vi "AbelFcsMain.vi"() -> ()   [LabVIEW 2011]
uses:
  <vilib>/FPGAPlugInAG/PCIe-7852R/niLvFpga_Open_PCIe-7852R.vi
  <vilib>/rvi/interface/common/dynamic/niFpgaDynamicAddResources.vi
  <vilib>/Utility/error.llb/Error Cluster From Error Code.vi
  <vilib>/FPGAPlugInAG/Dynamic/niLvFpga_Run_Dynamic.vi
  <vilib>/RVI Host/nirviSupport.llb/nirviErrorClusterFromErrorCode.vi
  <vilib>/rvi/errors/niLvFpgaAdjustHostInterfaceError.vi
  <vilib>/DAQmx/create/channels.llb/DAQmx Create Channel (CO-Pulse Generation-Frequency).vi
  <vilib>/FPGAPlugInAG/Dynamic/niLvFpga_Reset_Dynamic.vi
  <vilib>/FPGAPlugInAG/Dynamic/niLvFpga_Close_Dynamic.vi
  <vilib>/rvi/interface/nirviOpenFPGA/nirviOpenFPGA.xnode
  FPGA Bitfiles/AbelFcsProject_FPGATarget_FPGAABELKalman_643775DA.lvbitx
  ABEL-Trap/FPGA_ABEL_Kalman.vi
  <vilib>/rvi/interface/nirviMethod/nirviMethod.xnode
  <vilib>/rvi/interface/nirviCloseFPGA/nirviCloseFPGA.xnode
  <vilib>/FPGAPlugInAG/Dynamic/niLvFpga_ConfigureFifo_Dynamic.vi
  <vilib>/rvi/errors/niLvFpgaMergeErrorWithErrorCode.vi
  <vilib>/FPGAPlugInAG/Dynamic/niLvFpga_StartFifo_Dynamic.vi
  <vilib>/FPGAPlugInAG/Dynamic/niLvFpga_ReadFifo_Dynamic.vi
  <vilib>/Analysis/NI_AALBase.lvlib
  <vilib>/FPGAPlugInAG/Dynamic/niLvFpga_WriteFifo_Dynamic.vi
  <vilib>/rvi/interface/nirviMethod/StockFPGA_InlinedMethodWaitForMultipleIRQ.vi
  <vilib>/FPGAPlugInAG/Dynamic/niLvFpga_WaitOnIrq_Dynamic.vi
  <vilib>/FPGAPlugInAG/Dynamic/niLvFpga_AcknowledgeIrq_Dynamic.vi
panel:
  out "X Steps":dbl
  out "FCS Point Measurement 2":bool
  out "Abeltrapping (EodScan) 2":bool
  out "3dAbelFcs":bool=TRUE
  out "Y Steps":dbl
  out "Z Steps":dbl
  out "concatenated string":string
  out "20Mhz":bool
  out "80Mhz":bool
  in  "Main Control":enum32{"Main", "Trapping"}(tab)
  in  "Stop Program":bool
  in  "SCANNER EMERGENCY":bool
  out "Task":T1(ring)
  in  "Trap":bool
  out "Current Modulation Voltages":dbl[][](array[numeric])
  out "Current Voltages":dbl[][](array[numeric])
  out "Global Stop":bool=TRUE
  out "Stop Measurement":bool
  in  "DeviceTabs":T2(tab)
  in  "WS File Tree":string(tree)
  out "Workspace":path=path "X:/MTusers/Christoph/2011-02-01 Andi/2011-02-01.msw"
  in  "New MSW":bool
  in  "Open MSW":bool
  in  "Sample description":string
  in  "Save Files":bool=TRUE
  out "Last Image File No":i32=-1
  in  "Prefix":string
  in  "Get Position":bool
  in  "Move Stage":bool
  in  "X-Position":dbl=48.0021 caption="X" min=0.0 max=200.0 step=0.1 format="%1.3f um"
  in  "Y-Position":dbl=19.9997 caption="Y" min=0.0 max=200.0 step=0.1 format="%1.3f um"
  in  "Z-Position":dbl=69.999 caption="Z" min=0.0 max=200.0 step=0.1 format="%1.3f um"
  out "x-position":dbl format="%.3f"
  out "y-position":dbl format="%.3f"
  out "z-position":dbl format="%.3f"
  in  "Power Button":bool
  in  "Power":dbl(knob)=100.0 min=0.0 max=100.0 step=5.0 scale=0.0..100.0 scale format="%#_3g"
  out "Laser Connected":bool
  out "Laser ready":bool
  out "Time to go":i32
  in  "Laser  Profile":string="1"
  in  "CFD Settings":T3={"Sync Level"=15, "Sync ZeroX"=0, "Sync Offset"=0, "Chan Settings"=[{"CHx Level"=50, "CHx ZeroX"=10, "CHx Offset"=-22150}, {"CHx Level"=50, "CHx ZeroX"=10, "CHx Offset"=-21850}, {"CHx Level"=75, "CHx ZeroX"=10, "CHx Offset"=-6000}, {"CHx Level"=75, "CHx ZeroX"=10, "CHx Offset"=-5700}]}
  in  "Auto Exposure::Mode":u32(ring) items=["Relative"=0, "Ignored"=5]
  in  "Brightness::Mode":u32(ring) items=["Relative"=0, "Ignored"=5]
  in  "Gain::Mode":u32(ring) items=["Absolute"=1, "Auto"=3, "Relative"=0, "Ignored"=5]
  in  "Gamma::Mode":u32(ring)=2 items=["Relative"=0, "Off"=2, "Ignored"=5]
  in  "Shutter::Mode":u32(ring) items=["Auto"=3, "Relative"=0, "Ignored"=5]
  in  "Trigger::Trigger Activation":u32(ring) items=["Level Low", "Level High"]
  in  "Trigger::Trigger Mode":u32(ring)=16 items=["Mode 0"=0, "Mode 1"=1, "Mode 15"=15, "Off"=16]
  in  "Trigger Delay::Mode":u32(ring)=2 items=["Absolute"=1, "Relative"=0, "Off"=2, "Ignored"=5]
  in  "Brightness::Value":dbl=16.0 min=0.0 max=1023.0 step=1.0
  in  "Shutter::Value":dbl=436.0 min=1.0 max=4095.0 step=1.0
  in  "Auto Exposure::Value":dbl=125.0 min=50.0 max=205.0 step=1.0
  in  "Gain::Value":dbl min=0.0 max=680.0 step=1.0
  in  "Trigger::Trigger Parameter":u32 max=0
  in  "is on?":bool
  out "error out":errorcluster
  in  "PI SystemNumber":i32=1
  in  "Image Measurent Parameters":T4
  in  "Measurement Tab Control":T5(tab)
  in  "Adjustment":bool
  in  "Move into solution":bool=TRUE
  in  "Laser pulse duration":i32[](array[numeric]) min=2 max=100000 step=1 format="%d µs"
  in  "Measurement Time":i32=60 min=10 format="%.0d s"
  in  "Point Measurement":bool
  out "Counts":u32[](array[numeric])
  in  "Line Scan":bool
  in  "Grid Measurement":bool
  in  "Z-Axis Offset":dbl=2.0 min=0.1 max=10.0
  in  "Y-Axis Offset":dbl=2.0 min=0.1 max=10.0
  in  "X-Axis Offset":dbl=2.0 min=0.1 max=10.0
  in  "Z-Axis Points":u16=1 min=1 max=100
  in  "Y-Axis Points":u16=50 min=1 max=100
  in  "X-Axis Points":u16=50 min=1 max=100
  out "Grid Points":dbl[][](array[numeric])
  in  "Axis":enum32{"x-y", "x-z", "y-x", "y-z", "z-x", "z-y"}(ring)
  in  "Picture size 2":dbl=50.0 min=0.1 max=200.0 format="%1.1f um"
  in  "Picture size":dbl=50.0 min=0.1 max=200.0 format="%1.1f um"
  in  "Pixel time":dbl=1.0 min=0.1 max=10.0 step=0.1 format="%.1f ms"
  in  "Resolution":dbl=1.0 min=0.05 max=10.0 step=0.05 format="%.2f µm"
  out "Measure. time":dbl format="%7.1f s"
  in  "Aquire Image":bool
  out "y":i16=500
  out "x":i16=500
  in  "Trapping Tab Control":T6(tab)
  in  "Clear Warnings":bool
  in  "Record":bool
  in  "Estimate Trap Time":bool
  in  "Update FPGA":bool
  in  "Include Mobility Update":bool
  in  "Update Period (ms)":u32=50 min=1
  in  "Time to Show (s)":dbl=10.0 min=1.0
  in  "Threshold (Hz)":dbl=12000.0 min=0.0
  out "Number of Trapping Events":u16
  out "Average Time Trapped (ms)":dbl
  out "x Estimate":dbl
  out "y Estimate":dbl
  out "Time Recorded (s)":dbl
  in  "Time to Record (s)":dbl=-1.0
  out "Current Sub-Bin Delay":u16=112
  in  "New Sub-Bin Delay":u16=112
  out "Current Radius (um)":dbl
  in  "New Radius (um)":dbl min=0.0
  out "Current Scan Frequency (Hz)":dbl
  in  "New Scan Frequency (Hz)":dbl
  out "Current Spacing (um)":dbl
  out "Current Scan Form":enum8{"Circular", "Square", "Hexagonal"}(ring)
  in  "New Spacing (um)":dbl=0.75 min=0.0
  in  "New Number of Points per Scan":u8=27 min=3 max=32
  out "Current Number of Points per Scan":u8=1
  in  "New Scan Form":T7(ring)
  out "Current EOD Deflection Scale (um/V)":dbl
  in  "New EOD Deflection Scale (um/V)":dbl=0.21 min=0.0
  out "Current Beam Waist Estimate (um)":dbl
  in  "New Beam Waist Estimate (um)":dbl=0.36 min=0.0
  out "Current Maximum Feedback (V)":dbl
  out "Current Mobility Estimate (um/s/V)":dbl
  in  "New Mobility Estimate (um/s/V)":dbl
  out "Current Diffusion Constant Estimate (um^2/s)":dbl
  in  "New Diffusion Constant Estimate (um^2/s)":dbl min=0.0
  in  "New Maximum Feedback (V)":dbl=10.0 min=0.0 max=10.0
  out "Current Modulation Angle (degrees)":dbl
  in  "New Modulation Angle (degrees)":dbl min=0.0 max=360.0
  out "Current Number of Modulation Points":u8=1
  in  "New Number of Modulation Points":u8=1 min=1 max=16
  in  "New Modulation Radius (um)":dbl min=0.0
  out "Current Modulation Radius (um)":dbl
  in  "New Modulation Frequency (Hz)":dbl min=0.0
  out "Current Modulation Frequency (Hz)":dbl
  out "Z in":dbl
  out "Z out":dbl
  out "X in":dbl
  in  "How long?":bool
  out "Estimated Time (h)":dbl
  in  "Mesaurement Time (Sec) / Step":dbl
  in  "Start 3D FCS Abel Scan":bool
  in  "Abeltrapping (EodScan)":bool
  in  "FCS Point Measurement":bool
  in  "Z Stepsize":dbl
  in  "Y Stepsize":dbl
  in  "X Stepsize":dbl
  in  "Z End":dbl
  in  "Y End":dbl
  in  "X End":dbl
  in  "Z Start":dbl
  in  "Y Start":dbl
  in  "X Start":dbl
  out "X out":dbl
  out "Y in":dbl
  out "Y out":dbl
  out "Active pt3":path
  in  "ShowTab":T8(tab)=enum."TCSPC Histogram"
  out "acquired FPS":dbl
  out "Image Out":T9(plugin-control)
  out "Image Number":u32
  in  "Find Mols":bool
  out "Image":i32[][](graph)
  in  "Save Color Image":bool
  in  "Auto Shutter Control":bool=TRUE
  in  "Auto Meas":bool
  in  "Auto Measurement Time (ms)":i32=60 caption="Measurement Time (s)" min=10
  in  "Autopoint-Auto Z":bool
  out "Histogram":i32[][](graph)
  out "Trace":i32[][](graph)=[[2, 0, 0, 1, 1, 1, 0, 0, 0, 1, 0, 1, 0, 1, 2, 2, 0, 3, 0, 2, 2, 1, 3, 1, 0, 1, 1, 1, 0, 1, 3, 1, 0, 2, 0, 1, 0, 1, 1, 0, 1, 1, 3, 1, 0, 2, 0, 1, 1, 0, 0, 2, 0, 0, 1, 1, 1, 0, 0, 1, 0, 1, 0, 0, 0, 1, 2, 1, 1, 2, 0, 2, 4, 3, 1, 1, 0, 0, 1, 1, 2, 0, 1, 1, 0, 0, 0, 1, 1, 1, 1, 3, 0, 0, 1, 0, 0, 0, 2, 1, 1, 1, 2, 1, 0, 1, 1, 0, 0, 2, 1, 1, 0, 0, 1, 1, 1, 1, 0, 2, 2, 0, 1, 2, 1, 0, 3, 0, 2, 1, 3, 0, 1, 1, 0, 0, 3, 0, 0, 0, 0, 0, 0, 0, 0, 0, 0, 0, 0, 0, 0, 0, 0, 0, 0, 0, 0, 0, 0, 0, 0, 0, 0, 0, 0, 0, 0, 0, 0, 0, 0, 0, 0, 0, 0, 0, 0, 0, 0, 0, 0, 0, 0, 0, 0, 0, 0, 0, 0, 0, 0, 0, 0, 0, 0, 0, 0, 0, 0, 0], [1, 2, 2, 0, 0, 0, 1, 2, 1, 2, 1, 1, 1, 0, 0, 0, 3, 1, 0, 1, 0, 2, 0, 2, 1, 1, 0, 0, 1, 0, 1, 2, 1, 0, 0, 0, 0, 0, 1, 0, 1, 0, 2, 0, 1, 0, 0, 0, 0, 1, 1, 3, 0, 0, 0, 2, 0, 0, 2, 0, 1, 1, 0, 0, 2, 0, 2, 1, 0, 1, 1, 0, 1, 1, 0, 0, 0, 1, 0, 0, 1, 0, 0, 0, 0, 1, 0, 1, 1, 1, 1, 0, 0, 0, 1, 1, 1, 0, 1, 0, 0, 0, 1, 1, 1, 0, 0, 1, 1, 3, 1, 0, 0, 0, 0, 0, 0, 0, 1, 2, 1, 0, 0, 0, 2, 3, 3, 2, 0, 1, 1, 1, 0, 0, 4, 0, 1, 2, 0, 0, 0, 2, 0, 0, 0, 0, 0, 0, 0, 0, 0, 0, 0, 0, 0, 0, 0, 0, 0, 0, 0, 0, 0, 0, 0, 0, 0, 0, 0, 0, 0, 0, 0, 0, 0, 0, 0, 0, 0, 0, 0, 0, 0, 0, 0, 0, 0, 0, 0, 0, 0, 0, 0, 0, 0, 0, 0, 0, 0, 0], [2, 2, 0, 1, 2, 0, 1, 0, 2, 3, 1, 0, 1, 0, 1, 0, 0, 0, 0, 2, 1, 0, 0, 2, 2, 0, 0, 0, 3, 0, 0, 2, 2, 2, 0, 3, 0, 3, 1, 3, 1, 3, 1, 0, 3, 1, 3, 3, 1, 1, 1, 1, 2, 0, 1, 0, 1, 1, 1, 3, 0, 2, 3, 1, 1, 1, 0, 1, 0, 1, 2, 3, 1, 2, 1, 3, 0, 2, 0, 2, 0, 1, 0, 2, 2, 1, 1, 3, 1, 2, 1, 1, 1, 3, 0, 0, 0, 0, 1, 1, 1, 0, 1, 0, 2, 1, 1, 0, 1, 0, 1, 2, 2, 2, 2, 0, 1, 0, 0, 0, 1, 1, 2, 0, 0, 1, 5, 2, 2, 0, 2, 0, 2, 2, 2, 0, 1, 0, 6, 0, 0, 0, 0, 0, 0, 0, 0, 0, 0, 0, 0, 0, 0, 0, 0, 0, 0, 0, 0, 0, 0, 0, 0, 0, 0, 0, 0, 0, 0, 0, 0, 0, 0, 0, 0, 0, 0, 0, 0, 0, 0, 0, 0, 0, 0, 0, 0, 0, 0, 0, 0, 0, 0, 0, 0, 0, 0, 0, 0, 0], [0, 0, 1, 0, 1, 1, 0, 0, 0, 1, 1, 0, 1, 0, 0, 0, 0, 0, 2, 0, 0, 0, 0, 2, 0, 0, 0, 1, 1, 2, 1, 1, 1, 2, 1, 0, 0, 3, 0, 1, 1, 0, 0, 0, 0, 1, 0, 0, 2, 1, 0, 0, 1, 1, 1, 2, 2, 0, 1, 0, 0, 1, 0, 1, 1, 0, 0, 2, 1, 1, 2, 1, 1, 0, 0, 0, 0, 2, 1, 0, 0, 0, 0, 1, 0, 1, 0, 0, 0, 0, 1, 0, 0, 0, 0, 1, 0, 1, 1, 1, 0, 2, 3, 1, 1, 0, 1, 1, 1, 0, 1, 0, 0, 1, 1, 0, 2, 0, 0, 0, 0, 3, 0, 0, 0, 0, 0, 0, 0, 0, 1, 0, 2, 0, 0, 0, 1, 2, 2, 0, 1, 0, 0, 0, 0, 0, 0, 0, 0, 0, 0, 0, 0, 0, 0, 0, 0, 0, 0, 0, 0, 0, 0, 0, 0, 0, 0, 0, 0, 0, 0, 0, 0, 0, 0, 0, 0, 0, 0, 0, 0, 0, 0, 0, 0, 0, 0, 0, 0, 0, 0, 0, 0, 0, 0, 0, 0, 0, 0, 0]]
  out "Laser Temperature":dbl[](graph)
  out "Amplifier":i32[](graph)
  out "Preamplifier":i32(knob) scale=0.0..4500.0
  out "Backreflection":i32(knob) scale=0.0..500.0
  out "Power set":dbl(knob) scale=0.0..100.0 scale format="%#_3g"
  out "Photodiode":i32(knob) scale=0.0..20.0 scale format="%-3.0f"
  out "Recent Photon Count Rate":cluster{dbl[], dbl[]}(graph)
  out "Position Plot":T10(graph)
  out "On-Chip FIFO Overflow":bool
  out "Feedback DMA Overflow":bool
  out "Photon DMA Overflow":bool
  out "Unrecognized Command":bool
  out "Mistimed":bool
  out "Ready":bool
  out "Currently Trapped":bool
  out "Feedback":dbl(slide) scale=0.0..1.0
  out "Photon":dbl(slide) scale=0.0..1.0
  out "Buffer Overrun":bool
  out "Running":bool
  # "Scanner Position"
  # "Point Measurement Settings"
  # "Line Scan Settings"
  # "Starting Point"
  # "Grid Measurement Settings"
  # "Starting Point"
  # "um"
  # "um"
  # "um"
  # "Image Scan Settings"
  # "Pixel"
  # "Debug:In/out x,y,z"
  # "Auto Measurement Settings"
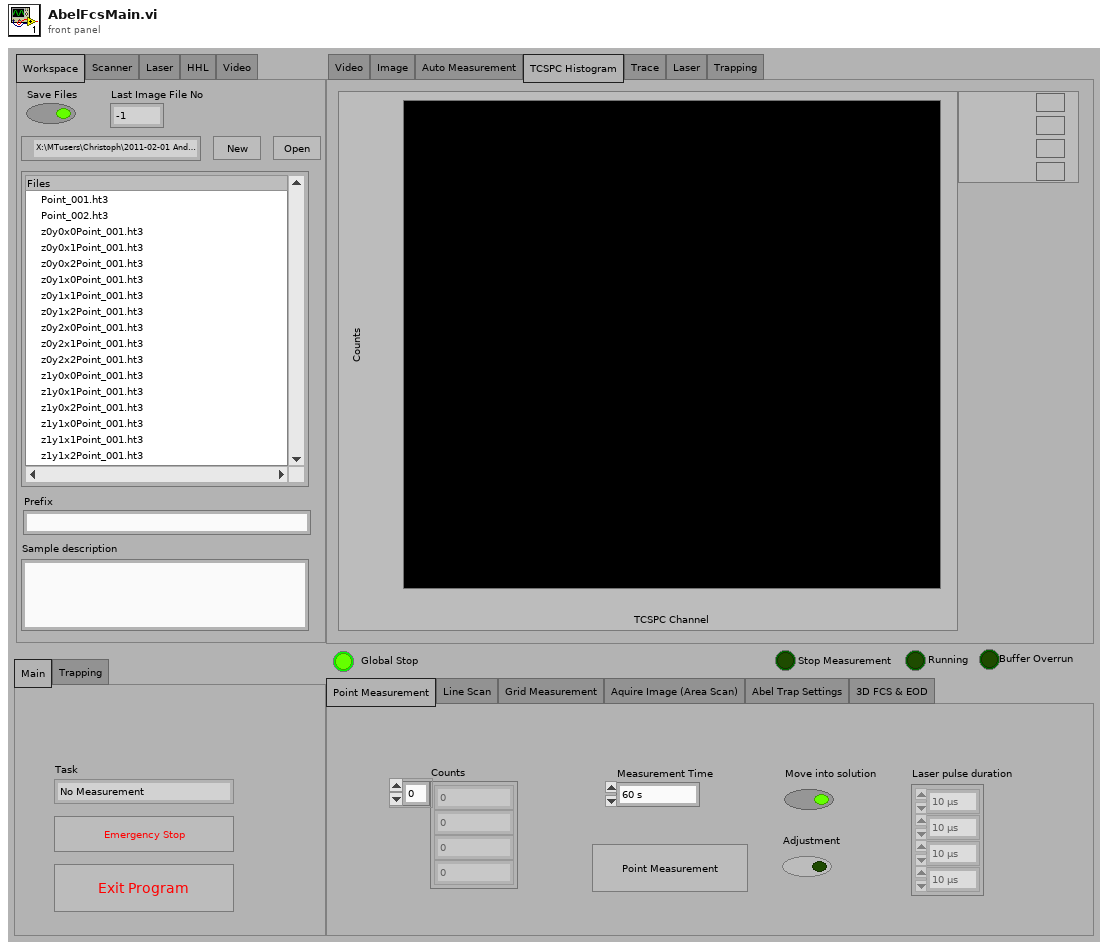
[diagram p1: front panel]
types:
  T1 = enum16{"No Measurement", "Aquire Image", "Point Measurement", "Multi Measurement", "Save Color Image", "Find Single Mol.", "Auto Measurement Control", "Auto Point", "Aquire Line Scan", "Grid Measurement", "Trapping", "Move Scanner"}
  T2 = enum32{"Workspace", "Scanner", "Laser", "HHL", "Video"}
  T3 = cluster{"Sync Level":i32, "Sync ZeroX":i32, "Sync Offset":i32, "Chan Settings":cluster{"CHx Level":i32, "CHx ZeroX":i32, "CHx Offset":i32}[]}
  T4 = cluster{"Position":cluster{"X-Position":dbl, "Y-Position":dbl, "Z-Position":dbl}, "Axis 1 Pixels":dbl, "Axis 2 Pixels":dbl, "Axis":i32, "Resolution":dbl, "PixelTime":dbl, "Laser pulses":i32}
  T5 = enum32{"Point Measurement", "Line Scan", "Grid Measurement", "Aquire Image (Area Scan)", "Abel Trap Settings", "3D FCS & EOD"}
  T6 = enum32{"Main", "Scan Parameters", "Beam Parameters", "Trap Parameters", "modulation Parameters"}
  T7 = enum8{"Circular", "Square", "Hexagonal", "FilledSquare"}
  T8 = enum32{"Video", "Image", "Auto Measurement", "TCSPC Histogram", "Trace", "Laser", "Trapping"}
  T9 = typedef "IMAQ Image.ctl" = refnum<image>
  T10 = cluster{"X coordinates":dbl[], "Y coordinates":dbl[]}[]
  T11 = cluster{"Dev":i32, "SerNo":string, "HW_Model":string, "HW_Partno":string}[]
  T12 = enum16{"No Measurement", "Aquire Image", "Point Measurement", "Multi Measurement", "Save Color Image"}
  T13 = enum16{"No Measurement", "Aquire Image", "Point Measurement", "Multi Measurement", "Save Color Image", "Find Single Mol.", "Auto Measurement Control", "Auto Point", "Aquire Line Scan"}
  T14 = enum16{"No Measurement", "Aquire Image", "Point Measurement", "Multi Measurement", "Save Color Image", "Find Single Mol.", "Auto Measurement Control", "Auto Point", "Aquire Line Scan", "Grid Measurement"}
  T15 = enum16{"No Measurement", "Aquire Image", "Point Measurement", "Multi Measurement", "Save Color Image", "Find Single Mol.", "Auto Measurement Control", "Auto Point"}
  T16 = enum16{"No Measurement", "Aquire Image", "Point Measurement", "Multi Measurement", "Save Color Image", "Find Single Mol."}
  T17 = enum16{"Get (Default)", "Set Workspace", "Append File", "Change Comment"}
  T18 = enum16{"unknown", "pt3 File", "png Image", "bmp Image"}
  T19 = cluster{"File No":i32, "File Path":path, "Parent File":i32, "File Type":enum16{"unknown", "pt3 File", "png Image", "bmp Image"}, "Measurement Type":enum16{"not a pt3 File", "Image File", "Point Measurement", "Auto Point", "Line Scan", "Grid Scan"}, "Upper Left":cluster{"x-Position":dbl, "y-Position":dbl, "z-Position":dbl}, "Pixels":dbl[], "Resolution":dbl, "Scan Axis":enum32{"x-y", "x-z", "y-x", "y-z", "z-x", "z-y"}, "PixelTime":dbl}[]
  T20 = cluster{"File No":i32, "File Path":path, "Parent File":i32, "File Type":enum16{"unknown", "pt3 File", "png Image", "bmp Image"}, "Measurement Type":enum16{"not a pt3 File", "Image File", "Point Measurement", "Auto Point", "Line Scan", "Grid Scan"}, "Upper Left":cluster{"x-Position":dbl, "y-Position":dbl, "z-Position":dbl}, "Pixels":i32[], "Scan Axis":enum32{"x-y", "x-z", "y-x", "y-z", "z-x", "z-y"}, "Resolution":dbl, "PixelTime":dbl}[]
  T21 = cluster{"File No":i32, "File Path":path, "Parent File":i32, "File Type":enum16{"unknown", "pt3 File", "png Image", "bmp Image"}, "Measurement Type":enum16{"not a pt3 File", "Image File", "Point Measurement", "Auto Point", "Line Scan", "Grid Scan"}, "Upper Left":cluster{"x-Position":dbl, "y-Position":dbl, "z-Position":dbl}, "Pixels":i32[], "Resolution":dbl, "Scan Axis":enum32{"x-y", "x-z", "y-z"}, "PixelTime":dbl}[]
  T22 = typedef "LVPoint32TypeDef.ctl" = cluster{"Horizontal":i32, "Vertical":i32}
  T23 = cluster{"Shift":bool, "Ctrl":bool, "Alt":bool, "Cmd":bool, "Opt":bool}
  T24 = cluster{"File No":i32, "File Path":path, "Parent File":i32, "File Type":enum16{"unknown", "pt3 File", "png Image", "bmp Image"}, "Measurement Type":enum16{"not a pt3 File", "Image File", "Point Measurement", "Auto Point", "Line Scan", "Grid Scan"}, "Upper Left":cluster{"x-Position":dbl, "y-Position":dbl, "z-Position":dbl}, "Pixels":i32[], "Scan Axis":enum32{"x-y", "x-z", "y-z"}, "Resolution":dbl, "PixelTime":dbl}
  T25 = enum16{"not a pt3 File", "Image File", "Point Measurement", "Auto Point", "Line Scan", "Grid Scan"}
  T26 = cluster{"Ident":string, "Format Version":string, "Creator Name":string, "Creator Version":string, "File Time":string, "Comment":string, "Laser":i32, "Binning":i32, "Offset":i32, "AcquisitionTime (ms)":i32, "HardwareSerial":i32, "SyncDivider":i32, "Resolution (ps)":dbl, "Rates":dbl[], "SyncRate":dbl, "CFD Settings":cluster{"Sync Level":i32, "Sync ZeroX":i32, "Sync Offset":i32, "Chan Settings":cluster{"CHx Level":i32, "CHx ZeroX":i32, "CHx Offset":i32}[]}}
  T27 = cluster{"Dimensions":i32, "Time Per Pixel [ms]":dbl, "Acceleration":i32, "Pattern":i32, "X0":sgl, "Y0":sgl, "Z0":dbl, "PixX":i32, "PixY":i32, "PixResol":sgl, "TStartTo":sgl, "TStoptTo":sgl, "TStartFro":sgl, "TStopFro":sgl}
  T28 = cluster{cluster{"X0":sgl, "Y0":sgl, "Z0":dbl}, "PixX":i32, "PixY":i32, "Pattern":i32, "PixResol":sgl, "Time Per Pixel [ms]":dbl, "Laser":i32}
  T29 = enum8{"Enabled", "Disabled", "Disabled and Grayed Out"}
  T30 = cluster{"Photon File":refnum<file>, "Feedback File":refnum<file>}
  T31 = enum16{"big-endian, network order", "native, host order", "little-endian"}
  T32 = enum16{"open", "replace", "create", "open or create", "replace or create", "replace or create with confirmation"}
  T33 = cluster{"X coordinates":dbl[], "Y coordinates":dbl[]}
  T34 = cluster{"refnum out":refnum<file>, "refnum out":refnum<file>}
  T35 = enum16{"none", "fast axis", "slow axis", "both axis", ""}
  T36 = enum16{"none", "fast axis", "slow axis", "both", ""}
  T37 = enum16{"target position", "relative position", "actual position", "position error"}
  T38 = enum16{"not a pt3 File", "Image File", "Point Measurement", "Auto Point"}
  T39 = enum16{"not a pt3 File", "Image File", "Point Measurement", "Auto Point", "Line Scan"}
  T40 = cluster{"Dev":i32, "SerNo":string, "HW_Model":string, "HW_Partno":string}
  T41 = cluster{"Comment":string, "Binning":i32, "Offset":i32, "AcquisitionTime (ms)":i32, "HardwareSerial":i32, "SyncDivider":i32, "Resolution (ps)":dbl, "CFD Settings":cluster{"Sync Level":i32, "Sync ZeroX":i32, "Sync Offset":i32, "Chan Settings":cluster{"CHx Level":i32, "CHx ZeroX":i32, "CHx Offset":i32}[]}, "ModuleInfo":cluster{"modelcode":i32, "versioncode":i32}[], "BaseResolution (ps)":dbl, "RefClockSource":i32, "ChanInfo":cluster{"CHx Level":i32, "CHx ZeroX":i32, "CHx Offset":i32, "CHx modidx":i32}[], "SyncRate":i32, "InputsEnabled":i64}
  T42 = cluster{"InpRateFilePos":i64, "StopAfterFilePos":i64}
  T43 = cluster{"X-Position":dbl, "Y-Position":dbl, "Z-Position":dbl}
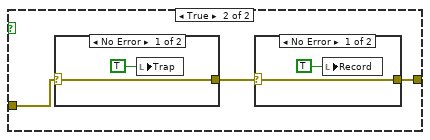
[diagram p3: hidden frame]
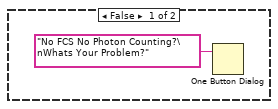
[diagram p7: hidden frame]
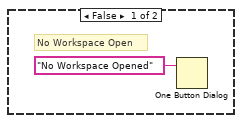
[diagram p8: hidden frame]
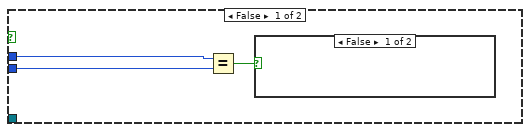
[diagram p9: hidden frame]
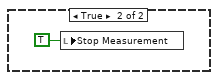
[diagram p10: hidden frame]
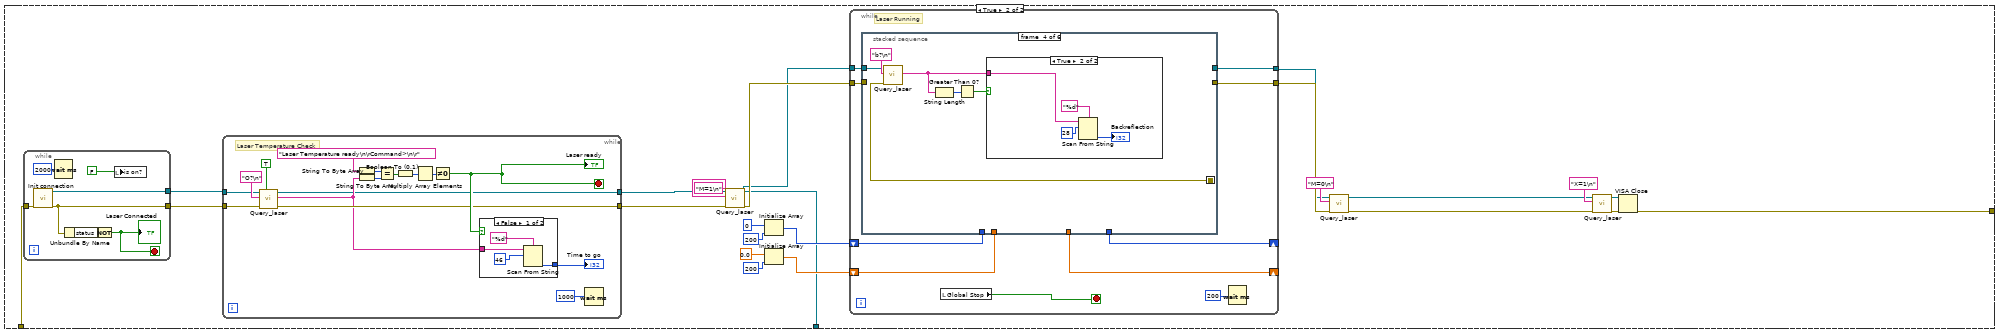
[diagram p11: hidden frame]
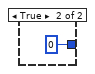
[diagram p12: hidden frame]
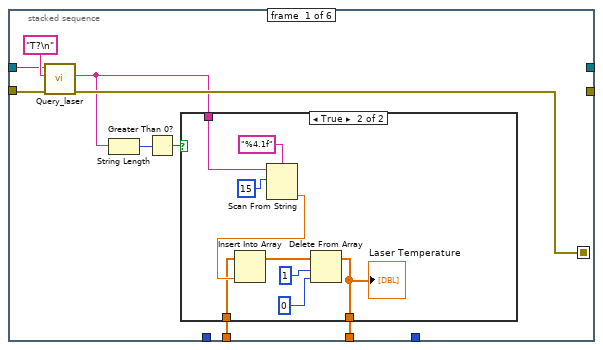
[diagram p13: hidden frame]
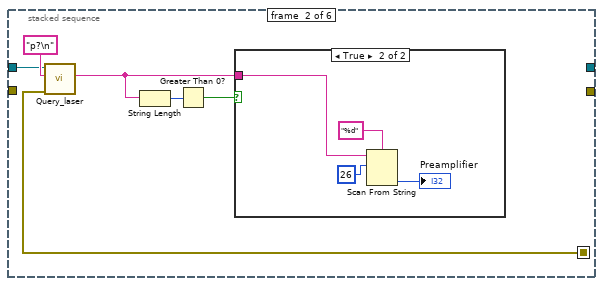
[diagram p15: hidden frame]
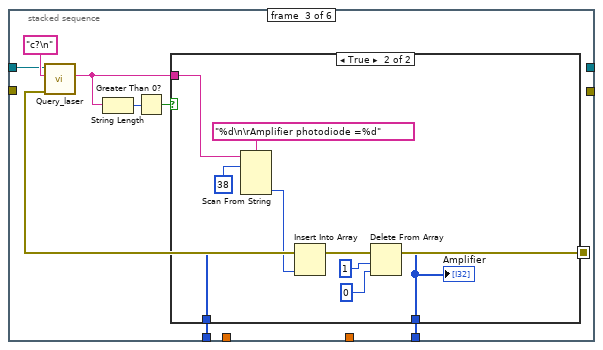
[diagram p17: hidden frame]
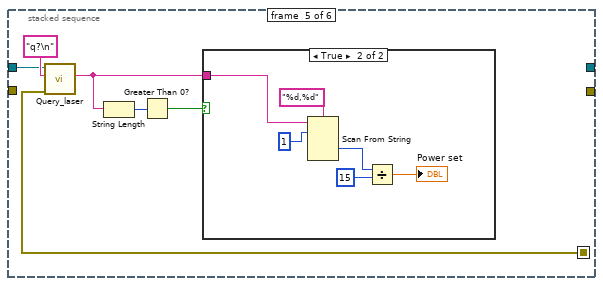
[diagram p20: hidden frame]
diagram:
  w11 = i8 4  # Variance Scale
  w18 = 41.0  # Shortest Bin Length (ticks)
  w20 = 40000000.0  # Clock Speed
  w21 = u8 32  # Maximum Allowed Points
  # "Command Interpreter\nValue in 8 MSBs sets the command\n[Bracketed commands are deprecated]\n0, dflt - unrecognized\n1 - Go/Stop (T/F) (value in 16 LSBs)\n[2 - Acquire/stop acquiring (T/F) (value in 16 LSBs)]\n4 - Mobility Update? (value in 16 LSBs)\n5 - Inverse Diffusion Constant (value in 24 LSBs)\n6 - Inverse Mobility (value in 24 LSBs)\n7 - Saturated Position Step (value in 24 LSBs)\n8 - Bin Length in ticks (value in 24 LSBs)\n9 - Bins per Cycle (value in 8 LSBs)\n[10 - Bin Delay (T/F) (value in 16 LSBs)]\n11 - Sub-Bin Delay in ticks (value in 16 LSBs)\n12 - Cycles per Modulation (value in 24 LSBs)\n13 - Number of Modulation Points (value in 8 LSBs)\n16 - EOD Voltage (x) (value in 16 LSBs, address in bits 16-23)\n17 - EOD Voltage (y) (value in 16 LSBs, address in bits 16-23)\n[18 - Feedback Voltage (x) (value in 16 LSBs, address in bits 16-23)]\n[19 - Feedback Voltage (y) (value in 16 LSBs, address in bits 16-23)]\n20 - Modulation (x) (value in 16 LSBs, address in bits 16-23)\n21 - Modulation (y) (value in 16 LSBs, address in bits 16-23)"
  # "Maximum Voltage"
  # "Global Constants"
  n1 = control-ref of="ShowTab"() -> (w1:refnum<vi>)
  n2 = local read "20Mhz"() -> (w6:bool)
  n3 = flat-sequence {
    tunnel: [w63] -> w35
    tunnel: errorcluster {"status"=FALSE, "code"=0, "source"=""} ("error in") -> [w51]
    frame #0 {
      w56 = path ""
      w66 = FALSE ("Global Stop")
      n4 = local write "Last Image File No"(-1 ("Last Image File No")) -> ()
      n5 = property on="Aquire Image" class="Bool"("BoolText.Text"="Aquire Image" ("Caption.Text"), "BoolText.TextColor"=u32 0 ("Boolean Text.Colors:FG Color")) -> ()  [unwired: 2 in, 2 out]
      n6 = property on="Line Scan" class="Bool"("BoolText.Text"="Start Line Scan" ("Caption.Text"), "BoolText.TextColor"=u32 0 ("Boolean Text.Colors:FG Color")) -> ()  [unwired: 2 in, 2 out]
      n7 = control-ref of="WS File Tree"() -> (w65:refnum<vi>)
      n8 = control-ref of="ShowTab"() -> (w48:refnum<vi>)
      n9 = property on="Point Measurement" class="Bool"("BoolText.Text"="Point Measurement" ("Caption.Text"), "BoolText.TextColor"=u32 0 ("Boolean Text.Colors:FG Color")) -> ()  [unwired: 2 in, 2 out]
      n10 = property on="Grid Measurement" class="Bool"("BoolText.Text"="Grid Measurement" ("Caption.Text"), "BoolText.TextColor"=u32 0 ("Boolean Text.Colors:FG Color")) -> ()  [unwired: 2 in, 2 out]
      n11 = local write "PI SystemNumber"("PI SystemNumber") -> ()
      n12 = call "MTS_ClearWSTree2.vi"("error in"=w51, "Tree Refnum"=w65) -> ("error out"=w64:errorcluster)  [unwired: 8 in, 1 out]
      n13 = call "MTS_ShowHideTabs.vi"("Action"=enum16{"Show All", "Hide Tab", "Show Tab"}."Show All", "error in (no error)"=w64, "ShowTab"=w48) -> ("error out"=w63:errorcluster)  [unwired: 7 in, 1 out]
      "Global Stop" <- w66
      "Running" <- w66
      "Buffer Overrun" <- w66
      "Stop Measurement" <- w66
      "Workspace" <- w56
      "Active pt3" <- w56
      "Task" <- T1."No Measurement" ("Do Measurement")
    }
  }
  n14 = flat-sequence {
    tunnel: [w74] -> w45
    tunnel: w35 -> [w69]
    tunnel: [w67] -> w5
    frame #0 {
      n15 = local read "PI SystemNumber"() -> (w68:i32)
      n16 = call "InitScanner.vi"("error in (no error)"=w69, "PI SystemNumber"=w68) -> ("error out"=w73:errorcluster, "z-position"=w71:dbl, "y-position"=w70:dbl, "x-position"=w72:dbl)  [unwired: 6 in]
      n17 = local write "X-Position"(w72) -> ()
      n18 = local write "Y-Position"(w70) -> ()
      n19 = local write "Z-Position"(w71) -> ()
      n20 = call "HH_Init.vi"("error in (no error)"=w73) -> ("Device List"=w74:T11, "error out"=w67:errorcluster)  [unwired: 12 in, 1 out]
    }
  }
  n21 = call "Prompt User for Input"("error in (no error)"=w5) -> ("20Mhz"=→"20Mhz":bool, "80Mhz"=→"80Mhz":bool, "error out"=w2:errorcluster)  [unwired: 15 in, 1 out]
  n22 = while {
    tunnel: w2 -> [w78]
    tunnel: [w76] -> _
    tunnel: w1 -> [w75]
    stop <- w80 stop-if-true
    n23 = property on="3dAbelFcs" class="Bool (strict)"(error in=w78) -> (error out=w77:errorcluster, "Value"=w79:bool)  [unwired: 1 in, 1 out]
    n24 = case shown="True" w79 {
      tunnel: w77 -> [_ w89]
      tunnel: [_ w86] -> w76
      tunnel: w75 -> [_ w82]
      frame False {
      }
      frame True {
        n25 = local read "X Stepsize"() -> (w85:dbl)
        n26 = local read "Y Stepsize"() -> (w84:dbl)
        n27 = local read "Z Stepsize"() -> (w83:dbl)
        n28 = local read "Z Steps"() -> (w81:dbl)
        n29 = for {
          N: w81 -> [_]
          tunnel: w82 -> [w101]
          tunnel: w89 -> [w94]
          tunnel: w83 -> [w100]
          tunnel: w84 -> [w99]
          tunnel: w85 -> [w98]
          tunnel: [w97] -> w88
          i -> [w96]
          n30 = local read "Z Start"() -> (w91:dbl)
          n31 = local read "Y Steps"() -> (w93:dbl)
          n32 = Multiply(x=w100, y=w96) -> (x*y=w92:dbl)
          n33 = Number To Decimal String(number=w96) -> (decimal integer string=w95:string)  [unwired: 1 in]
          n34 = Add(x=w91, y=w92) -> (x+y=w90:dbl)
          "Z in" <- w90
          n35 = for {
            N: w93 -> [_]
            tunnel: w101 -> [w113]
            tunnel: w99 -> [w112]
            tunnel: w98 -> [w111]
            tunnel: w94 -> [w106]
            tunnel: [w110] -> w97
            tunnel: w95 -> [w108]
            i -> [w109]
            n36 = local read "Y Start"() -> (w103:dbl)
            n37 = local read "X Steps"() -> (w105:dbl)
            n38 = Multiply(x=w112, y=w109) -> (x*y=w104:dbl)
            n39 = Add(x=w103, y=w104) -> (x+y=w102:dbl)
            "Y in" <- w102
            n40 = Number To Decimal String(number=w109) -> (decimal integer string=w107:string)  [unwired: 1 in]
            n41 = for {
              N: w105 -> [_]
              tunnel: w113 -> [w133]
              tunnel: w106 -> [w115]
              tunnel: w111 -> [w131]
              tunnel: [w123] -> w110
              tunnel: w108 -> [w128]
              tunnel: w107 -> [w126]
              i -> [w130]
              n42 = local read "FCS Point Measurement"() -> (w120:bool)
              n43 = Multiply(x=w131, y=w130) -> (x*y=w118:dbl)
              n44 = case shown="True" w120 {
                tunnel: w133 -> [_ w155]
                tunnel: [_ w154] -> w132
                tunnel: w115 -> [_ w152]
                frame False {
                  n45 = One Button Dialog(message="No FCS No Photon Counting?\nWhats Your Problem?") -> ()  [unwired: 1 in, 1 out]
                }
                frame True {
                  n46 = local read "Workspace"() -> (w153:path)
                  n47 = local read "Running"() -> (w161:bool)
                  n48 = Not(x=w161) -> (.not. x?=w156:bool)
                  n49 = Not Equal?(x=w153, y=path "") -> (x != y?=w157:bool)
                  n50 = local read "Task"() -> (w160:T1)
                  n51 = case shown="True" w157 {
                    tunnel: w156 -> [_ w168]
                    tunnel: T12."Point Measurement" ("Do Measurement") -> [_ w167]
                    tunnel: w160 -> [_ w166]
                    tunnel: w155 -> [_ w165]
                    tunnel: [_ w164] -> w154
                    tunnel: w152 -> [_ w163]
                    frame False {
                      # "No Workspace Open"
                      n52 = One Button Dialog(message="No Workspace Opened") -> ()  [unwired: 1 in, 1 out]
                    }
                    frame True {
                      # "Aquire Image if not Running"
                      n53 = case shown="True" w168 {
                        tunnel: w167 -> [w170 w183]
                        tunnel: w166 -> [w171 _]
                        tunnel: w165 -> [_ w175]
                        tunnel: [_ w173] -> w164
                        tunnel: w163 -> [_ w173]
                        frame False {
                          n54 = Equal?(x=w171, y=w170) -> (x = y?=w169:bool)
                          n55 = case shown="False" w169 {
                            frame False {
                            }
                            frame True {
                              n56 = local write "Stop Measurement"(TRUE ("Stop Measurement")) -> ()
                            }
                          }
                        }
                        frame True {
                          w176 = enum16{"Show All", "Hide Tab", "Show Tab"}."Hide Tab" ("Action")
                          n57 = local write "Task"(w183) -> ()
                          n58 = local write "Running"(TRUE ("Measurement Running")) -> ()
                          n59 = control-ref of="Point Measurement"() -> (w174:refnum<vi>)
                          n60 = call "MTS_ShowHideTabs.vi"("Action"=w176, "Tab Caption"="Video", "ShowTab"=w175) -> ("ShowTab out"=w179:refnum<vi>)  [unwired: 7 in, 1 out]
                          n61 = property on="Property Node" class="Bool"(reference=w174, "BoolText.Text"="Stop Aquire" ("Caption.Text"), "BoolText.TextColor"=u32 16711680 ("Boolean Text.Colors:FG Color")) -> ()  [unwired: 1 in, 2 out]
                          n62 = call "MTS_ShowHideTabs.vi"("Action"=w176, "Tab Caption"="Image", "ShowTab"=w179) -> ("ShowTab out"=w177:refnum<vi>)  [unwired: 7 in, 1 out]
                          n63 = call "MTS_ShowHideTabs.vi"("Action"=w176, "Tab Caption"="Auto Measurement", "ShowTab"=w177) -> ()  [unwired: 7 in, 2 out]
                        }
                      }
                    }
                  }
                }
              }
              n64 = Number To Decimal String(number=w130) -> (decimal integer string=w124:string)  [unwired: 1 in]
              n65 = local read "X Start"() -> (w117:dbl)
              n66 = Add(x=w117, y=w118) -> (x+y=w116:dbl)
              "X in" <- w116
              n67 = Concatenate Strings("z" ("string"), w128, "y" ("string"), w126, "x" ("string"), w124) -> (→"concatenated string":string)
              n68 = local write "X-Position"(w116) -> ()
              n69 = local read "Abeltrapping (EodScan)"() -> (w119:bool)
              n70 = case shown="False" w119 {
                tunnel: [w134 w136] -> w122
                tunnel: w115 -> [w134 w135]
                frame False {
                }
                frame True {
                  n71 = case shown="No Error" w135 {
                    selector: w135 -> [w141 _]
                    tunnel: [w141 _] -> w137
                    frame No Error {
                      n72 = local write "Trap"(TRUE ("Trap")) -> ()
                    }
                    frame Error {
                    }
                  }
                  n73 = case shown="No Error" w137 {
                    selector: w137 -> [w139 _]
                    tunnel: [w139 _] -> w136
                    frame No Error {
                      n74 = local write "Record"(TRUE ("Record")) -> ()
                    }
                    frame Error {
                    }
                  }
                }
              }
              n75 = while {
                tunnel: w132 -> [w148]
                tunnel: w122 -> [w147]
                tunnel: [w146] -> w114
                stop <- w150 continue-if-true
                n76 = Merge Errors(w148, w147) -> (w146:errorcluster)
                n77 = local read "Running"() -> (w150:bool)
                n78 = Wait (ms)(milliseconds to wait=u32 100) -> ()  [unwired: 1 out]
              }
              n79 = case shown="No Error" w114 {
                selector: w114 -> [w143 w145]
                tunnel: [w144 w145] -> w123
                frame No Error {
                  w142 = FALSE ("Value (Signaling)")
                  n80 = local write "Trap"(w142) -> ()
                  n81 = local write "Record"(w142) -> ()
                  n82 = property on="Trap" class="Bool (strict)"(error in=w143, "Val(Sgnl)"=w142) -> (error out=w144:errorcluster)  [unwired: 1 in, 1 out]
                }
                frame Error {
                }
              }
            }
            n83 = local write "Y-Position"(w102) -> ()
          }
          n84 = local write "Z-Position"(w90) -> ()
        }
        n85 = property on="3dAbelFcs" class="Bool (strict)"(error in=w88, "Value"=FALSE ("3dAbelFcs")) -> (error out=w86:errorcluster)  [unwired: 1 in, 1 out]
      }
    }
    n86 = local read "Global Stop"() -> (w80:bool)
  }
  n87 = case shown="False" w6 {
    tunnel: [_ w189] -> w34
    tunnel: [w186 w188] -> w33
    tunnel: w2 -> [w186 w187]
    frame False {
    }
    frame True {
      n88 = while {
        tunnel: [w235] -> w206
        tunnel: [w234] -> w207
        tunnel: w187 -> [w231]
        stop <- w233 stop-if-true
        n89 = call "Init connection.vi"("error in"=w231) -> ("error constant"=w235:errorcluster, "VISA resource name 2"=w234:refnum<visa-resource-name>)  [unwired: 9 in]
        n90 = Wait (ms)(milliseconds to wait=2000) -> ()  [unwired: 1 out]
        n91 = Unbundle By Name(w235) -> ("status"=w236:bool)
        n92 = Not(x=w236) -> (.not. x?=w233:bool)
        "Laser Connected" <- w233
        n93 = local write "is on?"(FALSE) -> ()
      }
      n94 = while {
        tunnel: w207 -> [w223]
        tunnel: w206 -> [w222]
        tunnel: [w211] -> w189
        tunnel: [w213] -> w209
        stop <- w215 stop-if-true
        # "Laser Temperature Check"
        n95 = call "Query_laser.vi"("Reset?"=TRUE, "error in (no error)"=w222, "String in"="O?\n", "VISA resource name"=w223) -> ("error out"=w213:errorcluster, "String out"=w212:string, "VISA resource name 2"=w211:refnum<visa-resource-name>)  [unwired: 3 in, 1 out]
        n96 = String To Byte Array(string="Laser Temperature ready\n\rCommand>\n\r") -> (unsigned byte array=w220:u8[])
        n97 = String To Byte Array(string=w212) -> (unsigned byte array=w219:u8[])
        n98 = Equal?(x=w220, y=w219) -> (x = y?=w218:bool[])
        n99 = Boolean To (0,1)(Boolean=w218) -> (0, 1=w217:i16[])
        n100 = Multiply Array Elements(1:w217) -> (0:w216:i16)
        n101 = Not Equal To 0?(x=w216) -> (x != 0?=w215:bool)
        "Laser ready" <- w215
        n102 = case shown="False" w215 {
          tunnel: w212 -> [w229 _]
          tunnel: [w227 0] -> w214
          frame False {
            n103 = Scan From String(format string="%d", input string=w229, initial scan location=46) -> (output 1=w227:i32)  [unwired: 2 in, 3 out]
          }
          frame True {
          }
        }
        "Time to go" <- w214
        n104 = Wait (ms)(milliseconds to wait=1000) -> ()  [unwired: 1 out]
      }
      n105 = call "Query_laser.vi"("error in (no error)"=w209, "String in"="M=1\n", "VISA resource name"=w189) -> ("error out"=w191:errorcluster, "VISA resource name 2"=w190:refnum<visa-resource-name>)  [unwired: 4 in, 2 out]
      n106 = Initialize Array(0, 200) -> (w192:i32[])
      n107 = Initialize Array(0.0, 200) -> (w195:dbl[])
      n108 = while {
        tunnel: w190 -> [w246]
        tunnel: w191 -> [w247]
        tunnel: [w244] -> w199
        tunnel: [w245] -> w198
        shift-right: [w240] -> _
        shift-left: w195 -> [w242]
        shift-right: [w239] -> _
        shift-left: w192 -> [w241]
        stop <- w238 stop-if-true
        # "Laser Running"
        n109 = stacked-sequence {
          seq-local: [w251 _ _ _ _ _] -> [_ w267 w283 w299 w309 w323]
          tunnel: w246 -> [w254 w271 w280 w298 w308 w320]
          tunnel: w247 -> [w255 _ _ _ _ _]
          tunnel: [_ _ _ _ _ w322] -> w245
          tunnel: [_ _ _ _ _ w321] -> w244
          tunnel: w242 -> [w253 _ _ _ _ _]
          tunnel: w241 -> [_ _ w282 _ _ _]
          tunnel: [w252 _ _ _ _ _] -> w240
          tunnel: [_ _ w281 _ _ _] -> w239
          frame #0 {
            n110 = call "Query_laser.vi"("error in (no error)"=w255, "String in"="T?\n", "VISA resource name"=w254) -> ("error out"=w251:errorcluster, "String out"=w249:string)  [unwired: 4 in, 2 out]
            n111 = String Length(string=w249) -> (length=w250:i32)
            n112 = Greater Than 0?(x=w250) -> (x > 0?=w248:bool)
            n113 = case shown="True" w248 {
              tunnel: w253 -> [w257 w263]
              tunnel: [w257 w259] -> w252
              tunnel: w249 -> [_ w258]
              frame False {
              }
              frame True {
                n114 = Scan From String(format string="%4.1f", input string=w258, initial scan location=15) -> (output 1=w264:dbl)  [unwired: 2 in, 3 out]
                n115 = Insert Into Array(array=w263, new element=w264) -> (w262:dbl[])  [unwired: 1 in]
                n116 = Delete From Array(array=w262, length=1, index=0) -> (array with subset deleted=w259:dbl[])  [unwired: 1 out]
                "Laser Temperature" <- w259
              }
            }
          }
          frame #1 {
            n117 = call "Query_laser.vi"("error in (no error)"=w267, "String in"="p?\n", "VISA resource name"=w271) -> ("String out"=w270:string)  [unwired: 4 in, 3 out]
            n118 = String Length(string=w270) -> (length=w269:i32)
            n119 = Greater Than 0?(x=w269) -> (x > 0?=w268:bool)
            n120 = case shown="True" w268 {
              tunnel: w270 -> [_ w273]
              frame False {
              }
              frame True {
                n121 = Scan From String(format string="%d", input string=w273, initial scan location=26) -> (output 1=→"Preamplifier":i32)  [unwired: 2 in, 3 out]
              }
            }
          }
          frame #2 {
            n122 = call "Query_laser.vi"("error in (no error)"=w283, "String in"="c?\n", "VISA resource name"=w280) -> ("String out"=w277:string)  [unwired: 4 in, 3 out]
            n123 = String Length(string=w277) -> (length=w279:i32)
            n124 = Greater Than 0?(x=w279) -> (x > 0?=w278:bool)
            n125 = case shown="True" w278 {
              tunnel: w282 -> [w285 w288]
              tunnel: [w285 w287] -> w281
              tunnel: w277 -> [_ w286]
              frame False {
              }
              frame True {
                n126 = Scan From String(format string="%d\n\rAmplifier photodiode =%d", input string=w286, initial scan location=38) -> (output 2=w289:i32)  [unwired: 4 in, 3 out]
                n127 = Insert Into Array(array=w288, new element=w289) -> (w292:i32[])  [unwired: 1 in]
                n128 = Delete From Array(array=w292, length=1, index=0) -> (array with subset deleted=w287:i32[])  [unwired: 1 out]
                "Amplifier" <- w287
              }
            }
          }
          frame #3 {
            n129 = call "Query_laser.vi"("error in (no error)"=w299, "String in"="b?\n", "VISA resource name"=w298) -> ("String out"=w296:string)  [unwired: 4 in, 3 out]
            n130 = String Length(string=w296) -> (length=w297:i32)
            n131 = Greater Than 0?(x=w297) -> (x > 0?=w295:bool)
            n132 = case shown="True" w295 {
              tunnel: w296 -> [_ w301]
              frame False {
              }
              frame True {
                n133 = Scan From String(format string="%d", input string=w301, initial scan location=28) -> (output 1=→"Backreflection":i32)  [unwired: 2 in, 3 out]
              }
            }
          }
          frame #4 {
            n134 = call "Query_laser.vi"("error in (no error)"=w309, "String in"="q?\n", "VISA resource name"=w308) -> ("String out"=w306:string)  [unwired: 4 in, 3 out]
            n135 = String Length(string=w306) -> (length=w307:i32)
            n136 = Greater Than 0?(x=w307) -> (x > 0?=w305:bool)
            n137 = case shown="True" w305 {
              tunnel: w306 -> [_ w311]
              frame False {
              }
              frame True {
                n138 = Scan From String(format string="%d,%d", input string=w311, initial scan location=1) -> (output 1=w312:i32)  [unwired: 4 in, 3 out]
                n139 = Divide(x=w312, y=15) -> (x/y=→"Power set":dbl)
              }
            }
          }
          frame #5 {
            n140 = call "Query_laser.vi"("error in (no error)"=w323, "String in"="g?\n", "VISA resource name"=w320) -> ("error out"=w321:errorcluster, "String out"=w318:string, "VISA resource name 2"=w322:refnum<visa-resource-name>)  [unwired: 4 in, 1 out]
            n141 = String Length(string=w318) -> (length=w319:i32)
            n142 = Greater Than 0?(x=w319) -> (x > 0?=w317:bool)
            n143 = case shown="True" w317 {
              tunnel: w318 -> [_ w325]
              frame False {
              }
              frame True {
                n144 = Scan From String(format string="%d", input string=w325, initial scan location=12) -> (output 1=→"Photodiode":i32)  [unwired: 2 in, 3 out]
              }
            }
          }
        }
        n145 = local read "Global Stop"() -> (w238:bool)
        n146 = Wait (ms)(milliseconds to wait=u32 200) -> ()  [unwired: 1 out]
      }
      n147 = call "Query_laser.vi"("error in (no error)"=w199, "String in"="M=0\n", "VISA resource name"=w198) -> ("error out"=w200:errorcluster, "VISA resource name 2"=w201:refnum<visa-resource-name>)  [unwired: 4 in, 2 out]
      n148 = call "Query_laser.vi"("error in (no error)"=w200, "String in"="X=1\n", "VISA resource name"=w201) -> ("error out"=w204:errorcluster, "VISA resource name 2"=w203:refnum<visa-resource-name>)  [unwired: 4 in, 2 out]
      n149 = VISA Close(VISA resource name=w203, error in (no error)=w204) -> (error out=w188:errorcluster)
    }
  }
  n150 = local read "PI SystemNumber"() -> (w37:i32)
  n151 = local read "PI SystemNumber"() -> (w38:i32)
  n152 = while {
    shift-right: [w360] -> w32
    shift-left: w2 -> [w363]
    tunnel: w34 -> [w348]
    stop <- w362 stop-if-true
    n153 = control-ref of="ShowTab"() -> (w361:refnum<vi>)
    n154 = control-ref of="WS File Tree"() -> (w330:refnum<vi>)
    n155 = event shown="[19] \"Power Button\": Value Change" {
      selector: _ -> [_ _ _ _ _ _ _ _ _ _ _ _ _ _ _ _ _ _ _ _ _]
      dyn-events: _ -> [_ _ _ _ _ _ _ _ _ _ _ _ _ _ _ _ _ _ _ _ _]
      timeout: 100 -> [_ _ _ _ _ _ _ _ _ _ _ _ _ _ _ _ _ _ _ _ _]
      tunnel: w363 -> [w365 w367 _ _ _ _ w517 w533 _ _ _ _ w607 w636 w639 w675 _ w729 _ w901 w952]
      tunnel: [w365 w367 _ _ _ _ w508 w533 _ _ _ _ w606 w635 w637 w672 _ w728 _ w892 w950] -> w360
      tunnel: w330 -> [_ _ _ _ _ _ _ _ _ _ _ _ _ _ w641 w676 _ _ _ _ _]
      tunnel: w361 -> [_ _ w369 w395 w427 _ _ _ w540 w558 w566 w574 _ _ _ _ _ _ _ _ _]
      tunnel: "Aquire Image" -> [_ _ _ _ _ _ _ _ _ _ _ _ _ _ _ _ _ _ _ _ _]
      tunnel: "Save Color Image" -> [_ _ _ _ _ _ _ _ _ _ _ _ _ _ _ _ _ _ _ _ _]
      tunnel: "Open MSW" -> [_ _ _ _ _ _ _ _ _ _ _ _ _ _ _ _ _ _ _ _ _]
      tunnel: "Find Mols" -> [_ _ _ _ _ _ _ _ _ _ _ _ _ _ _ _ _ _ _ _ _]
      tunnel: "Auto Meas" -> [_ _ _ _ _ _ _ _ _ _ _ _ _ _ _ _ _ _ _ _ _]
      tunnel: "Line Scan" -> [_ _ _ _ _ _ _ _ _ _ _ _ _ _ _ _ _ _ _ _ _]
      tunnel: "Grid Measurement" -> [_ _ _ _ _ _ _ _ _ _ _ _ _ _ _ _ _ _ _ _ _]
      tunnel: "New MSW" -> [_ _ _ _ _ _ _ _ _ _ _ _ _ _ _ _ _ _ _ _ _]
      tunnel: "Stop Program" -> [_ _ _ _ _ _ _ _ _ _ _ _ _ _ _ _ _ _ _ _ _]
      tunnel: "Point Measurement" -> [_ _ _ _ _ _ _ _ _ _ _ _ _ _ _ _ _ _ _ _ _]
      tunnel: "Move Stage" -> [_ _ _ _ _ _ _ _ _ _ _ _ _ _ _ _ _ _ _ _ _]
      tunnel: w348 -> [_ _ _ _ _ _ _ _ _ _ _ _ _ _ _ _ _ _ _ w893 w951]
      tunnel: "Get Position" -> [_ _ _ _ _ _ _ _ _ _ _ _ _ _ _ _ _ _ _ _ _]
      tunnel: [_ _ _ _ _ _ _ _ _ _ _ _ w602 w633 _ _ _ _ _ _ _] -> w346
      tunnel: [_ _ _ _ _ _ _ _ _ _ _ _ w603 w632 _ _ _ _ _ _ _] -> w329
      tunnel: [_ _ _ _ _ _ _ _ _ _ _ _ w604 w631 _ _ _ _ _ _ _] -> w345
      tunnel: "How long?" -> [_ _ _ _ _ _ _ _ _ _ _ _ _ _ _ _ _ _ _ _ _]
      tunnel: "Start 3D FCS Abel Scan" -> [_ _ _ _ _ _ _ _ _ _ _ _ _ _ _ _ _ _ _ _ _]
      tunnel: "Mesaurement Time (Sec) / Step" -> [_ _ _ _ _ w479 w516 _ _ _ _ _ _ _ _ _ _ _ _ _ _]
      tunnel: "Y Stepsize" -> [_ _ _ _ _ w478 w512 _ _ _ _ _ _ _ _ _ _ _ _ _ _]
      tunnel: "X Stepsize" -> [_ _ _ _ _ w477 w511 _ _ _ _ _ _ _ _ _ _ _ _ _ _]
      tunnel: "Z Stepsize" -> [_ _ _ _ _ w476 w510 _ _ _ _ _ _ _ _ _ _ _ _ _ _]
      tunnel: "FCS Point Measurement" -> [_ _ _ _ _ _ w529 _ _ _ _ _ _ _ _ _ _ _ _ _ _]
      tunnel: "Abeltrapping (EodScan)" -> [_ _ _ _ _ _ w528 _ _ _ _ _ _ _ _ _ _ _ _ _ _]
      tunnel: "Z End" -> [_ _ _ _ _ w475 w527 _ _ _ _ _ _ _ _ _ _ _ _ _ _]
      tunnel: "X End" -> [_ _ _ _ _ w474 w521 _ _ _ _ _ _ _ _ _ _ _ _ _ _]
      tunnel: "Y End" -> [_ _ _ _ _ w473 w524 _ _ _ _ _ _ _ _ _ _ _ _ _ _]
      tunnel: "Z Start" -> [_ _ _ _ _ w472 w513 _ _ _ _ _ _ _ _ _ _ _ _ _ _]
      tunnel: "X Start" -> [_ _ _ _ _ w471 w515 _ _ _ _ _ _ _ _ _ _ _ _ _ _]
      tunnel: "Y Start" -> [_ _ _ _ _ w470 w514 _ _ _ _ _ _ _ _ _ _ _ _ _ _]
      tunnel: w330 -> [_ _ _ _ _ _ _ _ _ _ _ _ _ _ _ _ _ _ _ _ _]
      event Timeout {
        n156 = event-data() -> ()  [unwired: 1 in, 2 out]
      }
      event "Stop Program": Mouse Up {
        n157 = event-data() -> ()  [unwired: 1 in, 7 out]
        n158 = local write "Global Stop"(TRUE ("Global Stop")) -> ()
      }
      event "Aquire Image": Mouse Up {
        n159 = event-data() -> ()  [unwired: 1 in, 7 out]
        n160 = local read "Workspace"() -> (w372:path)
        n161 = local read "Running"() -> (w375:bool)
        n162 = local read "Task"() -> (w368:T1)
        n163 = Not Equal?(x=w372, y=path "") -> (x != y?=w370:bool)
        n164 = Not(x=w375) -> (.not. x?=w374:bool)
        n165 = case shown="True" w370 {
          tunnel: w374 -> [_ w380]
          tunnel: T12."Aquire Image" ("Do Measurement") -> [_ w379]
          tunnel: w369 -> [_ w378]
          tunnel: w368 -> [_ w377]
          frame False {
            # "No Workspace Open"
            n166 = One Button Dialog(message="No Workspace Opened") -> ()  [unwired: 1 in, 1 out]
          }
          frame True {
            # "Aquire Image if not Running"
            n167 = case shown="True" w380 {
              tunnel: w379 -> [w383 w391]
              tunnel: w378 -> [_ w388]
              tunnel: w377 -> [w381 _]
              frame False {
                n168 = Equal?(x=w381, y=w383) -> (x = y?=w382:bool)
                n169 = case shown="False" w382 {
                  frame False {
                  }
                  frame True {
                    n170 = local write "Stop Measurement"(TRUE ("Stop Measurement")) -> ()
                  }
                }
              }
              frame True {
                w386 = enum16{"Show All", "Hide Tab", "Show Tab"}."Hide Tab" ("Action")
                n171 = local write "Task"(w391) -> ()
                n172 = property on="Aquire Image" class="Bool"("BoolText.Text"="Stop Aquire" ("Caption.Text"), "BoolText.TextColor"=u32 16711680 ("Boolean Text.Colors:FG Color")) -> ()  [unwired: 2 in, 2 out]
                n173 = local write "Running"(TRUE ("Measurement Running")) -> ()
                n174 = call "MTS_ShowHideTabs.vi"("Action"=w386, "Tab Caption"="Video", "ShowTab"=w388) -> ("ShowTab out"=w387:refnum<vi>)  [unwired: 7 in, 1 out]
                n175 = call "MTS_ShowHideTabs.vi"("Action"=w386, "Tab Caption"="Auto Measurement", "ShowTab"=w387) -> ()  [unwired: 7 in, 2 out]
              }
            }
          }
        }
      }
      event "Line Scan": Mouse Up {
        n176 = event-data() -> ()  [unwired: 1 in, 7 out]
        n177 = local read "Workspace"() -> (w398:path)
        n178 = local read "Task"() -> (w399:T1)
        n179 = local read "Running"() -> (w401:bool)
        n180 = Not Equal?(x=w398, y=path "") -> (x != y?=w396:bool)
        n181 = Not(x=w401) -> (.not. x?=w400:bool)
        n182 = case shown="True" w396 {
          tunnel: w400 -> [_ w406]
          tunnel: T13."Aquire Line Scan" ("Do Measurement") -> [_ w405]
          tunnel: w399 -> [_ w404]
          tunnel: w395 -> [_ w403]
          frame False {
            # "No Workspace Open"
            n183 = One Button Dialog(message="No Workspace Opened") -> ()  [unwired: 1 in, 1 out]
          }
          frame True {
            # "Aquire Image if not Running"
            n184 = case shown="False" w406 {
              tunnel: w405 -> [w408 w419]
              tunnel: w404 -> [w409 _]
              tunnel: w403 -> [_ w416]
              frame False {
                n185 = Equal?(x=w409, y=w408) -> (x = y?=w407:bool)
                n186 = case shown="True" w407 {
                  frame False {
                  }
                  frame True {
                    n187 = local write "Stop Measurement"(TRUE ("Stop Measurement")) -> ()
                  }
                }
              }
              frame True {
                w411 = enum16{"Show All", "Hide Tab", "Show Tab"}."Hide Tab" ("Action")
                n188 = local write "Running"(TRUE ("Measurement Running")) -> ()
                n189 = call "MTS_ShowHideTabs.vi"("Action"=w411, "Tab Caption"="Video", "ShowTab"=w416) -> ("ShowTab out"=w414:refnum<vi>)  [unwired: 7 in, 1 out]
                n190 = property on="Line Scan" class="Bool"("BoolText.Text"="Stop Scan" ("Caption.Text"), "BoolText.TextColor"=u32 16711680 ("Boolean Text.Colors:FG Color")) -> ()  [unwired: 2 in, 2 out]
                n191 = local write "Task"(w419) -> ()
                n192 = call "MTS_ShowHideTabs.vi"("Action"=w411, "Tab Caption"="Image", "ShowTab"=w414) -> ("ShowTab out"=w412:refnum<vi>)  [unwired: 7 in, 1 out]
                n193 = call "MTS_ShowHideTabs.vi"("Action"=w411, "Tab Caption"="Auto Measurement", "ShowTab"=w412) -> ()  [unwired: 7 in, 2 out]
              }
            }
          }
        }
      }
      event "Grid Measurement": Mouse Up {
        n194 = event-data() -> ()  [unwired: 1 in, 7 out]
        n195 = local read "Workspace"() -> (w430:path)
        n196 = local read "Task"() -> (w431:T1)
        n197 = local read "Running"() -> (w433:bool)
        n198 = local read "X-Position"() -> (w423:dbl)
        n199 = local read "Y-Position"() -> (w424:dbl)
        n200 = local read "Z-Position"() -> (w425:dbl)
        n201 = Not Equal?(x=w430, y=path "") -> (x != y?=w428:bool)
        n202 = Not(x=w433) -> (.not. x?=w432:bool)
        n203 = Build Array(w423, w424, w425) -> (w422:dbl[])
        n204 = case shown="True" w428 {
          tunnel: w432 -> [_ w439]
          tunnel: T14."Grid Measurement" ("Do Measurement") -> [_ w438]
          tunnel: w431 -> [_ w437]
          tunnel: w427 -> [_ w436]
          tunnel: w422 -> [_ w435]
          frame False {
            # "No Workspace Open"
            n205 = One Button Dialog(message="No Workspace Opened") -> ()  [unwired: 1 in, 1 out]
          }
          frame True {
            # "Aquire Grid if not Running"
            n206 = case shown="True" w439 {
              tunnel: w438 -> [w441 w462]
              tunnel: w437 -> [w442 _]
              tunnel: w436 -> [_ w459]
              tunnel: w435 -> [_ w445]
              frame False {
                n207 = Equal?(x=w442, y=w441) -> (x = y?=w440:bool)
                n208 = case shown="True" w440 {
                  frame False {
                  }
                  frame True {
                    n209 = local write "Stop Measurement"(TRUE ("Stop Measurement")) -> ()
                  }
                }
              }
              frame True {
                w454 = enum16{"Show All", "Hide Tab", "Show Tab"}."Hide Tab" ("Action")
                n210 = local write "Running"(TRUE ("Measurement Running")) -> ()
                n211 = call "MTS_ShowHideTabs.vi"("Action"=w454, "Tab Caption"="Video", "ShowTab"=w459) -> ("ShowTab out"=w457:refnum<vi>)  [unwired: 7 in, 1 out]
                n212 = property on="Grid Measurement" class="Bool"("BoolText.Text"="Stop Scan" ("Caption.Text"), "BoolText.TextColor"=u32 16711680 ("Boolean Text.Colors:FG Color")) -> ()  [unwired: 2 in, 2 out]
                n213 = local read "X-Axis Offset"() -> (w453:dbl)
                n214 = local read "Y-Axis Offset"() -> (w452:dbl)
                n215 = local read "Z-Axis Offset"() -> (w451:dbl)
                n216 = local write "Task"(w462) -> ()
                n217 = call "MTS_ShowHideTabs.vi"("Action"=w454, "Tab Caption"="Image", "ShowTab"=w457) -> ("ShowTab out"=w455:refnum<vi>)  [unwired: 7 in, 1 out]
                n218 = Build Array(w453, w452, w451) -> (w444:dbl[])
                n219 = call "MTS_ShowHideTabs.vi"("Action"=w454, "Tab Caption"="Auto Measurement", "ShowTab"=w455) -> ()  [unwired: 7 in, 2 out]
                n220 = local read "X-Axis Points"() -> (w450:u16)
                n221 = local read "Y-Axis Points"() -> (w449:u16)
                n222 = local read "Z-Axis Points"() -> (w448:u16)
                n223 = Build Array(w450, w449, w448) -> (w446:u16[])
                n224 = call "MTS_GenGridScanList.vi"("Offsets"=w444, "Points"=w446, "Starting"=w445) -> ("Grid Points"=→"Grid Points":dbl[][])  [unwired: 8 in]
              }
            }
          }
        }
      }
      event "How long?": Value Change {
        n225 = event-data() -> ()  [unwired: 1 in, 5 out]
        n226 = Build Array(w479, w478, w477, w476, w475, w474, w473, w472, w471, w470) -> (w469:dbl[])
        n227 = for {
          tunnel: w469 -> [w507] mode=indexing
          tunnel: [w506] -> w468 mode=indexing
          n228 = Not Equal To 0?(x=w507) -> (x != 0?=w506:bool)
        }
        n229 = Boolean Array To Number(Boolean array=w468) -> (number=w467:u32)
        n230 = Not Equal To 0?(x=w467) -> (x != 0?=w466:bool)
        n231 = case shown="True" w466 {
          tunnel: [0.0 w492] -> w465
          tunnel: w479 -> [_ w491]
          tunnel: w478 -> [_ w490]
          tunnel: w477 -> [_ w489]
          tunnel: w476 -> [_ w488]
          tunnel: w475 -> [_ w487]
          tunnel: w474 -> [_ w486]
          tunnel: w473 -> [_ w485]
          tunnel: w472 -> [_ w484]
          tunnel: w471 -> [_ w483]
          tunnel: w470 -> [_ w482]
          frame False {
            n232 = One Button Dialog(message="Supply valid information for the scanner x-z and stepsize and apply a measurement time ") -> ()  [unwired: 1 in, 1 out]
          }
          frame True {
            w493 = 60.0 ("y")
            # "to hours"
            # "to minutes"
            n233 = Subtract(x=w486, y=w483) -> (x-y=w505:dbl)
            n234 = Subtract(x=w485, y=w482) -> (x-y=w502:dbl)
            n235 = Subtract(x=w487, y=w484) -> (x-y=w500:dbl)
            n236 = Divide(x=w505, y=w489) -> (x/y=w504:dbl)
            n237 = Divide(x=w502, y=w490) -> (x/y=w503:dbl)
            n238 = Divide(x=w500, y=w488) -> (x/y=w501:dbl)
            n239 = Multiply(x=w491, y=w504) -> (x*y=w499:dbl)
            n240 = Multiply(x=w491, y=w503) -> (x*y=w498:dbl)
            n241 = Multiply(x=w491, y=w501) -> (x*y=w497:dbl)
            n242 = Add(x=w499, y=w498) -> (x+y=w496:dbl)
            n243 = Add(x=w497, y=w496) -> (x+y=w495:dbl)
            n244 = Divide(x=w495, y=w493) -> (x/y=w494:dbl)
            n245 = Divide(x=w494, y=w493) -> (x/y=w492:dbl)
          }
        }
        "Estimated Time (h)" <- w465
      }
      event "Start 3D FCS Abel Scan": Value Change {
        n246 = event-data() -> ()  [unwired: 1 in, 5 out]
        n247 = local write "X-Position"(w515) -> ()
        n248 = local write "Z-Position"(w513) -> ()
        n249 = local write "Y-Position"(w514) -> ()
        n250 = local read "PI SystemNumber"() -> (w518:i32)
        n251 = Subtract(x=w527, y=w513) -> (x-y=w525:dbl)
        n252 = Subtract(x=w524, y=w514) -> (x-y=w523:dbl)
        n253 = Subtract(x=w521, y=w515) -> (x-y=w520:dbl)
        n254 = Divide(x=w525, y=w510) -> (x/y=→"Z Steps":dbl)
        n255 = Divide(x=w523, y=w512) -> (x/y=→"Y Steps":dbl)
        n256 = Divide(x=w520, y=w511) -> (x/y=→"X Steps":dbl)
        n257 = call "PI Goto GPIB.vi"("System no."=w518, "x-position"=w515, "y-position"=w514, "z-position"=w513, "error in"=w517) -> ("error out"=w509:errorcluster)  [unwired: 14 in]
        n258 = property on="Measurement Time" class="DigNum (strict)"("Value"=w516) -> ()  [unwired: 2 in, 2 out]
        n259 = local write "Y Stepsize"(w512) -> ()
        n260 = local write "X Stepsize"(w511) -> ()
        n261 = local write "Z Stepsize"(w510) -> ()
        n262 = case shown="No Error" w509 {
          selector: w509 -> [w530 w532]
          tunnel: [w530 w532] -> w508
          frame No Error {
            "3dAbelFcs" <- TRUE
          }
          frame Error {
          }
        }
        "Abeltrapping (EodScan) 2" <- w528
        "FCS Point Measurement 2" <- w529
      }
      event "X-Axis Points", "Z-Axis Points", "Y-Axis Points": Value Change {
        n263 = event-data() -> ()  [unwired: 1 in, 5 out]
      }
      event "Auto Meas": Mouse Up {
        n264 = event-data() -> ()  [unwired: 1 in, 7 out]
        n265 = local read "Workspace"() -> (w542:path)
        n266 = local read "Task"() -> (w543:T1)
        n267 = local read "Last Image File No"() -> (w538:i32)
        n268 = local read "Running"() -> (w545:bool)
        n269 = Not Equal?(x=w542, y=path "") -> (x != y?=w536:bool)
        n270 = Not(x=w545) -> (.not. x?=w544:bool)
        n271 = Not Equal?(x=w538, y=-1) -> (x != y?=w535:bool)
        n272 = And(x=w536, y=w535) -> (x .and. y?=w534:bool)
        n273 = case shown="True" w534 {
          tunnel: w544 -> [_ w550]
          tunnel: T15."Auto Measurement Control" ("Do Measurement") -> [_ w549]
          tunnel: w543 -> [_ w548]
          tunnel: w540 -> [_ w547]
          frame False {
            # "No Workspace Open"
            n274 = One Button Dialog(message="No Workspace Opened or No Image Acquired") -> ()  [unwired: 1 in, 1 out]
          }
          frame True {
            # "Start Auto Measurement"
            n275 = case shown="True" w550 {
              tunnel: w549 -> [_ w556]
              tunnel: w548 -> [_ _]
              tunnel: w547 -> [_ w553]
              frame False {
                n276 = case shown="True" FALSE {
                  frame False {
                  }
                  frame True {
                    n277 = local write "Stop Measurement"(TRUE ("Stop Measurement")) -> ()
                  }
                }
              }
              frame True {
                n278 = local write "Running"(TRUE ("Measurement Running")) -> ()
                n279 = local write "Task"(w556) -> ()
                n280 = call "MTS_ShowHideTabs.vi"("Action"=enum16{"Show All", "Hide Tab", "Show Tab"}."Hide Tab", "Tab Caption"="Video", "ShowTab"=w553) -> ()  [unwired: 7 in, 2 out]
              }
            }
          }
        }
      }
      event "Save Color Image": Mouse Up {
        n281 = event-data() -> ()  [unwired: 1 in, 7 out]
        n282 = local read "Active pt3"() -> (w561:path)
        n283 = Not Equal?(x=w561, y=path "") -> (x != y?=w559:bool)
        n284 = case shown="True" w559 {
          tunnel: T16."Save Color Image" ("Do Measurement") -> [_ w565]
          tunnel: w558 -> [_ _]
          frame False {
            # "No Workspace Open"
            n285 = One Button Dialog(message="No pt3 File opened") -> ()  [unwired: 1 in, 1 out]
          }
          frame True {
            # "Aquire Image if not Running"
            n286 = local write "Running"(TRUE ("Measurement Running")) -> ()
            n287 = local write "Task"(w565) -> ()
          }
        }
      }
      event "Find Mols": Mouse Up {
        n288 = event-data() -> ()  [unwired: 1 in, 7 out]
        n289 = local read "Active pt3"() -> (w569:path)
        n290 = Not Equal?(x=w569, y=path "") -> (x != y?=w567:bool)
        n291 = case shown="True" w567 {
          tunnel: T16."Find Single Mol." ("Do Measurement") -> [_ w573]
          tunnel: w566 -> [_ _]
          frame False {
            # "No Workspace Open"
            n292 = One Button Dialog(message="No pt3 File opened") -> ()  [unwired: 1 in, 1 out]
          }
          frame True {
            # "Aquire Image if not Running"
            n293 = local write "Running"(TRUE ("Measurement Running")) -> ()
            n294 = local write "Task"(w573) -> ()
          }
        }
      }
      event "Point Measurement": Mouse Up {
        n295 = event-data() -> ()  [unwired: 1 in, 7 out]
        n296 = local read "Workspace"() -> (w577:path)
        n297 = local read "Running"() -> (w581:bool)
        n298 = local read "Task"() -> (w578:T1)
        n299 = Not Equal?(x=w577, y=path "") -> (x != y?=w575:bool)
        n300 = Not(x=w581) -> (.not. x?=w580:bool)
        n301 = case shown="True" w575 {
          tunnel: w580 -> [_ w586]
          tunnel: T12."Point Measurement" ("Do Measurement") -> [_ w585]
          tunnel: w578 -> [_ w584]
          tunnel: w574 -> [_ w583]
          frame False {
            # "No Workspace Open"
            n302 = One Button Dialog(message="No Workspace Opened") -> ()  [unwired: 1 in, 1 out]
          }
          frame True {
            # "Aquire Image if not Running"
            n303 = case shown="True" w586 {
              tunnel: w585 -> [w588 w599]
              tunnel: w584 -> [w589 _]
              tunnel: w583 -> [_ w591]
              frame False {
                n304 = Equal?(x=w589, y=w588) -> (x = y?=w587:bool)
                n305 = case shown="False" w587 {
                  frame False {
                  }
                  frame True {
                    n306 = local write "Stop Measurement"(TRUE ("Stop Measurement")) -> ()
                  }
                }
              }
              frame True {
                w592 = enum16{"Show All", "Hide Tab", "Show Tab"}."Hide Tab" ("Action")
                n307 = local write "Running"(TRUE ("Measurement Running")) -> ()
                n308 = call "MTS_ShowHideTabs.vi"("Action"=w592, "Tab Caption"="Video", "ShowTab"=w591) -> ("ShowTab out"=w595:refnum<vi>)  [unwired: 7 in, 1 out]
                n309 = property on="Point Measurement" class="Bool"("BoolText.Text"="Stop Aquire" ("Caption.Text"), "BoolText.TextColor"=u32 16711680 ("Boolean Text.Colors:FG Color")) -> ()  [unwired: 2 in, 2 out]
                n310 = local write "Task"(w599) -> ()
                n311 = call "MTS_ShowHideTabs.vi"("Action"=w592, "Tab Caption"="Image", "ShowTab"=w595) -> ("ShowTab out"=w593:refnum<vi>)  [unwired: 7 in, 1 out]
                n312 = call "MTS_ShowHideTabs.vi"("Action"=w592, "Tab Caption"="Auto Measurement", "ShowTab"=w593) -> ()  [unwired: 7 in, 2 out]
              }
            }
          }
        }
      }
      event "X-Position", "Y-Position", "Z-Position": Value Change; "Move Stage": Mouse Up {
        n313 = event-data() -> ()  [unwired: 1 in, 3 out]
        n314 = local read "PI SystemNumber"() -> (w605:i32)
        n315 = local read "Workspace"() -> (w610:path)
        n316 = local read "Running"() -> (w612:bool)
        n317 = Not Equal?(x=w610, y=path "") -> (x != y?=w608:bool)
        n318 = Not(x=w612) -> (.not. x?=w611:bool)
        n319 = case shown="True" w608 {
          tunnel: w611 -> [_ w620]
          tunnel: w607 -> [_ w619]
          tunnel: [_ w618] -> w606
          tunnel: w605 -> [_ w617]
          tunnel: [_ w616] -> w602
          tunnel: [_ w615] -> w603
          tunnel: [_ w614] -> w604
          frame False {
            # "No Workspace Open"
            n320 = One Button Dialog(message="No Workspace Opened") -> ()  [unwired: 1 in, 1 out]
          }
          frame True {
            # "Move Stage if not Running"
            n321 = case shown="True" w620 {
              tunnel: w619 -> [_ w627]
              tunnel: [_ w625] -> w618
              tunnel: w617 -> [_ w624]
              tunnel: [_ w623] -> w616
              tunnel: [_ w622] -> w615
              tunnel: [_ w621] -> w614
              frame False {
              }
              frame True {
                n322 = local read "X-Position"() -> (w630:dbl)
                n323 = local read "Y-Position"() -> (w629:dbl)
                n324 = local read "Z-Position"() -> (w628:dbl)
                n325 = call "PI Goto GPIB.vi"("System no."=w624, "x-position"=w630, "y-position"=w629, "z-position"=w628, "error in"=w627) -> ("error out"=w626:errorcluster)  [unwired: 14 in]
                n326 = call "PI Pos GPIB.vi"("System no."=w624, "error in"=w626) -> ("x-position"=w621:dbl, "y-position"=w622:dbl, "z-position"=w623:dbl, "error out"=w625:errorcluster)  [unwired: 14 in]
              }
            }
          }
        }
        n327 = property on="x-position" class="DigNum (strict)"("Value"=w604) -> ()  [unwired: 2 in, 2 out]
        n328 = property on="y-position" class="DigNum (strict)"("Value"=w603) -> ()  [unwired: 2 in, 2 out]
        n329 = property on="z-position" class="DigNum (strict)"("Value"=w602) -> ()  [unwired: 2 in, 2 out]
      }
      event "Get Position": Value Change {
        n330 = event-data() -> ()  [unwired: 1 in, 5 out]
        n331 = local read "PI SystemNumber"() -> (w634:i32)
        n332 = call "PI Pos GPIB.vi"("System no."=w634, "error in"=w636) -> ("x-position"=w631:dbl, "y-position"=w632:dbl, "z-position"=w633:dbl, "error out"=w635:errorcluster)  [unwired: 14 in]
        n333 = property on="z-position" class="DigNum (strict)"("Value"=w633) -> ()  [unwired: 2 in, 2 out]
        n334 = property on="x-position" class="DigNum (strict)"("Value"=w631) -> ()  [unwired: 2 in, 2 out]
        n335 = property on="y-position" class="DigNum (strict)"("Value"=w632) -> ()  [unwired: 2 in, 2 out]
      }
      event "New MSW": Mouse Up {
        # "Default Name"
        n336 = event-data() -> ()  [unwired: 1 in, 7 out]
        n337 = flat-sequence {
          tunnel: [w657] -> w640
          tunnel: w639 -> [w657]
          frame #0 {
            n338 = local write "Running"(TRUE ("MeasRunig")) -> ()
          }
        }
        n339 = Get Date/Time In Seconds() -> (seconds since 1Jan1904=w654:timestamp)
        n340 = Format Date/Time String(time format string (%c)="%Y-%m-%d", seconds (now)=w654) -> (date/time string=w652:string)  [unwired: 1 out]
        n341 = Concatenate Strings(w652, ".msw" ("string")) -> (w650:string)
        n342 = call "File Dialog"("start path"=path "D:/", "prompt"="Create New Workspace", "button label"="Create", "default name"=w650, "error in"=w640, "pattern (all files)"="*.msw", "pattern label"="MT Scan Workspace") -> ("selected path"=w644:path, "cancelled"=w645:bool, "error out"=w643:errorcluster)  [unwired: 5 in, 1 out]
        n343 = case shown="False" w645 {
          tunnel: w644 -> [w663 _]
          tunnel: w643 -> [w669 w671]
          tunnel: [w661 w670] -> w638
          tunnel: w641 -> [w659 _]
          frame False {
            # "Create Empty Workspace"
            n344 = local write "Workspace"(w663) -> ()
            n345 = call "MTS_CreateWriteMSW.vi"("Rewrite"=TRUE, "error in (no error)"=w669, "Workspace Path"=w663) -> ("error out"=w662:errorcluster, "Created"=w666:string, "Comment (dup)"=w665:string, "Files in Workspace (dup)"=w664:T19)  [unwired: 5 in]
            n346 = call "MTS_Workspace.vi"("Workspace"=w663, "Operation"=T17."Set Workspace", "Created in"=w666, "New Comment"=w665, "Files in Workspace in"=w664) -> ("Files in Workspace"=w660:T20)  [unwired: 3 in, 3 out]
            n347 = call "MTS_BuildWSTree.vi"("error in"=w662, "Files in Workspace"=w660, "Tree Refnum"=w659) -> ("error out"=w661:errorcluster)  [unwired: 7 in, 1 out]
          }
          frame True {
            n348 = call <vilib>:"Clear Errors.vi"("error in (no error)"=w671) -> ("error out"=w670:errorcluster)  [unwired: 6 in]
          }
        }
        n349 = flat-sequence {
          tunnel: w638 -> [w655]
          tunnel: [w655] -> w637
          frame #0 {
            n350 = local write "Running"(FALSE ("MeasRunig")) -> ()
          }
        }
      }
      event "Open MSW": Mouse Up {
        n351 = event-data() -> ()  [unwired: 1 in, 7 out]
        n352 = flat-sequence {
          tunnel: w675 -> [w687]
          tunnel: [w687] -> w674
          frame #0 {
            n353 = local write "Running"(TRUE ("MeasRunig")) -> ()
          }
        }
        n354 = call "File Dialog2"("start path"=path "D:/", "prompt"="Create New Workspace", "button label"="Open", "error in"=w674, "pattern (all files)"="*.msw", "pattern label"="MT Scan Workspace") -> ("selected path"=w679:path, "cancelled"=w680:bool, "error out"=w678:errorcluster)  [unwired: 6 in, 1 out]
        n355 = case shown="False" w680 {
          tunnel: w679 -> [w693 _]
          tunnel: w678 -> [w698 w700]
          tunnel: [w691 w699] -> w673
          tunnel: w676 -> [w689 _]
          frame False {
            # "Open Workspace"
            n356 = local write "Workspace"(w693) -> ()
            n357 = call "MTS_ReadMSW.vi"("error in (no error)"=w698, "Workspace Path"=w693) -> ("error out"=w692:errorcluster, "Created"=w696:string, "Comment"=w695:string, "Files in Workspace"=w694:T21)  [unwired: 6 in]
            n358 = call "MTS_Workspace.vi"("Workspace"=w693, "Operation"=T17."Set Workspace", "Created in"=w696, "New Comment"=w695, "Files in Workspace in"=w694) -> ("Files in Workspace"=w690:T20)  [unwired: 3 in, 3 out]
            n359 = call "MTS_BuildWSTree.vi"("error in"=w692, "Files in Workspace"=w690, "Tree Refnum"=w689) -> ("error out"=w691:errorcluster)  [unwired: 7 in, 1 out]
          }
          frame True {
            n360 = call <vilib>:"Clear Errors.vi"("error in (no error)"=w700) -> ("error out"=w699:errorcluster)  [unwired: 6 in]
          }
        }
        n361 = flat-sequence {
          tunnel: w673 -> [w685]
          tunnel: [w685] -> w672
          frame #0 {
            n362 = local write "Running"(FALSE ("MeasRunig")) -> ()
          }
        }
      }
      event "Image": Mouse Up {
        w703 = 100.0 ("y")
        n363 = event-data() -> ("Coords"=w715:T22, "PlatMods"=w716:T23)  [unwired: 1 in, 5 out]
        n364 = local read "Axis"() -> (w711:enum32{"x-y", "x-z", "y-x", "y-z", "z-x", "z-y"})
        n365 = invoke on="Image" class="IntGraph (strict)" method="Map Coords To XY"("Coords"=w715) -> ("Map Coords To XY"=w712:bool, "XY"=w710:cluster{"X":dbl, "Y":dbl})  [unwired: 6 in, 5 out]
        n366 = Unbundle By Name(w716) -> ("Ctrl"=w713:bool)
        n367 = And(x=w712, y=w713) -> (x .and. y?=w714:bool)
        n368 = Unbundle(w710) -> ("X"=w709:dbl, "Y"=w706:dbl)
        n369 = Multiply(x=w709, y=w703) -> (x*y=w708:dbl)
        n370 = Multiply(x=w706, y=w703) -> (x*y=w705:dbl)
        n371 = Round To Nearest(number=w708) -> (nearest integer value=w707:dbl)
        n372 = Round To Nearest(number=w705) -> (nearest integer value=w704:dbl)
        n373 = Divide(x=w707, y=w703) -> (x/y=w702:dbl)
        n374 = Divide(x=w704, y=w703) -> (x/y=w701:dbl)
        n375 = case shown="True" w714 {
          tunnel: w711 -> [_ w719]
          tunnel: w702 -> [_ w718]
          tunnel: w701 -> [_ w717]
          frame False {
          }
          frame True {
            n376 = case shown="\"x-y\", Default" w719 {
              tunnel: w718 -> [w721 w723 w725]
              tunnel: w717 -> [w720 w722 w724]
              frame "x-y", Default {
                n377 = local write "X-Position"(w721) -> ()
                n378 = local write "Y-Position"(w720) -> ()
              }
              frame "x-z" {
                n379 = local write "X-Position"(w723) -> ()
                n380 = local write "Z-Position"(w722) -> ()
              }
              frame "y-z" {
                n381 = local write "Y-Position"(w725) -> ()
                n382 = local write "Z-Position"(w724) -> ()
              }
            }
          }
        }
      }
      event "WS File Tree": Value Change {
        n383 = event-data() -> ("NewVal"=w731:string)  [unwired: 1 in, 4 out]
        n384 = local read "Workspace"() -> (w727:path)
        n385 = Not Equal?(x=path "", y=w727) -> (x != y?=w730:bool)
        n386 = case shown="True" w730 {
          tunnel: w731 -> [_ w742]
          tunnel: w727 -> [_ w741]
          tunnel: w729 -> [w732 w740]
          tunnel: [w732 w739] -> w728
          frame False {
          }
          frame True {
            n387 = call "MTS_GetFileFromWS.vi"("Tree Label"=w742) -> ("File Header"=w738:T24, "File Found"=w737:bool)  [unwired: 9 in]
            n388 = Unbundle By Name(w738) -> ("File Type"=w736:T18)
            n389 = Equal?(x=w736, y=T18."pt3 File" ("File Type")) -> (x = y?=w734:bool)
            n390 = And(x=w737, y=w734) -> (x .and. y?=w733:bool)
            n391 = case shown="True" w733 {
              tunnel: w738 -> [_ w772]
              tunnel: w741 -> [_ w786]
              tunnel: w740 -> [w743 w783]
              tunnel: [w743 w776] -> w739
              frame False {
              }
              frame True {
                # "Image Intensity Array"
                n392 = control-ref of="Image"() -> (w754:refnum<vi>)
                n393 = Unbundle By Name(w772) -> ("File Path"=w785:path)
                n394 = Unbundle By Name(w772) -> ("Measurement Type"=w771:T25)
                n395 = Strip Path(path=w786) -> (stripped path=w784:path)  [unwired: 1 out]
                n396 = Strip Path(path=w785) -> (name=w773:string)  [unwired: 1 out]
                n397 = Build Path(base path=w784, name or relative path=w773) -> (appended path=w766:path)
                n398 = local write "Active pt3"(w766) -> ()
                n399 = call "HT3_Open.vi"("error in"=w783, "File Path"=w766) -> ("error out"=w782:errorcluster, "Header"=w751:T26, "refnum out"=w781:refnum<file>, "Image Header"=w774:T27)  [unwired: 3 in, 3 out]
                n400 = Unbundle By Name(w751) -> ("SyncRate"=w764:dbl)
                n401 = Divide(x=w764, y=10) -> (x/y=w757:dbl)
                n402 = Unbundle By Name(w774) -> ("PixX"=w749:i32, "PixY"=w748:i32, "PixResol"=w755:sgl, "X0"=w768:sgl, "Y0"=w756:sgl, "Z0"=w753:dbl, "Time Per Pixel [ms]"=w765:dbl, "TStartTo"=w762:sgl, "TStoptTo"=w761:sgl, "TStartFro"=w760:sgl, "TStopFro"=w759:sgl, "Pattern"=w752:i32)
                n403 = Unbundle By Name(w751) -> ("Laser"=w744:i32)
                n404 = Build Array(w762, w761, w760, w759) -> (w758:sgl[])
                n405 = Bundle("X0"=w768, "Y0"=w756, "Z0"=w753) -> (w767:cluster{"X0":sgl, "Y0":sgl, "Z0":dbl})  [unwired: 1 in]
                n406 = Bundle(w767, "PixX"=w749, "PixY"=w748, "Pattern"=w752, "PixResol"=w755, "Time Per Pixel [ms]"=w765, "Laser"=w744) -> (w775:T28)  [unwired: 1 in]
                n407 = Initialize Array(u16 0 ("element"), w748, w749, w744) -> (w769:u16[][][])
                n408 = case shown="\"Image File\"" w771 {
                  tunnel: w782 -> [w800 w840]
                  tunnel: w781 -> [w803 w839]
                  tunnel: [w802 w835] -> w780
                  tunnel: [w801 w836] -> w779
                  tunnel: [w792 w838] -> w778
                  tunnel: [w794 w837] -> w777
                  tunnel: w754 -> [w799 _]
                  tunnel: w775 -> [w798 _]
                  tunnel: w769 -> [w788 w834]
                  tunnel: w757 -> [w791 w833]
                  tunnel: w758 -> [w790 _]
                  tunnel: [w787 w834] -> w750
                  frame "Image File" {
                    n409 = call "Scan_SetGraphScales.vi"("error in (no error)"=w800, "Image Measurent Parameters"=w798, "Image"=w799) -> ("error out"=w797:errorcluster)  [unwired: 8 in]
                    n410 = while {
                      tunnel: w803 -> [w832]
                      shift-right: [FALSE ("Start From Top")] -> _
                      shift-left: TRUE ("Start From Top") -> [w827]
                      shift-right: [w826] -> w795
                      shift-left: w797 -> [w823]
                      tunnel: [w825] -> w793
                      tunnel: [w824] -> w802
                      tunnel: [w822] -> w801
                      tunnel: w791 -> [w821]
                      tunnel: [w819] -> w789
                      stop <- w829 stop-if-true
                      n411 = call "HT3_Read.vi"("Start From Top"=w827, "error in"=w823, "Data count"=1000000000, "refnum in"=w832) -> ("error out"=w826:errorcluster, "Data out"=w828:u32[], "refnum out"=w825:refnum<file>, "EOF?"=w829:bool)  [unwired: 4 in]
                      n412 = Array Size(array=w828) -> (size(s)=w820:i32)
                      n413 = call "HH_FileToImage_1.vi"("Data In"=w828, "Reset"=w827, "Data Count"=w820, "Trace Bins"=w821) -> ("Histograms"=w824:i32[][], "Trigger Times"=w819:u64[], "Traces"=w822:i32[][])  [unwired: 6 in, 3 out]
                    }
                    n414 = while {
                      tunnel: w793 -> [w818]
                      shift-right: [FALSE ("Start From Top")] -> _
                      shift-left: TRUE ("Start From Top") -> [w813]
                      shift-right: [w812] -> w794
                      shift-left: w795 -> [w810]
                      tunnel: [w811] -> w792
                      tunnel: w790 -> [w808]
                      tunnel: w789 -> [w807]
                      shift-right: [w805] -> w787
                      shift-left: w788 -> [w806]
                      stop <- w815 stop-if-true
                      n415 = call "HT3_Read.vi"("Start From Top"=w813, "error in"=w810, "Data count"=1000000000, "refnum in"=w818) -> ("error out"=w812:errorcluster, "Data out"=w814:u32[], "refnum out"=w811:refnum<file>, "EOF?"=w815:bool)  [unwired: 4 in]
                      n416 = Array Size(array=w814) -> (size(s)=w809:i32)
                      n417 = call "HH_FileToImage_2.vi"("Data In"=w814, "Reset"=w813, "Image Data In"=w806, "Data Count"=w809, "Trigger Times"=w807, "Trigger"=w808) -> ("Image Data Out"=w805:u16[][][])  [unwired: 6 in, 3 out]
                    }
                  }
                  frame "Point Measurement", Default {
                    n418 = while {
                      tunnel: w839 -> [w852]
                      tunnel: [w851] -> w838
                      tunnel: [w847] -> w836
                      tunnel: [w846] -> w835
                      shift-right: [FALSE] -> _
                      shift-left: TRUE ("Start From Top") -> [w854]
                      tunnel: w833 -> [w843]
                      shift-right: [w850] -> w837
                      shift-left: w840 -> [w853]
                      stop <- w844 stop-if-true
                      n419 = call "HT3_Read.vi"("Start From Top"=w854, "error in"=w853, "Data count"=1000000, "refnum in"=w852) -> ("error out"=w850:errorcluster, "Data out"=w848:u32[], "refnum out"=w851:refnum<file>, "EOF?"=w844:bool)  [unwired: 4 in]
                      n420 = Array Size(array=w848) -> (size(s)=w842:i32)
                      n421 = call "HH_FileToImage_1.vi"("Data In"=w848, "Reset"=w854, "Data Count"=w842, "Trace Bins"=w843) -> ("Histograms"=w846:i32[][], "Traces"=w847:i32[][])  [unwired: 6 in, 4 out]
                    }
                  }
                }
                n422 = local write "Histogram"(w780) -> ()
                n423 = local write "Trace"(w779) -> ()
                n424 = Close File(refnum=w778, error in=w777) -> (error out=w776:errorcluster)  [unwired: 1 out]
                n425 = Index Array(array=w750, index (dim 2)=0) -> (element=w747:u16[][])  [unwired: 2 in]
                n426 = Transpose 2D Array(2D array=w747) -> (transposed array=w745:u16[][])
                n427 = local write "Image"(w745) -> ()
              }
            }
          }
        }
      }
      event "Resolution", "Picture size", "Pixel time", "Picture size 2", "Axis", "Laser  Profile": Value Change {
        n428 = event-data() -> ()  [unwired: 1 in, 5 out]
        n429 = local read "Laser  Profile"() -> (w859:string)
        n430 = local read "Pixel time"() -> (w878:dbl)
        n431 = local read "Picture size"() -> (w877:dbl)
        n432 = local read "Picture size 2"() -> (w876:dbl)
        n433 = local read "X-Position"() -> (w872:dbl)
        n434 = local read "Axis"() -> (w875:enum32{"x-y", "x-z", "y-x", "y-z", "z-x", "z-y"})
        n435 = local read "Resolution"() -> (w869:dbl)
        n436 = local read "Y-Position"() -> (w871:dbl)
        n437 = local read "Z-Position"() -> (w870:dbl)
        n438 = String To Byte Array(string=w859) -> (unsigned byte array=w857:u8[])
        n439 = Array Size(array=w857) -> (size(s)=w856:i32)
        n440 = Subtract(x=w857, y=48) -> (x-y=w863:i32[])
        n441 = Initialize Array(4, w856) -> (w867:i32[])
        n442 = Initialize Array(1, w856) -> (w865:i32[])
        n443 = call "PI_CheckScan.vi"("Picture size"=w877, "Picture size 2"=w876, "Axis"=w875, "x-Position"=w872, "y-Position"=w871, "z-Position"=w870) -> ("Picture size out"=w873:dbl, "Picture size out 2"=w874:dbl)  [unwired: 8 in, 4 out]
        n444 = In Range and Coerce(upper limit=w867, x=w863, lower limit=w865) -> (coerced(x)=w860:i32[])  [unwired: 1 out]
        n445 = local write "Pixel time"(w878) -> ()
        n446 = local write "Picture size"(w873) -> ()
        n447 = local write "Picture size 2"(w874) -> ()
        n448 = local write "Axis"(w875) -> ()
        n449 = Add(x=w860, y=48) -> (x+y=w862:i32[])
        n450 = Byte Array To String(unsigned byte array=w862) -> (string=w858:string)
        n451 = while {
          shift-right: [w887] -> w855
          shift-left: w858 -> [w891]
          i -> [w883]
          stop <- w886 stop-if-true
          n452 = String Subset(string=w891, offset (0)=w883, length (rest)=1) -> (substring=w889:string)
          n453 = Increment(x=w883) -> (x+1=w884:i32)
          n454 = Search and Replace String(replace all?=TRUE, input string=w891, search string=w889, offset=w884) -> (result string=w887:string)  [unwired: 4 in, 3 out]
          n455 = String Length(string=w887) -> (length=w885:i32)
          n456 = Less?(x=w885, y=w883) -> (x < y?=w886:bool)
        }
        n457 = Divide(x=w873, y=w869) -> (x/y=w881:dbl)
        n458 = Divide(x=w874, y=w869) -> (x/y=w882:dbl)
        n459 = Round Toward +Infinity(x=w881) -> (ceil(x): smallest int >= x=→"x":dbl)
        n460 = Round Toward +Infinity(x=w882) -> (ceil(x): smallest int >= x=→"y":dbl)
        n461 = local write "Laser  Profile"(w855) -> ()
      }
      event "Power Button": Value Change {
        w897 = T29."Enabled" ("Disabled")
        w902 = T29."Disabled" ("Disabled")
        n462 = event-data() -> ()  [unwired: 1 in, 5 out]
        n463 = property on="Power Button" class="Bool (strict)"(error in=w901, "DisabledEnum"=w902) -> (error out=w895:errorcluster)  [unwired: 1 in, 1 out]
        n464 = property on="Power" class="Knob (strict)"(error in=w895, "DisabledEnum"=w902) -> (error out=w894:errorcluster)  [unwired: 1 in, 1 out]
        n465 = case shown="False" "is on?" {
          tunnel: w894 -> [w905 w931]
          tunnel: w893 -> [w904 w930]
          tunnel: [w903 w929] -> w896
          frame True {
            n466 = stacked-sequence {
              seq-local: [w906 _] -> [_ w926]
              tunnel: w905 -> [w911 _]
              tunnel: w904 -> [w910 _]
              tunnel: [_ w926] -> w903
              frame #0 {
                n467 = local read "Power"() -> (w908:dbl)
                n468 = Multiply(x=15, y=w908) -> (x*y=w907:dbl)
                n469 = for {
                  N: w907 -> [_]
                  shift-right: [w915] -> w906
                  shift-left: w911 -> [w917]
                  tunnel: w910 -> [w916]
                  tunnel: w907 -> [w912]
                  i -> [w914]
                  n470 = Subtract(x=w912, y=w914) -> (x-y=w913:dbl)
                  n471 = Wait (ms)(milliseconds to wait=u32 600) -> ()  [unwired: 1 out]
                  n472 = Format Value(format string="q=%d\n", value (0)=w913) -> (output string=w918:string)  [unwired: 1 in]
                  n473 = while {
                    tunnel: w918 -> [w925]
                    tunnel: w917 -> [w924]
                    tunnel: w916 -> [w923]
                    tunnel: [w922] -> w915
                    stop <- w921 continue-if-true
                    n474 = call "Query_laser.vi"("error in (no error)"=w924, "String in"=w925, "VISA resource name"=w923) -> ("error out"=w922:errorcluster, "was busy?"=w921:bool)  [unwired: 4 in, 2 out]
                  }
                }
              }
              frame #1 {
                n475 = local write "is on?"(FALSE) -> ()
                n476 = local write "Global Stop"(FALSE) -> ()
              }
            }
          }
          frame False {
            n477 = stacked-sequence {
              tunnel: w931 -> [w934 _]
              tunnel: w930 -> [w933 _]
              tunnel: [w932 _] -> w929
              frame #0 {
                n478 = for {
                  N: 1500 -> [_]
                  shift-right: [w937] -> w932
                  shift-left: w934 -> [w939]
                  tunnel: w933 -> [w940]
                  i -> [w936]
                  n479 = Wait (ms)(milliseconds to wait=u32 600) -> ()  [unwired: 1 out]
                  n480 = Format Value(format string="q=%d\n", value (0)=w936) -> (output string=w938:string)  [unwired: 1 in]
                  n481 = while {
                    tunnel: w940 -> [w947]
                    tunnel: w939 -> [w946]
                    tunnel: w938 -> [w945]
                    tunnel: [w944] -> w937
                    stop <- w943 continue-if-true
                    n482 = call "Query_laser.vi"("error in (no error)"=w946, "String in"=w945, "VISA resource name"=w947) -> ("error out"=w944:errorcluster, "was busy?"=w943:bool)  [unwired: 4 in, 2 out]
                  }
                }
              }
              frame #1 {
                n483 = local write "is on?"(TRUE) -> ()
              }
            }
          }
        }
        n484 = property on="Power Button" class="Bool (strict)"(error in=w896, "DisabledEnum"=w897) -> (error out=w898:errorcluster)  [unwired: 1 in, 1 out]
        n485 = property on="Power" class="Knob (strict)"(error in=w898, "Value"=100.0 ("Power"), "DisabledEnum"=w897) -> (error out=w892:errorcluster)  [unwired: 1 in, 1 out]
      }
      event "Power": Value Change {
        n486 = event-data() -> ()  [unwired: 1 in, 5 out]
        n487 = local read "is on?"() -> (w949:bool)
        n488 = case shown="False" w949 {
          tunnel: w952 -> [_ w957]
          tunnel: w951 -> [_ w956]
          tunnel: [_ w955] -> w950
          frame False {
          }
          frame True {
            n489 = local read "Power set"() -> (w953:dbl)
            n490 = local read "Power"() -> (w954:dbl)
            n491 = Multiply(x=15, y=w953) -> (x*y=w962:dbl)
            n492 = Multiply(x=w954, y=15) -> (x*y=w961:dbl)
            n493 = Subtract(x=w962, y=w961) -> (x-y=w960:dbl)
            n494 = Sign(1:w960) -> (0:w963:dbl)
            n495 = while {
              tunnel: w956 -> [w971]
              tunnel: w957 -> [w970]
              tunnel: w961 -> [w968]
              shift-right: [w965] -> _
              shift-left: w962 -> [w967]
              tunnel: w963 -> [w966]
              tunnel: [w964] -> w955
              stop <- w969 stop-if-true
              n496 = Subtract(x=w967, y=w966) -> (x-y=w965:dbl)
              n497 = Format Value(format string="q=%d\n", value (0)=w965) -> (output string=w973:string)  [unwired: 1 in]
              n498 = call "Query_laser.vi"("error in (no error)"=w970, "String in"=w973, "VISA resource name"=w971) -> ("error out"=w964:errorcluster)  [unwired: 4 in, 3 out]
              n499 = Equal?(x=w965, y=w968) -> (x = y?=w969:bool)
              n500 = Wait (ms)(milliseconds to wait=u32 600) -> ()  [unwired: 1 out]
            }
          }
        }
      }
    }
    "z-position" <- w346
    "y-position" <- w329
    "x-position" <- w345
    n501 = local read "Global Stop"() -> (w362:bool)
  }
  n502 = flat-sequence {
    tunnel: [w991] -> w27
    tunnel: [w995] -> w26
    tunnel: [w988] -> w25
    tunnel: w2 -> [w975]
    tunnel: w27 -> [w1016]
    tunnel: [w1016] -> w24
    tunnel: w21 -> [w1020]
    tunnel: w15 -> [w1019]
    tunnel: w19 -> [w1018]
    tunnel: w20 -> [w1017]
    tunnel: w26 -> [w1014]
    tunnel: w25 -> [w1015]
    tunnel: [w1015] -> w23
    tunnel: [w1014] -> w22
    tunnel: "Please enter a new prefix." ("message") -> [w1013]
    tunnel: "Must be in trapping mode for data storage." ("message") -> [w1012]
    tunnel: "Scan Frequency: %f Hz\nBin Period: %f ns\nScan Form: %s\nPoints Per Scan: %d\nPoint Spacing: %f um\nSub-Bin Delay: %f ns\nBeam Waist: %f um\nEOD Scale: %f um/V\nDiffusion Constant: %f um^2/s\nMobility: %f um/s/V\nMaximum Feedback: %f V\nInclude Mobility Update: %s\n" ("format string") -> [w1011]
    tunnel: w11 -> [w1010]
    tunnel: "Modulation Frequency: %f Hz\nNumber of Modulation Points: %d\nModulation Radius: %f um\nModulation Angle: %f degrees\n" ("format string") -> [w1009]
    tunnel: "Calibration forbidden when modulation is turned on." ("message") -> [w1008]
    tunnel: "Please set the recording time to a positive value." ("message") -> [w1007]
    tunnel: w24 -> [w2284]
    tunnel: w23 -> [w2281]
    tunnel: w22 -> [w2280]
    frame #0 {
      # "No datafile loaded yet"
      # "Available space for data received\nfrom the FPGA. Generally the CPU\nis fast enough to avoid backlogs."
      # "Number of commands that\ncould pile up at the FPGA\nwithout causing problems"
      # "Currently no data in the FPGA - no points, no voltages"
      # "Indicates a mistake in the commands sent to the FPGA (i.e. programmer error)"
      # "DMA is currently empty, so no overflow has occurred yet"
      # "Settings have not yet been sent to FPGA, so values in memory are unreliable"
      # "Not currently recording data"
      # "Initialize Variables"
      n503 = xnode "FPGA Open VI Reference"("error in"=w975) -> ("FPGA VI Reference Out"=w1005:refnum<k20>)  [unwired: 1 in, 1 out]
      n504 = xnode "Invoke Method"("FPGA VI Reference In"=w1005, "Depth"=u32 1024) -> ("FPGA VI Reference Out"=w1003:refnum<k20>)  [unwired: 1 in, 1 out]
      n505 = local write "Estimate Trap Time"(FALSE ("Estimate Trap Time")) -> ()
      n506 = local write "Currently Trapped"(FALSE ("Currently Trapped")) -> ()
      n507 = local write "Trap"(FALSE ("Trap")) -> ()
      n508 = local write "Record"(FALSE ("Record")) -> ()
      n509 = local write "Photon"(0.0 ("DMA Use")) -> ()
      n510 = local write "Feedback"(0.0 ("DMA Use")) -> ()
      n511 = Initialize Array(0.0 ("element"), 2 ("dimension size"), 0 ("dimension size")) -> (→"Current Voltages":dbl[][])
      n512 = Obtain Notifier(name (unnamed)="scan", notification data type=T10 [] ("appended array")) -> (notifier out=w988:refnum<notifier>)  [unwired: 2 in, 2 out]
      n513 = Obtain Notifier(name (unnamed)="datafile", notification data type=T30 {"Photon File"=refnum, "Feedback File"=refnum}) -> (notifier out=w995:refnum<notifier>)  [unwired: 2 in, 2 out]
      n514 = xnode "Invoke Method"("FPGA VI Reference In"=w1003, "Depth"=u32 1048576) -> ("FPGA VI Reference Out"=w992:refnum<k20>)  [unwired: 1 in, 1 out]
      n515 = xnode "Invoke Method"("FPGA VI Reference In"=w992, "Depth"=u32 1048576) -> ("FPGA VI Reference Out"=w981:refnum<k20>)  [unwired: 1 in, 1 out]
      n516 = xnode "Invoke Method"("FPGA VI Reference In"=w981) -> ("FPGA VI Reference Out"=w980:refnum<k20>)  [unwired: 1 in, 1 out]
      n517 = xnode "Invoke Method"("FPGA VI Reference In"=w980) -> ("FPGA VI Reference Out"=w979:refnum<k20>)  [unwired: 1 in, 1 out]
      n518 = xnode "Invoke Method"("FPGA VI Reference In"=w979) -> ("FPGA VI Reference Out"=w991:refnum<k20>)  [unwired: 2 in, 1 out]
      "Ready" <- FALSE ("Ready")
      "Unrecognized Command" <- FALSE ("Incorrect Command")
      "Photon DMA Overflow" <- FALSE ("Overflow")
      "Feedback DMA Overflow" <- FALSE ("Feedback DMA Overflow")
      "On-Chip FIFO Overflow" <- FALSE ("On-Chip FIFO Overflow")
    }
    frame #1 {
      n519 = while {
        tunnel: w1014 -> [w1024]
        tunnel: w1016 -> [w1023]
        tunnel: w1015 -> [w1022]
        stop <- w1021 stop-if-true
        n520 = event shown="[0] \"Trap\": Value Change" {
          selector: _ -> [_]
          dyn-events: _ -> [_]
          timeout: _ -> [_]
          tunnel: w1024 -> [w1063]
          tunnel: w1023 -> [w1047]
          tunnel: w1022 -> [w1055]
          tunnel: [w1025] -> w1021
          event "Trap": Value Change {
            w1036 = u16 0  # Number of Trapping Events
            w1035 = 0.0  # Total Time Trapped (s)
            w1037 = 0.0  # Time Recorded (s)
            w1038 = dbl[] []
            w1048 = TRUE  # Not reached end of recording length?
            w1034 = FALSE
            w1050 = refnum<k0> refnum  # Feedback File
            w1061 = refnum<k0> refnum  # Photon File
            w1062 = FALSE  # Recording?
            n521 = event-data() -> ()  [unwired: 1 in, 1 out]
            n522 = xnode "Invoke Method"("FPGA VI Reference In"=w1047, "Number of Elements"=u32 0, "Timeout (ms)"=-1) -> ("FPGA VI Reference Out"=w1046:refnum<k20>, "Elements Remaining"=w1042:u32)  [unwired: 1 in, 2 out]
            n523 = call-poly <vilib>:"DAQmx Create Virtual Channel.vi"("frequency"=20000.0, "duty cycle"=0.5, "counter"=tag "Dev1/ctr6") -> ("task out"=w1030:refnum<k21>, "error out"=w1029:errorcluster)  [unwired: 11 in]
            n524 = xnode "Invoke Method"("FPGA VI Reference In"=w1046, "Number of Elements"=u32 0, "Timeout (ms)"=-1) -> ("FPGA VI Reference Out"=w1045:refnum<k20>, "Elements Remaining"=w1041:u32)  [unwired: 1 in, 2 out]
            n525 = Tick Count (ms)() -> (millisecond timer value=w1058:u32)
            n526 = while {
              shift-right: [w1104] -> w1056
              shift-left: w1042 -> [w1124]
              shift-right: [w1119] -> w1059
              shift-left: w1061 -> [w1118]
              tunnel: w1063 -> [w1085]
              shift-right: [w1117] -> w1060
              shift-left: w1062 -> [w1086]
              tunnel: w1058 -> [w1111]
              shift-right: [w1098] -> w1052
              shift-left: w1041 -> [w1103]
              tunnel: w1055 -> [w1101]
              shift-right: [w1097] -> w1054
              shift-left: w1045 -> [w1125]
              shift-right: [w1075] -> w1033
              shift-left: w1034 -> [_]
              shift-left: w1034 -> [w1095]
              shift-right: [w1093] -> w1049
              shift-left: w1050 -> [w1094]
              border: w1038 -> [_]
              border: w1038 -> [_]
              border: w1038 -> [_]
              border: w1038 -> [_]
              border: w1048 -> [_]
              border: w1037 -> [_]
              border: w1035 -> [_]
              border: w1036 -> [_]
              stop <- w1095 stop-if-true
              # "Delay ending by two cycles\nto allow FIFO to clear out"
              n527 = flat-sequence {
                tunnel: w1114 -> [w1135]
                tunnel: [w1134] -> w1113
                tunnel: [w1130] -> w1112
                tunnel: w1111 -> [w1127]
                tunnel: ["Estimate Trap Time"] -> w1089
                tunnel: w1125 -> [w1232]
                tunnel: w1124 -> [w1190]
                tunnel: [w1231] -> w1104
                tunnel: [w1226] -> w1123
                tunnel: [w1225] -> w1122
                tunnel: w1121 -> [w1224]
                tunnel: w1120 -> [w1223]
                tunnel: [w1219] -> w1119
                tunnel: w1118 -> [w1143]
                tunnel: w1086 -> [w1145]
                tunnel: [w1139] -> w1117
                tunnel: w1113 -> [w1217]
                tunnel: w1112 -> [w1218]
                tunnel: w1110 -> [w1215]
                tunnel: [w1155] -> w1109
                tunnel: [w1211] -> w1108
                tunnel: w1107 -> [w1207]
                tunnel: w1106 -> [w1206]
                tunnel: [w1189] -> w1105
                tunnel: w1103 -> [w1196]
                tunnel: [w1154] -> w1098
                tunnel: [w1188] -> w1102
                tunnel: w1101 -> [w1186]
                tunnel: [w1179] -> w1097
                tunnel: w1094 -> [w1144]
                tunnel: [w1171] -> w1093
                tunnel: [w1165] -> w1092
                tunnel: w1091 -> [w1164]
                tunnel: [w1161] -> w1082
                tunnel: w1083 -> [w1138]
                tunnel: [w1160] -> w1090
                tunnel: w1089 -> [w1159]
                tunnel: [w1159] -> w1088
                tunnel: w1087 -> [w1158]
                tunnel: [w1152] -> w1080
                tunnel: w1081 -> [w1151]
                tunnel: [w1150] -> w1079
                tunnel: w1078 -> [w1149]
                tunnel: [w1148] -> w1076
                tunnel: w1077 -> [w1147]
                tunnel: w1085 -> [w1146]
                tunnel: w1084 -> [w1142]
                frame #0 {
                  n528 = Wait Until Next ms Multiple(millisecond multiple="Update Period (ms)") -> (millisecond timer value=w1128:u32)
                  n529 = Subtract(x=w1128, y=w1127) -> (x-y=w1129:u32)
                  n530 = Divide(x=w1129, y=1000.0) -> (x/y=w1132:dbl)
                  n531 = Subtract(x=w1132, y="Time to Show (s)") -> (x-y=w1130:dbl)
                  n532 = Insert Into Array(array=w1135, new element=w1132) -> (w1134:dbl[])  [unwired: 1 in]
                }
                frame #1 {
                  # "Scans apart"
                  # "Bins apart"
                  # "# photons"
                  n533 = case shown="False" w1145 {
                    tunnel: w1146 -> [w1243 _]
                    tunnel: w1144 -> [w1241 w1258]
                    tunnel: w1143 -> [w1240 w1257]
                    tunnel: w1142 -> [_ w1259]
                    tunnel: [w1238 w1256] -> w1141
                    tunnel: [w1239 w1255] -> w1140
                    tunnel: [w1236 w1254] -> w1139
                    tunnel: w1138 -> [w1235 w1253]
                    tunnel: [w1234 w1253] -> w1137
                    frame False {
                      # "Not recording at the moment - see if should start"
                      n534 = Wait on Notification(notifier=w1243, timeout in ms (-1)=0) -> (notifier out=w1233:refnum<notifier>, notification=w1242:T30, timed out?=w1237:bool)  [unwired: 2 in, 1 out]
                      n535 = Not(x=w1237) -> (.not. x?=w1236:bool)
                      n536 = case shown="False" w1236 {
                        tunnel: w1242 -> [_ w1252]
                        tunnel: [w1246 w1251] -> w1238
                        tunnel: [w1247 w1250] -> w1239
                        tunnel: w1241 -> [w1247 _]
                        tunnel: w1240 -> [w1246 _]
                        tunnel: [w1245 0.0] -> w1234
                        tunnel: w1235 -> [w1245 _]
                        tunnel: w1233 -> [_ w1248]
                        frame False {
                        }
                        frame True {
                          # "New data files"
                          n537 = Cancel Notification(0:w1248) -> ()  [unwired: 1 in, 3 out]
                          n538 = Unbundle(w1252) -> ("Photon File"=w1251:refnum<file>, "Feedback File"=w1250:refnum<file>)
                        }
                      }
                    }
                    frame True {
                      # "Currently recording - stop if button depressed or time up"
                      n539 = And(x="Record", y=w1259) -> (x .and. y?=w1254:bool)
                      n540 = local write "Record"(w1254) -> ()
                      n541 = case shown="True" w1254 {
                        tunnel: w1258 -> [w1264 w1266]
                        tunnel: w1257 -> [w1263 w1265]
                        tunnel: [refnum<k0> refnum w1265] -> w1256
                        tunnel: [refnum<k0> refnum w1266] -> w1255
                        frame False {
                          n542 = Close File(refnum=w1263) -> ()  [unwired: 1 in, 2 out]
                          n543 = Close File(refnum=w1264) -> ()  [unwired: 1 in, 2 out]
                        }
                        frame True {
                        }
                      }
                    }
                  }
                  n544 = Threshold 1D Array(2:w1218, 3:w1217) -> (0:w1208:dbl)  [unwired: 1 in]
                  n545 = local read "Current Number of Points per Scan"() -> (w1192:u8)
                  n546 = Delete From Array(array=w1217, length=w1208, index=0) -> (array with subset deleted=w1155:dbl[])  [unwired: 1 out]
                  n547 = local read "Current EOD Deflection Scale (um/V)"() -> (w1173:dbl)
                  n548 = xnode "Invoke Method"("FPGA VI Reference In"=w1232, "Number of Elements"=w1190, "Timeout (ms)"=0) -> ("FPGA VI Reference Out"=w1195:refnum<k20>, "Data"=w1180:u32[], "Elements Remaining"=w1231:u32)  [unwired: 1 in, 1 out]
                  n549 = Decrement(x=w1190) -> (x-1=w1229:u32)
                  n550 = Divide(x=w1173, y=3276.8) -> (x/y=w1172:dbl)
                  n551 = Quotient & Remainder(x=w1196, y=u32 4) -> (x-y*floor(x/y)=w1197:u32)  [unwired: 1 out]
                  n552 = Split Number(x=w1180) -> (hi(x)=w1201:u16[], lo(x)=w1202:u16[])
                  n553 = Subtract(x=w1196, y=w1197) -> (x-y=w1194:u32)
                  n554 = xnode "Invoke Method"("FPGA VI Reference In"=w1195, "Number of Elements"=w1194) -> ("FPGA VI Reference Out"=w1179:refnum<k20>, "Data"=w1170:u32[], "Elements Remaining"=w1154:u32)  [unwired: 2 in, 1 out]
                  n555 = Split Number(x=w1202) -> (hi(x)=w1200:u8[], lo(x)=w1199:u8[])
                  n556 = To Unsigned Long Integer(number=w1199) -> (unsigned 32bit integer=w1230:u32[])
                  n557 = Index Array(array=w1201, index=w1229) -> (element=w1226:u16)
                  n558 = Index Array(array=w1200, index=w1229) -> (element=w1225:u8)
                  n559 = local read "Current Scan Frequency (Hz)"() -> (w1163:dbl)
                  n560 = Add Array Elements(numeric array=w1230) -> (sum=w1162:u32)
                  n561 = Subtract(x=w1226, y=w1224) -> (x-y=w1220:u16)
                  n562 = Subtract(x=w1225, y=w1223) -> (x-y=w1222:u8)
                  n563 = Decimate 1D Array(w1170) -> (w1178:u32[], w1176:u32[])  [unwired: 2 out]
                  n564 = To Byte Integer(number=w1222) -> (8bit integer=w1221:i8)
                  n565 = To Long Integer(number=w1178) -> (32bit integer=w1177:i32[])
                  n566 = To Long Integer(number=w1176) -> (32bit integer=w1175:i32[])
                  n567 = Divide(x=w1221, y=w1192) -> (x/y=w1228:dbl)
                  n568 = call <vilib>:"Mean.vi"("X"=w1177) -> ("mean"=w1193:dbl)  [unwired: 1 out]
                  n569 = call <vilib>:"Mean.vi"("X"=w1175) -> ("mean"=w1191:dbl)  [unwired: 1 out]
                  n570 = Add(x=w1220, y=w1228) -> (x+y=w1227:dbl)
                  n571 = Multiply(x=w1193, y=w1172) -> (x*y=w1169:dbl)
                  "x Estimate" <- w1169
                  n572 = Multiply(x=w1191, y=w1172) -> (x*y=w1168:dbl)
                  "y Estimate" <- w1168
                  n573 = Divide(x=w1227, y=w1163) -> (x/y=w1153:dbl)
                  n574 = case shown="True" w1139 {
                    tunnel: [w1302 w1319] -> w1219
                    tunnel: w1141 -> [w1302 w1305]
                    tunnel: w1180 -> [_ w1316]
                    tunnel: w1140 -> [w1301 w1304]
                    tunnel: [w1301 w1313] -> w1171
                    tunnel: w1170 -> [_ w1312]
                    tunnel: w1153 -> [_ w1307]
                    tunnel: [w1300 w1306] -> w1161
                    tunnel: w1137 -> [w1300 w1303]
                    tunnel: [TRUE w1308] -> w1160
                    frame False {
                      # "Not in record mode"
                    }
                    frame True {
                      n575 = Add(x=w1307, y=w1303) -> (x+y=w1306:dbl)
                      "Time Recorded (s)" <- w1306
                      n576 = Write to Binary File(file (use dialog)=w1305, data=w1316, 5:FALSE ("prepend array or string size? (T)"), 9:T31."native, host order" ("byte order (0:big-endian, network order)")) -> (refnum out=w1319:refnum<file>)  [unwired: 2 in, 2 out]
                      n577 = Write to Binary File(file (use dialog)=w1304, data=w1312, 5:FALSE ("prepend array or string size? (T)"), 9:T31."native, host order" ("byte order (0:big-endian, network order)")) -> (refnum out=w1313:refnum<file>)  [unwired: 2 in, 2 out]
                      n578 = Less?(x=w1306, y="Time to Record (s)") -> (x < y?=w1310:bool)
                      n579 = Less Than 0?(x="Time to Record (s)") -> (x < 0?=w1309:bool)
                      n580 = Or(x=w1310, y=w1309) -> (x .or. y?=w1308:bool)
                    }
                  }
                  n581 = Delete From Array(array=w1215, length=w1208, index=0) -> (array with subset deleted=w1212:dbl[])  [unwired: 1 out]
                  n582 = Divide(x=w1162, y=w1153) -> (x/y=w1157:dbl)
                  n583 = Greater Or Equal?(x=w1157, y="Threshold (Hz)") -> (x >= y?=w1148:bool)
                  "Currently Trapped" <- w1148
                  n584 = Insert Into Array(array=w1212, new element=w1157) -> (w1211:dbl[])  [unwired: 1 in]
                  n585 = Build Array(w1169) -> (w1183:dbl[])
                  n586 = Build Array(w1168) -> (w1182:dbl[])
                  n587 = case shown="True" w1159 {
                    tunnel: w1158 -> [_ w1279]
                    tunnel: w1148 -> [_ w1278]
                    tunnel: w1153 -> [_ w1276]
                    tunnel: [w1268 w1273] -> w1150
                    tunnel: [w1267 w1272] -> w1152
                    tunnel: w1151 -> [w1267 w1271]
                    tunnel: w1149 -> [w1268 w1270]
                    tunnel: w1147 -> [_ w1269]
                    frame False {
                      # "Not recording trapping time"
                    }
                    frame True {
                      n588 = case shown="False" w1279 {
                        tunnel: [w1295 w1297] -> w1277
                        tunnel: [w1294 w1296] -> w1275
                        tunnel: [w1293 w1298] -> w1274
                        tunnel: w1271 -> [_ w1298]
                        tunnel: w1270 -> [_ w1297]
                        tunnel: w1269 -> [_ w1296]
                        frame False {
                          w1293 = u16 0  # Number of Trapping Events
                          w1294 = FALSE  # Currently Trapped
                          w1295 = 0.0  # Total Time Trapped (s)
                          # "Start recording trapping time"
                        }
                        frame True {
                          # "Continue recording\ntrapping time"
                        }
                      }
                      n589 = case shown="False" w1278 {
                        tunnel: w1277 -> [w1281 w1292]
                        tunnel: w1276 -> [_ w1291]
                        tunnel: w1275 -> [w1283 _]
                        tunnel: w1274 -> [w1282 w1289]
                        tunnel: [w1281 w1290] -> w1273
                        tunnel: [w1280 w1289] -> w1272
                        frame False {
                          n590 = case shown="True" w1283 {
                            tunnel: w1282 -> [w1284 w1288]
                            tunnel: w1281 -> [_ w1287]
                            tunnel: [w1284 w1285] -> w1280
                            frame False {
                            }
                            frame True {
                              # "Molecule just departed"
                              n591 = Increment(x=w1288) -> (x+1=w1285:u16)
                              "Number of Trapping Events" <- w1285
                              n592 = Divide(x=w1287, y=w1285) -> (x/y=→"Average Time Trapped (ms)":dbl)
                            }
                          }
                        }
                        frame True {
                          n593 = Add(x=w1292, y=w1291) -> (x+y=w1290:dbl)
                        }
                      }
                    }
                  }
                  n594 = Wait on Notification(notifier=w1186, timeout in ms (-1)=0) -> (notification=w1166:T10, timed out?=w1167:bool)  [unwired: 2 in, 2 out]
                  n595 = Select(t=w1164, s=w1167, f=w1166) -> (s? t:f=w1165:T10)
                  n596 = Delete From Array(array=w1207, length=w1208, index=0) -> (array with subset deleted=w1205:dbl[])  [unwired: 1 out]
                  n597 = Delete From Array(array=w1206, length=w1208, index=0) -> (array with subset deleted=w1204:dbl[])  [unwired: 1 out]
                  n598 = Bundle(w1155, w1211) -> (→"Recent Photon Count Rate":cluster{dbl[], dbl[]})  [unwired: 1 in]
                  n599 = Insert Into Array(array=w1205, new element=w1169) -> (w1189:dbl[])  [unwired: 1 in]
                  n600 = Insert Into Array(array=w1204, new element=w1168) -> (w1188:dbl[])  [unwired: 1 in]
                  n601 = Bundle(w1183, w1182) -> (w1184:cluster{dbl[], dbl[]})  [unwired: 1 in]
                  n602 = Bundle(w1189, w1188) -> (w1185:cluster{dbl[], dbl[]})  [unwired: 1 in]
                  n603 = Build Array (concatenate)(w1165, w1184, w1185) -> (→"Position Plot":T10)
                }
              }
              n604 = feedback-in #1(w1109) -> ()
              n605 = feedback #1() -> (w1114:dbl[])
              n606 = feedback-in #2(w1082) -> ()
              n607 = feedback #2() -> (w1083:dbl)
              n608 = feedback-in #3(w1088) -> ()
              n609 = feedback #3() -> (w1087:bool)  [unwired: 1 in]
              n610 = feedback-in #4(w1123) -> ()
              n611 = feedback #4() -> (w1121:u16)  [unwired: 1 in]
              n612 = feedback-in #5(w1122) -> ()
              n613 = feedback #5() -> (w1120:u8)  [unwired: 1 in]
              n614 = feedback-in #6(w1090) -> ()
              n615 = feedback #6() -> (w1084:bool)
              n616 = feedback-in #7(w1108) -> ()
              n617 = feedback #7() -> (w1110:dbl[])
              n618 = feedback-in #8(w1092) -> ()
              n619 = feedback #8() -> (w1091:T10)  [unwired: 1 in]
              n620 = feedback-in #9(w1079) -> ()
              n621 = feedback #9() -> (w1078:dbl)
              n622 = feedback-in #10(w1080) -> ()
              n623 = feedback #10() -> (w1081:u16)
              n624 = feedback-in #11(w1076) -> ()
              n625 = feedback #11() -> (w1077:bool)  [unwired: 1 in]
              n626 = feedback-in #12(w1102) -> ()
              n627 = feedback #12() -> (w1106:dbl[])
              n628 = feedback-in #13(w1105) -> ()
              n629 = feedback #13() -> (w1107:dbl[])
              n630 = Divide(x=w1104, y=1048576.0 ("Depth")) -> (x/y=→"Photon":dbl)
              n631 = Divide(x=w1098, y=1048576.0 ("Depth")) -> (x/y=→"Feedback":dbl)
              n632 = Not(x="Trap") -> (.not. x?=w1075:bool)
            }
            n633 = while {
              tunnel: w1033 -> [w1064]
              tunnel: [w1069] -> w1032
              tunnel: [w1068] -> w1031
              tunnel: w1030 -> [w1067]
              tunnel: w1029 -> [w1066]
              stop <- w1064 stop-if-true
              n634 = call <vilib>:"DAQmx Start Task.vi"("task/channels in"=w1067, "error in"=w1066) -> ("task out"=w1070:refnum<k21>, "error out"=w1071:errorcluster)  [unwired: 12 out]
              n635 = call <vilib>:"DAQmx Is Task Done.vi"("task/channels in"=w1070, "error in"=w1071) -> ("task out"=w1068:refnum<k21>, "error out"=w1069:errorcluster)  [unwired: 1 in, 11 out]
              n636 = Wait (ms)(milliseconds to wait=u32 100) -> ()  [unwired: 1 out]
            }
            n637 = call <vilib>:"DAQmx Clear Task.vi"("task in"=w1031, "error in"=w1032) -> ()  [unwired: 14 out]
            n638 = xnode "Invoke Method"("FPGA VI Reference In"=w1054, "Number of Elements"=w1056, "Timeout (ms)"=0) -> ("FPGA VI Reference Out"=w1053:refnum<k20>)  [unwired: 1 in, 3 out]
            n639 = case shown="True" w1060 {
              tunnel: w1059 -> [_ w1074]
              tunnel: w1049 -> [_ w1072]
              frame False {
              }
              frame True {
                # "Close data file if one existed\nTurn off record mode"
                n640 = Close File(refnum=w1072) -> ()  [unwired: 1 in, 2 out]
                n641 = local write "Record"(FALSE ("Record")) -> ()
                n642 = Close File(refnum=w1074) -> ()  [unwired: 1 in, 2 out]
              }
            }
            n643 = local read "Global Stop"() -> (w1025:bool)
            n644 = xnode "Invoke Method"("FPGA VI Reference In"=w1053, "Number of Elements"=w1052, "Timeout (ms)"=0) -> ()  [unwired: 1 in, 4 out]
          }
        }
      }
      n645 = while {
        tunnel: w1016 -> [w2256]
        stop <- w2251 stop-if-true
        n646 = flat-sequence {
          tunnel: w2256 -> [w2266]
          tunnel: [w2263] -> w2255
          tunnel: [w2262] -> w2253
          tunnel: w2255 -> [w2269]
          tunnel: [w2269] -> w2254
          tunnel: w2253 -> [w2268]
          tunnel: [w2268] -> w2252
          tunnel: w2254 -> [w2270]
          tunnel: w2252 -> [w2271]
          frame #0 {
            # "Check if any interrupts triggered\nRepeat every 500 ms"
            n647 = Build Array(0 ("element"), 1 ("element"), 6 ("element"), 7 ("element"), 8 ("element")) -> (w2264:i32[])
            n648 = xnode "Invoke Method"("FPGA VI Reference In"=w2266, "IRQ Number(s)"=w2264, "Timeout (ms)"=500) -> ("FPGA VI Reference Out"=w2262:refnum<k20>, "IRQ(s) Asserted"=w2263:i32[])  [unwired: 1 in, 2 out]
          }
          frame #1 {
            # "Clear these warnings if they\nwere set previously"
            "Mistimed" <- FALSE ("Mistimed")
          }
          frame #2 {
            # "Clear the interrupts that were triggered\nTurn on the corresponding error lights on the GUI"
            n649 = Array Size(array=w2270) -> (size(s)=w2272:i32)
            n650 = for {
              N: w2272 -> [_]
              tunnel: w2271 -> [w2274]
              tunnel: w2270 -> [w2273] mode=indexing
              n651 = xnode "Invoke Method"("FPGA VI Reference In"=w2274, "IRQ Number(s)"=w2273) -> ()  [unwired: 1 in, 2 out]
              n652 = case shown="6" w2273 {
                frame 0 {
                  # "Soft toggle - cleared after 0.5 s"
                  n653 = local write "Mistimed"(TRUE ("Overflow")) -> ()
                }
                frame 1, Default {
                  # "Hard toggle - stays on if ever on"
                  n654 = local write "Unrecognized Command"(TRUE ("Incorrect Command")) -> ()
                }
                frame 6 {
                  # "Hard toggle - stays on if ever on"
                  n655 = local write "On-Chip FIFO Overflow"(TRUE ("Mistimed")) -> ()
                }
                frame 7 {
                  # "Hard toggle - stays on if ever on"
                  n656 = local write "Photon DMA Overflow"(TRUE ("Mistimed")) -> ()
                }
                frame 8 {
                  # "Hard toggle - stays on if ever on"
                  n657 = local write "Feedback DMA Overflow"(TRUE ("Mistimed")) -> ()
                }
              }
            }
          }
        }
        n658 = local read "Global Stop"() -> (w2251:bool)
      }
      n659 = while {
        tunnel: w1016 -> [w1346]
        tunnel: w1020 -> [w1345]
        tunnel: w1019 -> [w1344]
        tunnel: w1018 -> [w1343]
        tunnel: w1017 -> [w1342]
        tunnel: w1014 -> [w1337]
        tunnel: w1015 -> [w1335]
        tunnel: w1013 -> [w1329]
        tunnel: w1012 -> [w1328]
        tunnel: w1011 -> [w1327]
        tunnel: w1010 -> [w1326]
        tunnel: w1009 -> [w1324]
        tunnel: w1008 -> [w1323]
        tunnel: w1007 -> [w1322]
        stop <- w1347 stop-if-true
        # "Inverse Diffusion Coefficient"
        # "Bin Length (ticks)"
        n660 = local read "Current Number of Points per Scan"() -> (w1338:u8)
        n661 = local read "Current Scan Frequency (Hz)"() -> (w1334:dbl)
        n662 = feedback #14() -> (w1332:u16)  [unwired: 1 in]
        n663 = feedback #15() -> (w1330:u32)  [unwired: 1 in]
        n664 = event shown="[10] \"Update FPGA\": Value Change" {
          selector: _ -> [_ _ _ _ _ _ _ _ _ _ _ _ _]
          dyn-events: _ -> [_ _ _ _ _ _ _ _ _ _ _ _ _]
          timeout: _ -> [_ _ _ _ _ _ _ _ _ _ _ _ _]
          tunnel: [_ _ _ _ _ _ _ _ _ _ _ _ w2250] -> w1347
          tunnel: w1346 -> [w1353 _ w1379 _ _ _ _ _ _ _ w1888 _ w2243]
          tunnel: w1345 -> [_ _ _ _ w1403 _ _ _ _ _ _ _ _]
          tunnel: w1344 -> [_ _ _ _ w1390 w1684 w1781 w1808 w1834 w1862 _ _ _]
          tunnel: w1343 -> [_ _ _ w1383 w1406 _ _ _ _ _ _ _ _]
          tunnel: w1342 -> [_ _ _ _ _ _ _ _ _ _ w1877 _ _]
          tunnel: "New Number of Points per Scan" -> [_ _ _ w1382 w1400 w1685 w1794 w1821 w1846 w1857 w1889 _ _]
          tunnel: "New Scan Frequency (Hz)" -> [_ _ _ _ w1401 _ _ _ _ _ w1886 _ _]
          tunnel: "New Spacing (um)" -> [_ _ _ _ w1399 w1683 _ _ w1840 w1858 w1891 _ _]
          tunnel: "New Scan Form" -> [_ _ _ _ w1402 _ w1795 w1822 w1845 w1856 w1890 _ _]
          tunnel: w1334 -> [_ _ _ _ _ _ _ _ _ _ _ w2129 _]
          tunnel: w1338 -> [_ _ _ _ _ _ _ _ _ _ w1887 w2128 _]
          tunnel: w1337 -> [_ _ _ _ _ _ _ _ _ _ _ w2127 _]
          tunnel: "New EOD Deflection Scale (um/V)" -> [_ _ _ _ w1392 w1680 w1783 w1811 _ w1854 w1885 _ _]
          tunnel: w1335 -> [_ _ _ _ _ _ _ _ _ _ w1884 _ _]
          tunnel: [w1349 w1363 w1378 w1381 w1395 w1678 w1786 w1813 w1842 w1851 w1874 w2126 w2241] -> w1333
          tunnel: w1332 -> [w1349 w1363 w1378 w1381 w1395 w1678 w1786 w1813 w1842 w1851 w1873 w2126 w2241]
          tunnel: [w1348 w1364 w1377 w1380 w1394 w1677 w1785 w1812 w1841 w1852 w1870 w2125 w2240] -> w1331
          tunnel: w1330 -> [w1348 w1364 w1377 w1380 w1394 w1677 w1785 w1812 w1841 w1852 w1869 w2125 w2240]
          tunnel: w1329 -> [_ _ _ _ _ _ _ _ _ _ _ w2123 _]
          tunnel: w1328 -> [_ _ _ _ _ _ _ _ _ _ _ w2124 _]
          tunnel: w1327 -> [_ _ _ _ _ _ _ _ _ _ _ w2122 _]
          tunnel: w1326 -> [_ _ _ _ _ _ _ _ _ _ w1868 _ _]
          tunnel: "New Modulation Radius (um)" -> [_ _ _ _ w1391 _ w1784 w1810 w1839 _ w1867 _ _]
          tunnel: w1324 -> [_ _ _ _ _ _ _ _ _ _ _ w2121 _]
          tunnel: w1323 -> [_ _ _ _ _ _ _ _ _ _ _ _ _]
          tunnel: w1322 -> [_ _ _ _ _ _ _ _ _ _ _ _ _]
          tunnel: "Prefix" -> [_ _ _ _ _ _ _ _ _ _ _ w2120 _]
          event "Trap": Value Change {
            # "If Ready (i.e. FPGA has been updated at least once), send a command to start or stop\nIf not Ready, then should not start yet, and no need to stop (since FPGA initializes to off)"
            n665 = event-data() -> ("NewVal"=w1352:bool)  [unwired: 1 in]
            n666 = local read "Ready"() -> (w1350:bool)
            n667 = And(x=w1350, y=w1352) -> (x .and. y?=w1351:bool)
            n668 = local write "Trap"(w1351) -> ()
            n669 = case shown="True" w1350 {
              tunnel: w1352 -> [_ w1356]
              tunnel: w1353 -> [_ w1355]
              frame False {
              }
              frame True {
                n670 = Join Numbers(hi=u8 1, lo=u8 0) -> ((hi.lo)=w1357:u16)
                n671 = Boolean To (0,1)(Boolean=w1356) -> (0, 1=w1362:i16)
                n672 = Join Numbers(hi=w1357, lo=w1362) -> ((hi.lo)=w1360:u32)
                n673 = Build Array(w1360) -> (w1361:u32[])
                n674 = xnode "Invoke Method"("FPGA VI Reference In"=w1355, "Data"=w1361, "Timeout (ms)"=-1) -> ()  [unwired: 1 in, 3 out]
              }
            }
          }
          event "Clear Warnings": Value Change {
            n675 = event-data() -> ()  [unwired: 1 in, 1 out]
            n676 = local write "Unrecognized Command"(FALSE ("Unrecognized Command")) -> ()
            n677 = local write "Photon DMA Overflow"(FALSE ("Photon DMA Overflow")) -> ()
            n678 = local write "On-Chip FIFO Overflow"(FALSE ("On-Chip FIFO Overflow")) -> ()
            n679 = local write "Feedback DMA Overflow"(FALSE ("Feedback DMA Overflow")) -> ()
          }
          event "Include Mobility Update": Value Change {
            n680 = event-data() -> ("NewVal"=w1369:bool)  [unwired: 1 in]
            n681 = Join Numbers(hi=u8 4, lo=u8 0) -> ((hi.lo)=w1371:u16)
            n682 = Boolean To (0,1)(Boolean=w1369) -> (0, 1=w1376:i16)
            n683 = Join Numbers(hi=w1371, lo=w1376) -> ((hi.lo)=w1374:u32)
            n684 = Build Array(w1374) -> (w1375:u32[])
            n685 = xnode "Invoke Method"("FPGA VI Reference In"=w1379, "Data"=w1375, "Timeout (ms)"=-1) -> ()  [unwired: 1 in, 3 out]
          }
          event "New Scan Frequency (Hz)": Value Change {
            # "Only allow the scan frequency to be changed if it does not max out.\nIf it does max out, then just set the frequency to the maximum allowed."
            n686 = event-data() -> ("NewVal"=w1386:dbl)  [unwired: 1 in]
            n687 = Multiply(x=w1386, y=w1382) -> (x*y=w1388:dbl)
            n688 = Less Or Equal?(x=w1388, y=w1383) -> (x <= y?=w1387:bool)
            n689 = Divide(x=w1383, y=w1382) -> (x/y=w1384:dbl)
            n690 = Select(t=w1386, s=w1387, f=w1384) -> (s? t:f=w1385:dbl)
            n691 = local write "New Scan Frequency (Hz)"(w1385) -> ()
          }
          event "New Number of Points per Scan": Value Change {
            # "Allow the number of points per scan to be changed, as long as\nit does not max out the scan frequency or the maximum voltage"
            n692 = event-data() -> ("NewVal"=w1404:u8)  [unwired: 1 in]
            n693 = Divide(x=w1391, y=w1392) -> (x/y=w1393:dbl)
            n694 = Divide(x=w1399, y=w1392) -> (x/y=w1398:dbl)
            n695 = Increment(x=w1400) -> (x+1=w1408:u8)
            n696 = Equal?(x=w1404, y=w1408) -> (x = y?=w1405:bool)
            n697 = Subtract(x=w1390, y=w1393) -> (x-y=w1389:dbl)
            n698 = case shown="False" w1405 {
              tunnel: w1402 -> [w1417 w1572]
              tunnel: [w1412 w1567] -> w1407
              tunnel: w1404 -> [w1415 w1570]
              tunnel: w1403 -> [w1414 w1569]
              tunnel: w1398 -> [w1416 w1571]
              tunnel: w1389 -> [w1413 w1568]
              tunnel: [w1411 w1566] -> w1397
              tunnel: w1401 -> [w1410 w1565]
              tunnel: w1406 -> [w1409 w1564]
              frame False {
                # "Go to largest allowable number of points less than or equal to the requested number of points,\nwithout saturating the Voltage nor the number of points nor the frequency"
                n699 = case shown="\"Square\"" w1417 {
                  selector: w1417 -> [w1422 w1452 w1487 w1524]
                  tunnel: w1416 -> [w1427 w1454 w1489 w1529]
                  tunnel: w1415 -> [w1426 w1462 w1497 w1528]
                  tunnel: w1414 -> [w1425 w1461 w1496 w1527]
                  tunnel: w1413 -> [w1424 w1460 w1495 w1526]
                  tunnel: [w1423 w1459 w1494 w1525] -> w1412
                  tunnel: [w1419 w1456 w1491 w1521] -> w1411
                  tunnel: w1410 -> [w1421 w1458 w1493 w1523]
                  tunnel: w1409 -> [w1420 w1457 w1492 w1522]
                  tunnel: [w1418 w1450 w1485 w1520] -> _
                  frame "Circular", Default {
                    n700 = while {
                      shift-right: [w1431] -> _
                      shift-left: u8 1 -> [w1434]
                      tunnel: w1427 -> [w1449]
                      tunnel: w1426 -> [w1448]
                      tunnel: w1425 -> [w1447]
                      tunnel: w1424 -> [w1446]
                      tunnel: [w1434] -> w1423
                      tunnel: w1422 -> [w1441]
                      tunnel: w1421 -> [w1440]
                      tunnel: w1420 -> [w1438]
                      shift-right: [w1433] -> _
                      shift-left: _ -> [w1432]
                      tunnel: [w1432] -> w1419
                      shift-right: [w1430] -> _
                      shift-left: _ -> [w1429]
                      tunnel: [w1429] -> w1418
                      stop <- w1442 stop-if-true
                      n701 = Increment(x=w1434) -> (x+1=w1431:u8)
                      n702 = call "CalculateRadius.vi"("Scan Type"=w1441, "Points per Scan"=w1431, "Spacing (V)"=w1449) -> ("Maximum Voltage (V)"=w1430:dbl, "Radius (V)"=w1433:dbl)
                      n703 = Greater?(x=w1431, y=w1447) -> (0:w1444:bool)
                      n704 = Multiply(x=w1431, y=w1440) -> (x*y=w1439:dbl)
                      n705 = Greater?(x=w1431, y=w1448) -> (0:w1445:bool)
                      n706 = Greater Or Equal?(x=w1430, y=w1446) -> (x >= y?=w1436:bool)
                      n707 = Greater?(x=w1439, y=w1438) -> (0:w1437:bool)
                      n708 = Or(x=w1445, y=w1444) -> (x .or. y?=w1443:bool)
                      n709 = Or(x=w1436, y=w1437) -> (x .or. y?=w1435:bool)
                      n710 = Or(x=w1443, y=w1435) -> (x .or. y?=w1442:bool)
                    }
                  }
                  frame "Square" {
                    w1453 = u8 1
                    n711 = call "CalculateRadius.vi"("Scan Type"=w1452, "Points per Scan"=w1453, "Spacing (V)"=w1454) -> ("Maximum Voltage (V)"=w1451:dbl, "Radius (V)"=w1455:dbl)
                    n712 = while {
                      shift-right: [w1465] -> _
                      shift-left: w1453 -> [w1475]
                      tunnel: w1454 -> [w1484]
                      tunnel: w1462 -> [w1483]
                      tunnel: w1461 -> [w1482]
                      tunnel: w1460 -> [w1481]
                      tunnel: [w1475] -> w1459
                      tunnel: w1452 -> [w1476]
                      tunnel: w1458 -> [w1473]
                      tunnel: w1457 -> [w1471]
                      shift-right: [w1467] -> _
                      shift-left: w1455 -> [w1466]
                      tunnel: [w1466] -> w1456
                      shift-right: [w1464] -> _
                      shift-left: w1451 -> [w1463]
                      tunnel: [w1463] -> w1450
                      stop <- w1477 stop-if-true
                      n713 = Add(x=w1475, y=u8 1) -> (x+y=w1465:u8)
                      n714 = call "CalculateRadius.vi"("Scan Type"=w1476, "Points per Scan"=w1465, "Spacing (V)"=w1484) -> ("Maximum Voltage (V)"=w1464:dbl, "Radius (V)"=w1467:dbl)
                      n715 = Greater?(x=w1465, y=w1482) -> (0:w1479:bool)
                      n716 = Multiply(x=w1465, y=w1473) -> (x*y=w1472:dbl)
                      n717 = Greater?(x=w1465, y=w1483) -> (0:w1480:bool)
                      n718 = Greater Or Equal?(x=w1464, y=w1481) -> (x >= y?=w1469:bool)
                      n719 = Greater?(x=w1472, y=w1471) -> (0:w1470:bool)
                      n720 = Or(x=w1480, y=w1479) -> (x .or. y?=w1478:bool)
                      n721 = Or(x=w1469, y=w1470) -> (x .or. y?=w1468:bool)
                      n722 = Or(x=w1478, y=w1468) -> (x .or. y?=w1477:bool)
                    }
                  }
                  frame "FilledSquare" {
                    w1488 = u8 4
                    n723 = call "CalculateRadius.vi"("Scan Type"=w1487, "Points per Scan"=w1488, "Spacing (V)"=w1489) -> ("Maximum Voltage (V)"=w1486:dbl, "Radius (V)"=w1490:dbl)
                    n724 = while {
                      shift-right: [w1500] -> _
                      shift-left: w1488 -> [w1510]
                      tunnel: w1489 -> [w1519]
                      tunnel: w1497 -> [w1518]
                      tunnel: w1496 -> [w1517]
                      tunnel: w1495 -> [w1516]
                      tunnel: [w1510] -> w1494
                      tunnel: w1487 -> [w1511]
                      tunnel: w1493 -> [w1508]
                      tunnel: w1492 -> [w1506]
                      shift-right: [w1502] -> _
                      shift-left: w1490 -> [w1501]
                      tunnel: [w1501] -> w1491
                      shift-right: [w1499] -> _
                      shift-left: w1486 -> [w1498]
                      tunnel: [w1498] -> w1485
                      stop <- w1512 stop-if-true
                      n725 = Add(x=w1510, y=u8 4) -> (x+y=w1500:u8)
                      n726 = call "CalculateRadius.vi"("Scan Type"=w1511, "Points per Scan"=w1500, "Spacing (V)"=w1519) -> ("Maximum Voltage (V)"=w1499:dbl, "Radius (V)"=w1502:dbl)
                      n727 = Greater?(x=w1500, y=w1517) -> (0:w1514:bool)
                      n728 = Multiply(x=w1500, y=w1508) -> (x*y=w1507:dbl)
                      n729 = Greater?(x=w1500, y=w1518) -> (0:w1515:bool)
                      n730 = Greater Or Equal?(x=w1499, y=w1516) -> (x >= y?=w1504:bool)
                      n731 = Greater?(x=w1507, y=w1506) -> (0:w1505:bool)
                      n732 = Or(x=w1515, y=w1514) -> (x .or. y?=w1513:bool)
                      n733 = Or(x=w1504, y=w1505) -> (x .or. y?=w1503:bool)
                      n734 = Or(x=w1513, y=w1503) -> (x .or. y?=w1512:bool)
                    }
                  }
                  frame "Hexagonal" {
                    n735 = while {
                      shift-right: [w1533] -> _
                      shift-left: u8 1 -> [w1554]
                      tunnel: w1529 -> [w1563]
                      tunnel: w1528 -> [w1562]
                      tunnel: w1527 -> [w1561]
                      tunnel: w1526 -> [w1560]
                      tunnel: [w1554] -> w1525
                      tunnel: w1524 -> [w1555]
                      tunnel: w1523 -> [w1553]
                      tunnel: w1522 -> [w1551]
                      shift-right: [w1535] -> _
                      shift-left: _ -> [w1534]
                      tunnel: [w1534] -> w1521
                      shift-right: [w1532] -> _
                      shift-left: _ -> [w1531]
                      tunnel: [w1531] -> w1520
                      i -> [w1547]
                      stop <- w1556 stop-if-true
                      n736 = To Unsigned Byte Integer(number=w1547) -> (unsigned 8bit integer=w1537:u8)
                      n737 = Multiply(x=w1537, y=w1537) -> (x*y=w1536:u8)
                      n738 = Multiply(x=w1537, y=u8 3) -> (x*y=w1538:u8)
                      n739 = Add(x=w1536, y=w1538) -> (x+y=w1539:u8)
                      n740 = Add(x=w1539, y=u8 2) -> (x+y=w1542:u8)
                      n741 = Quotient & Remainder(x=w1536, y=u8 4) -> (floor(x/y)=w1545:u8)  [unwired: 1 out]
                      n742 = Quotient & Remainder(x=w1542, y=u8 2) -> (floor(x/y)=w1546:u8)  [unwired: 1 out]
                      n743 = Add(x=w1545, y=w1546) -> (x+y=w1533:u8)
                      n744 = call "CalculateRadius.vi"("Scan Type"=w1555, "Points per Scan"=w1533, "Spacing (V)"=w1563) -> ("Maximum Voltage (V)"=w1532:dbl, "Radius (V)"=w1535:dbl)
                      n745 = Greater?(x=w1533, y=w1561) -> (0:w1558:bool)
                      n746 = Multiply(x=w1533, y=w1553) -> (x*y=w1552:dbl)
                      n747 = Greater?(x=w1533, y=w1562) -> (0:w1559:bool)
                      n748 = Greater Or Equal?(x=w1532, y=w1560) -> (x >= y?=w1549:bool)
                      n749 = Greater?(x=w1552, y=w1551) -> (0:w1550:bool)
                      n750 = Or(x=w1559, y=w1558) -> (x .or. y?=w1557:bool)
                      n751 = Or(x=w1549, y=w1550) -> (x .or. y?=w1548:bool)
                      n752 = Or(x=w1557, y=w1548) -> (x .or. y?=w1556:bool)
                    }
                  }
                }
              }
              frame True {
                # "Increment to the next allowed number of points, if possible"
                n753 = case shown="\"Circular\", Default" w1572 {
                  selector: w1572 -> [w1575 w1603 w1637]
                  tunnel: w1571 -> [w1581 w1605 w1636]
                  tunnel: w1570 -> [w1580 w1613 w1643]
                  tunnel: w1569 -> [w1579 w1612 w1642]
                  tunnel: w1568 -> [w1578 w1611 w1641]
                  tunnel: [w1574 w1608 w1638] -> w1567
                  tunnel: [w1573 w1607 w1635] -> w1566
                  tunnel: w1565 -> [w1577 w1610 w1640]
                  tunnel: w1564 -> [w1576 w1609 w1639]
                  frame "Circular", Default {
                    n754 = while {
                      shift-right: [w1584] -> _
                      shift-left: u8 1 -> [w1587]
                      tunnel: w1581 -> [w1602]
                      tunnel: w1580 -> [w1601]
                      tunnel: w1579 -> [w1600]
                      tunnel: w1578 -> [w1599]
                      tunnel: [w1587] -> w1574
                      tunnel: w1575 -> [w1594]
                      tunnel: w1577 -> [w1593]
                      tunnel: w1576 -> [w1591]
                      shift-right: [w1586] -> _
                      shift-left: _ -> [w1585]
                      tunnel: [w1585] -> w1573
                      stop <- w1595 stop-if-true
                      n755 = Increment(x=w1587) -> (x+1=w1584:u8)
                      n756 = call "CalculateRadius.vi"("Scan Type"=w1594, "Points per Scan"=w1584, "Spacing (V)"=w1602) -> ("Maximum Voltage (V)"=w1583:dbl, "Radius (V)"=w1586:dbl)
                      n757 = Greater?(x=w1584, y=w1600) -> (0:w1597:bool)
                      n758 = Multiply(x=w1584, y=w1593) -> (x*y=w1592:dbl)
                      n759 = Greater Or Equal?(x=w1587, y=w1601) -> (x >= y?=w1598:bool)
                      n760 = Greater Or Equal?(x=w1583, y=w1599) -> (x >= y?=w1589:bool)
                      n761 = Greater?(x=w1592, y=w1591) -> (0:w1590:bool)
                      n762 = Or(x=w1598, y=w1597) -> (x .or. y?=w1596:bool)
                      n763 = Or(x=w1589, y=w1590) -> (x .or. y?=w1588:bool)
                      n764 = Or(x=w1596, y=w1588) -> (x .or. y?=w1595:bool)
                    }
                  }
                  frame "Square" {
                    w1604 = u8 4
                    n765 = call "CalculateRadius.vi"("Scan Type"=w1603, "Points per Scan"=w1604, "Spacing (V)"=w1605) -> ("Radius (V)"=w1606:dbl)  [unwired: 1 out]
                    n766 = while {
                      shift-right: [w1615] -> _
                      shift-left: w1604 -> [w1618]
                      tunnel: w1605 -> [w1634]
                      tunnel: w1613 -> [w1633]
                      tunnel: w1612 -> [w1632]
                      tunnel: w1611 -> [w1631]
                      tunnel: [w1618] -> w1608
                      tunnel: w1603 -> [w1626]
                      tunnel: w1610 -> [w1624]
                      tunnel: w1609 -> [w1622]
                      shift-right: [w1617] -> _
                      shift-left: w1606 -> [w1616]
                      tunnel: [w1616] -> w1607
                      stop <- w1627 stop-if-true
                      n767 = Add(x=w1618, y=u8 4) -> (x+y=w1615:u8)
                      n768 = call "CalculateRadius.vi"("Scan Type"=w1626, "Points per Scan"=w1615, "Spacing (V)"=w1634) -> ("Maximum Voltage (V)"=w1614:dbl, "Radius (V)"=w1617:dbl)
                      n769 = Greater?(x=w1615, y=w1632) -> (0:w1629:bool)
                      n770 = Multiply(x=w1615, y=w1624) -> (x*y=w1623:dbl)
                      n771 = Greater Or Equal?(x=w1618, y=w1633) -> (x >= y?=w1630:bool)
                      n772 = Greater Or Equal?(x=w1614, y=w1631) -> (x >= y?=w1620:bool)
                      n773 = Greater?(x=w1623, y=w1622) -> (0:w1621:bool)
                      n774 = Or(x=w1630, y=w1629) -> (x .or. y?=w1628:bool)
                      n775 = Or(x=w1620, y=w1621) -> (x .or. y?=w1619:bool)
                      n776 = Or(x=w1628, y=w1619) -> (x .or. y?=w1627:bool)
                    }
                  }
                  frame "Hexagonal" {
                    n777 = while {
                      shift-right: [w1646] -> _
                      shift-left: u8 1 -> [w1649]
                      tunnel: w1636 -> [w1676]
                      tunnel: w1643 -> [w1675]
                      tunnel: w1642 -> [w1674]
                      tunnel: w1641 -> [w1673]
                      tunnel: [w1649] -> w1638
                      tunnel: w1637 -> [w1668]
                      tunnel: w1640 -> [w1667]
                      tunnel: w1639 -> [w1665]
                      shift-right: [w1648] -> _
                      shift-left: _ -> [w1647]
                      tunnel: [w1647] -> w1635
                      i -> [w1661]
                      stop <- w1669 stop-if-true
                      n778 = To Unsigned Byte Integer(number=w1661) -> (unsigned 8bit integer=w1650:u8)
                      n779 = Multiply(x=w1650, y=w1650) -> (x*y=w1651:u8)
                      n780 = Multiply(x=w1650, y=u8 3) -> (x*y=w1652:u8)
                      n781 = Add(x=w1651, y=w1652) -> (x+y=w1653:u8)
                      n782 = Add(x=w1653, y=u8 2) -> (x+y=w1656:u8)
                      n783 = Quotient & Remainder(x=w1651, y=u8 4) -> (floor(x/y)=w1659:u8)  [unwired: 1 out]
                      n784 = Quotient & Remainder(x=w1656, y=u8 2) -> (floor(x/y)=w1660:u8)  [unwired: 1 out]
                      n785 = Add(x=w1659, y=w1660) -> (x+y=w1646:u8)
                      n786 = call "CalculateRadius.vi"("Scan Type"=w1668, "Points per Scan"=w1646, "Spacing (V)"=w1676) -> ("Maximum Voltage (V)"=w1645:dbl, "Radius (V)"=w1648:dbl)
                      n787 = Greater?(x=w1646, y=w1674) -> (0:w1671:bool)
                      n788 = Multiply(x=w1646, y=w1667) -> (x*y=w1666:dbl)
                      n789 = Greater Or Equal?(x=w1649, y=w1675) -> (x >= y?=w1672:bool)
                      n790 = Greater Or Equal?(x=w1645, y=w1673) -> (x >= y?=w1663:bool)
                      n791 = Greater?(x=w1666, y=w1665) -> (0:w1664:bool)
                      n792 = Or(x=w1672, y=w1671) -> (x .or. y?=w1670:bool)
                      n793 = Or(x=w1663, y=w1664) -> (x .or. y?=w1662:bool)
                      n794 = Or(x=w1670, y=w1662) -> (x .or. y?=w1669:bool)
                    }
                  }
                }
              }
            }
            n795 = Multiply(x=w1397, y=w1392) -> (x*y=w1396:dbl)
            n796 = local write "New Number of Points per Scan"(w1407) -> ()
            n797 = local write "New Radius (um)"(w1396) -> ()
          }
          event "New Scan Form": Value Change {
            # "Should always end up with fewer points, so no concern about frequency or number of points saturating"
            n798 = event-data() -> ("NewVal"=w1686:T7)  [unwired: 1 in]
            n799 = Divide(x=w1683, y=w1680) -> (x/y=w1682:dbl)
            n800 = case shown="\"FilledSquare\"" w1686 {
              selector: w1686 -> [w1689 w1707 w1728 w1751]
              tunnel: w1682 -> [w1693 w1708 w1729 w1755]
              tunnel: w1685 -> [w1692 w1714 w1735 w1754]
              tunnel: w1684 -> [w1691 w1713 w1734 w1753]
              tunnel: [w1690 w1712 w1733 w1752] -> w1687
              tunnel: [w1688 w1711 w1732 w1749] -> w1681
              frame "Circular", Default {
                n801 = while {
                  shift-right: [w1700] -> _
                  shift-left: u8 1 -> [w1701]
                  tunnel: w1693 -> [w1706]
                  tunnel: w1692 -> [w1705]
                  tunnel: w1691 -> [w1704]
                  tunnel: [w1701] -> w1690
                  tunnel: w1689 -> [w1699]
                  shift-right: [w1697] -> _
                  shift-left: _ -> [w1696]
                  tunnel: [w1696] -> w1688
                  stop <- w1702 stop-if-true
                  n802 = Increment(x=w1701) -> (x+1=w1700:u8)
                  n803 = call "CalculateRadius.vi"("Scan Type"=w1699, "Points per Scan"=w1700, "Spacing (V)"=w1706) -> ("Maximum Voltage (V)"=w1695:dbl, "Radius (V)"=w1697:dbl)
                  n804 = Greater?(x=w1700, y=w1705) -> (0:w1698:bool)
                  n805 = Greater Or Equal?(x=w1695, y=w1704) -> (x >= y?=w1703:bool)
                  n806 = Or(x=w1698, y=w1703) -> (x .or. y?=w1702:bool)
                }
              }
              frame "Square" {
                w1709 = u8 4
                n807 = call "CalculateRadius.vi"("Scan Type"=w1707, "Points per Scan"=w1709, "Spacing (V)"=w1708) -> ("Radius (V)"=w1710:dbl)  [unwired: 1 out]
                n808 = while {
                  shift-right: [w1720] -> _
                  shift-left: w1709 -> [w1721]
                  tunnel: w1708 -> [w1727]
                  tunnel: w1714 -> [w1726]
                  tunnel: w1713 -> [w1725]
                  tunnel: [w1721] -> w1712
                  tunnel: w1707 -> [w1722]
                  shift-right: [w1717] -> _
                  shift-left: w1710 -> [w1716]
                  tunnel: [w1716] -> w1711
                  stop <- w1723 stop-if-true
                  n809 = Add(x=w1721, y=u8 4) -> (x+y=w1720:u8)
                  n810 = call "CalculateRadius.vi"("Scan Type"=w1722, "Points per Scan"=w1720, "Spacing (V)"=w1727) -> ("Maximum Voltage (V)"=w1715:dbl, "Radius (V)"=w1717:dbl)
                  n811 = Greater?(x=w1720, y=w1726) -> (0:w1718:bool)
                  n812 = Greater Or Equal?(x=w1715, y=w1725) -> (x >= y?=w1724:bool)
                  n813 = Or(x=w1718, y=w1724) -> (x .or. y?=w1723:bool)
                }
              }
              frame "FilledSquare" {
                w1730 = u8 2
                n814 = call "CalculateRadius.vi"("Scan Type"=w1728, "Points per Scan"=w1730, "Spacing (V)"=w1729) -> ("Radius (V)"=w1731:dbl)  [unwired: 1 out]
                n815 = while {
                  shift-right: [w1742] -> _
                  shift-left: w1730 -> [w1743]
                  tunnel: w1729 -> [w1748]
                  tunnel: w1735 -> [w1747]
                  tunnel: w1734 -> [w1746]
                  tunnel: [w1743] -> w1733
                  tunnel: w1728 -> [w1744]
                  shift-right: [w1739] -> _
                  shift-left: w1731 -> [w1738]
                  tunnel: [w1738] -> w1732
                  stop <- w1736 stop-if-true
                  n816 = Add(x=w1743, y=u8 1) -> (x+y=w1742:u8)
                  n817 = call "CalculateRadius.vi"("Scan Type"=w1744, "Points per Scan"=w1742, "Spacing (V)"=w1748) -> ("Maximum Voltage (V)"=w1737:dbl, "Radius (V)"=w1739:dbl)
                  n818 = Greater?(x=w1742, y=w1747) -> (0:w1740:bool)
                  n819 = Greater Or Equal?(x=w1737, y=w1746) -> (x >= y?=w1745:bool)
                  n820 = Or(x=w1740, y=w1745) -> (x .or. y?=w1736:bool)
                }
              }
              frame "Hexagonal" {
                n821 = while {
                  shift-right: [w1758] -> _
                  shift-left: u8 1 -> [w1773]
                  tunnel: w1755 -> [w1779]
                  tunnel: w1754 -> [w1778]
                  tunnel: w1753 -> [w1777]
                  tunnel: [w1773] -> w1752
                  tunnel: w1751 -> [w1774]
                  shift-right: [w1771] -> _
                  shift-left: _ -> [w1769]
                  tunnel: [w1769] -> w1749
                  i -> [w1772]
                  stop <- w1775 stop-if-true
                  n822 = To Unsigned Byte Integer(number=w1772) -> (unsigned 8bit integer=w1757:u8)
                  n823 = Multiply(x=w1757, y=w1757) -> (x*y=w1759:u8)
                  n824 = Multiply(x=w1757, y=u8 3) -> (x*y=w1760:u8)
                  n825 = Add(x=w1759, y=w1760) -> (x+y=w1761:u8)
                  n826 = Add(x=w1761, y=u8 2) -> (x+y=w1764:u8)
                  n827 = Quotient & Remainder(x=w1759, y=u8 4) -> (floor(x/y)=w1767:u8)  [unwired: 1 out]
                  n828 = Quotient & Remainder(x=w1764, y=u8 2) -> (floor(x/y)=w1768:u8)  [unwired: 1 out]
                  n829 = Add(x=w1767, y=w1768) -> (x+y=w1758:u8)
                  n830 = call "CalculateRadius.vi"("Scan Type"=w1774, "Points per Scan"=w1758, "Spacing (V)"=w1779) -> ("Maximum Voltage (V)"=w1756:dbl, "Radius (V)"=w1771:dbl)
                  n831 = Greater?(x=w1758, y=w1778) -> (0:w1770:bool)
                  n832 = Greater Or Equal?(x=w1756, y=w1777) -> (x >= y?=w1776:bool)
                  n833 = Or(x=w1770, y=w1776) -> (x .or. y?=w1775:bool)
                }
              }
            }
            n834 = Multiply(x=w1681, y=w1680) -> (x*y=w1679:dbl)
            n835 = local write "New Number of Points per Scan"(w1687) -> ()
            n836 = local write "New Radius (um)"(w1679) -> ()
          }
          event "New Spacing (um)": Value Change {
            # "Allow the spacing between points to change as long\nas it does not saturate the maximum voltage applied"
            n837 = event-data() -> ("NewVal"=w1792:dbl)  [unwired: 1 in]
            n838 = Divide(x=w1784, y=w1783) -> (x/y=w1782:dbl)
            n839 = Divide(x=w1792, y=w1783) -> (x/y=w1791:dbl)
            n840 = call "CalculateRadius.vi"("Scan Type"=w1795, "Points per Scan"=w1794, "Spacing (V)"=w1791) -> ("Maximum Voltage (V)"=w1793:dbl, "Radius (V)"=w1796:dbl)
            n841 = Subtract(x=w1781, y=w1782) -> (x-y=w1780:dbl)
            n842 = Less Or Equal?(x=w1780, y=w1793) -> (x <= y?=w1797:bool)
            n843 = case shown="True" w1797 {
              tunnel: w1780 -> [_ w1806]
              tunnel: w1793 -> [_ w1805]
              tunnel: w1796 -> [w1799 w1804]
              tunnel: w1791 -> [w1798 w1802]
              tunnel: [w1799 w1801] -> w1789
              tunnel: [w1798 w1800] -> w1790
              frame False {
                # "Not oversaturated"
              }
              frame True {
                # "Oversaturated"
                n844 = Divide(x=w1806, y=w1805) -> (x/y=w1803:dbl)
                n845 = Multiply(x=w1803, y=w1802) -> (x*y=w1800:dbl)
                n846 = Multiply(x=w1803, y=w1804) -> (x*y=w1801:dbl)
              }
            }
            n847 = Multiply(x=w1790, y=w1783) -> (x*y=w1787:dbl)
            n848 = Multiply(x=w1789, y=w1783) -> (x*y=w1788:dbl)
            n849 = local write "New Spacing (um)"(w1787) -> ()
            n850 = local write "New Radius (um)"(w1788) -> ()
          }
          event "New Radius (um)": Value Change {
            # "Allow the radius of the pattern to change as long\nas it does not saturate the maximum voltage applied"
            n851 = event-data() -> ()  [unwired: 1 in, 1 out]
            n852 = Divide(x=w1810, y=w1811) -> (x/y=w1809:dbl)
            n853 = Divide(x="New Radius (um)", y=w1811) -> (x/y=w1818:dbl)
            n854 = Subtract(x=w1808, y=w1809) -> (x-y=w1807:dbl)
            n855 = call "CalculateSpacing.vi"("Scan Type"=w1822, "Points per Scan"=w1821, "Radius (V)"=w1818) -> ("Maximum Voltage (V)"=w1820:dbl, "Spacing (V)"=w1823:dbl)
            n856 = Less Or Equal?(x=w1807, y=w1820) -> (x <= y?=w1824:bool)
            n857 = case shown="True" w1824 {
              tunnel: w1807 -> [_ w1833]
              tunnel: w1820 -> [_ w1832]
              tunnel: w1823 -> [w1826 w1831]
              tunnel: w1818 -> [w1825 w1829]
              tunnel: [w1826 w1828] -> w1816
              tunnel: [w1825 w1827] -> w1817
              frame False {
                # "Not oversaturated"
              }
              frame True {
                # "Oversaturated"
                n858 = Divide(x=w1833, y=w1832) -> (x/y=w1830:dbl)
                n859 = Multiply(x=w1830, y=w1829) -> (x*y=w1827:dbl)
                n860 = Multiply(x=w1830, y=w1831) -> (x*y=w1828:dbl)
              }
            }
            n861 = Multiply(x=w1817, y=w1811) -> (x*y=w1815:dbl)
            n862 = Multiply(x=w1816, y=w1811) -> (x*y=w1814:dbl)
            n863 = local write "New Spacing (um)"(w1814) -> ()
            n864 = local write "New Radius (um)"(w1815) -> ()
          }
          event "New EOD Deflection Scale (um/V)": Value Change {
            n865 = event-data() -> ("NewVal"=w1837:dbl)  [unwired: 1 in]
            n866 = call "CalculateRadius.vi"("Scan Type"=w1845, "Points per Scan"=w1846, "Spacing (V)"=w1840) -> ("Maximum Voltage (V)"=w1838:dbl)  [unwired: 1 out]
            n867 = Add(x=w1839, y=w1838) -> (x+y=w1836:dbl)
            n868 = Multiply(x=w1834, y=w1837) -> (x*y=w1835:dbl)
            n869 = Less Or Equal?(x=w1835, y=w1836) -> (x <= y?=w1844:bool)
            n870 = case shown="True" w1844 {
              tunnel: w1837 -> [w1847 _]
              tunnel: [w1847 w1850] -> w1843
              tunnel: w1836 -> [_ w1849]
              tunnel: w1834 -> [_ w1848]
              frame False {
              }
              frame True {
                # "Oversaturated"
                n871 = Divide(x=w1848, y=w1849) -> (x/y=w1850:dbl)
              }
            }
            n872 = local write "New EOD Deflection Scale (um/V)"(w1843) -> ()
          }
          event "New Modulation Radius (um)": Value Change {
            n873 = event-data() -> ("NewVal"=w1861:dbl)  [unwired: 1 in]
            n874 = Divide(x=w1861, y=w1854) -> (x/y=w1860:dbl)
            n875 = Divide(x=w1858, y=w1854) -> (x/y=w1859:dbl)
            n876 = call "CalculateRadius.vi"("Scan Type"=w1856, "Points per Scan"=w1857, "Spacing (V)"=w1859) -> ("Maximum Voltage (V)"=w1863:dbl)  [unwired: 1 out]
            n877 = Add(x=w1863, y=w1860) -> (x+y=w1865:dbl)
            n878 = Less?(x=w1865, y=w1862) -> (x < y?=w1866:bool)
            n879 = Subtract(x=w1862, y=w1863) -> (x-y=w1864:dbl)
            n880 = Select(t=w1860, s=w1866, f=w1864) -> (s? t:f=w1855:dbl)
            n881 = Multiply(x=w1855, y=w1854) -> (x*y=w1853:dbl)
            n882 = local write "New Modulation Radius (um)"(w1853) -> ()
          }
          event "Update FPGA": Value Change {
            n883 = event-data() -> ()  [unwired: 1 in, 1 out]
            n884 = flat-sequence {
              tunnel: [w1914] -> w1883
              tunnel: w1889 -> [w1914]
              tunnel: w1888 -> [w1921]
              tunnel: [w1920] -> w1882
              tunnel: w1887 -> [w1919]
              tunnel: w1886 -> [w1915]
              tunnel: [w1918] -> w1881
              tunnel: w1877 -> [w1904]
              tunnel: [w1904] -> w1876
              tunnel: [w1903] -> w1875
              tunnel: [w1903] -> w1874
              tunnel: w1873 -> [w1913]
              tunnel: [w1900] -> w1872
              tunnel: [w1899] -> w1871
              tunnel: [w1898] -> w1870
              tunnel: w1869 -> [w1897]
              tunnel: w1868 -> [w1892]
              tunnel: [w1969] -> w1880
              tunnel: w1891 -> [w2030]
              tunnel: w1890 -> [w2057]
              tunnel: w1883 -> [w1996]
              tunnel: w1882 -> [w2062]
              tunnel: [w2062] -> w1879
              tunnel: w1885 -> [w1947]
              tunnel: w1884 -> [w2021]
              tunnel: w1881 -> [w2026]
              tunnel: [w2026] -> w1878
              tunnel: w1876 -> [w2014]
              tunnel: w1875 -> [w1991]
              tunnel: w1872 -> [w2013]
              tunnel: w1871 -> [w2012]
              tunnel: w1867 -> [w1951]
              tunnel: w1880 -> [w2108]
              tunnel: w1879 -> [w2109]
              tunnel: w1878 -> [w2106]
              frame #0 {
                # "Bin Length (ticks)"
                n885 = Multiply(x=w1915, y=w1914) -> (x*y=w1917:dbl)
                n886 = Divide(x=w1904, y=w1917) -> (x/y=w1916:dbl)
                n887 = To Unsigned Word Integer(number=w1916) -> (unsigned 16bit integer=w1903:u16)
                n888 = Square(x="New Beam Waist Estimate (um)") -> (x^2=w1912:dbl)
                n889 = Multiply(x=u16 2, y=w1903) -> (x*y=w1905:u16)
                n890 = Multiply(x=w1904, y=w1912) -> (x*y=w1908:dbl)
                n891 = Multiply(x="New Diffusion Constant Estimate (um^2/s)", y=w1905) -> (x*y=w1911:dbl)
                n892 = Divide(x=w1908, y=w1911) -> (x/y=w1896:dbl)
                n893 = Scale By Power Of 2(n=w1892, x=w1896) -> (x*2^n=w1895:dbl)
                n894 = To Unsigned Long Integer(number=w1895) -> (unsigned 32bit integer=w1909:u32)
                n895 = Split Number(x=w1909) -> (hi(x)=w1910:u16, lo(x)=w1899:u16)
                n896 = local read "Trap"() -> (w1918:bool)
                n897 = Split Number(x=w1910) -> (lo(x)=w1900:u8)  [unwired: 1 out]
                n898 = Join Numbers(hi=w1900, lo=w1899) -> ((hi.lo)=w1898:u32)
                n899 = Multiply(x=w1898, y=w1905) -> (x*y=w1906:u32)
                n900 = case shown="True" w1918 {
                  tunnel: w1921 -> [w1922 w1935]
                  tunnel: [w1922 w1934] -> w1920
                  tunnel: w1914 -> [_ w1929]
                  tunnel: w1919 -> [_ w1933]
                  tunnel: w1903 -> [_ w1932]
                  tunnel: w1898 -> [_ w1928]
                  tunnel: w1897 -> [_ w1927]
                  tunnel: w1913 -> [_ w1924]
                  frame False {
                  }
                  frame True {
                    n901 = Not Equal?(x=w1928, y=w1927) -> (x != y?=w1923:bool)
                    n902 = Not Equal?(x=w1933, y=w1929) -> (x != y?=w1930:bool)
                    n903 = Not Equal?(x=w1924, y=w1932) -> (x != y?=w1931:bool)
                    n904 = Or(x=w1930, y=w1931) -> (x .or. y?=w1926:bool)
                    n905 = Or(x=w1923, y=w1926) -> (x .or. y?=w1925:bool)
                    n906 = case shown="True" w1925 {
                      tunnel: w1935 -> [w1936 w1944]
                      tunnel: [w1936 w1937] -> w1934
                      frame False {
                      }
                      frame True {
                        # "Critical parameter change - must stop during update"
                        n907 = Join Numbers(hi=u8 1, lo=u8 0) -> ((hi.lo)=w1941:u16)
                        n908 = Join Numbers(hi=w1941, lo=u16 0) -> ((hi.lo)=w1939:u32)
                        n909 = Build Array(w1939) -> (w1938:u32[])
                        n910 = xnode "Invoke Method"("FPGA VI Reference In"=w1944, "Data"=w1938) -> ("FPGA VI Reference Out"=w1937:refnum<k20>)  [unwired: 2 in, 2 out]
                      }
                    }
                  }
                }
                n911 = Divide(x=w1908, y=w1906) -> (x/y=w1894:dbl)
                n912 = Scale By Power Of 2(n=w1892, x=w1894) -> (x*2^n=→"Current Diffusion Constant Estimate (um^2/s)":dbl)
                "Current Beam Waist Estimate (um)" <- "New Beam Waist Estimate (um)"
              }
              frame #1 {
                w1966 = 3276.8 ("y")
                w1994 = 3276.8 ("y")
                w2059 = 3276.8 ("y")
                # "Modulation points"
                # "EOD positions"
                # "Determine the Voltages required for the requested pattern/number of points"
                n913 = To Double Precision Float(number=w1991) -> (double precision float=w1990:dbl)
                n914 = Multiply(x=w1990, y=w1996) -> (x*y=w2063:dbl)
                n915 = Multiply(x=w2014, y=w1947) -> (x*y=w2024:dbl)
                n916 = Divide(x=w2014, y=w2063) -> (x/y=w1985:dbl)
                "Current Scan Frequency (Hz)" <- w1985
                n917 = Initialize Array "Commands to Send"(u32 0 ("element"), 0 ("dimension size")) -> (w2066:u32[])
                n918 = To Unsigned Word Integer(number=w1996) -> (unsigned 16bit integer=w2022:u16)
                n919 = Join Numbers(hi=u8 8, lo=u8 0) -> ((hi.lo)=w2051:u16)
                n920 = Join Numbers(hi=w2051, lo=w1991) -> ((hi.lo)=w2048:u32)
                n921 = Multiply(x="New Number of Modulation Points", y="New Modulation Frequency (Hz)") -> (x*y=w1988:dbl)
                n922 = Insert Into Array "Bin Length"(array=w2066, new element=w2048) -> (w2065:u32[])  [unwired: 1 in]
                n923 = Divide(x=w1985, y=w1988) -> (x/y=w1987:dbl)
                n924 = To Unsigned Long Integer(number=w1987) -> (unsigned 32bit integer=w1978:u32)
                n925 = Join Numbers(hi=u8 9, lo=u8 0) -> ((hi.lo)=w2047:u16)
                n926 = Split Number(x=w1978) -> (hi(x)=w1982:u16, lo(x)=w1954:u16)
                n927 = Join Numbers(hi=w2047, lo=w2022) -> ((hi.lo)=w2044:u32)
                n928 = Split Number(x=w1982) -> (lo(x)=w1955:u8)  [unwired: 1 out]
                n929 = Join Numbers(hi=u8 0, lo=w1955) -> ((hi.lo)=w1956:u16)
                n930 = Insert Into Array "Bins/cycle"(array=w2065, new element=w2044) -> (w2064:u32[])  [unwired: 1 in]
                n931 = Join Numbers(hi=w1956, lo=w1954) -> ((hi.lo)=w1952:u32)
                n932 = Multiply(x="New Number of Modulation Points", y=w1952) -> (x*y=w1986:u32)
                n933 = Join Numbers(hi=u8 11, lo=u8 0) -> ((hi.lo)=w2041:u16)
                n934 = Divide(x=w1985, y=w1986) -> (x/y=→"Current Modulation Frequency (Hz)":dbl)
                n935 = Join Numbers(hi=w2041, lo="New Sub-Bin Delay") -> ((hi.lo)=w2040:u32)
                n936 = Multiply(x="New Mobility Estimate (um/s/V)", y=w1990) -> (x*y=w2033:dbl)
                n937 = Divide(x=w2024, y=w2033) -> (x/y=w2032:dbl)
                n938 = Insert Into Array "Sub-Bin Delay"(array=w2064, new element=w2040) -> (w2053:u32[])  [unwired: 1 in]
                n939 = To Word Integer(number=w2032) -> (16bit integer=w2004:i16)
                n940 = Join Numbers(hi=u8 5, lo=w2013) -> ((hi.lo)=w2038:u16)
                n941 = Join Numbers(hi=w2038, lo=w2012) -> ((hi.lo)=w2037:u32)
                n942 = In Range and Coerce(upper limit=i16 32767, x=w2004, lower limit=i16 -32767) -> (coerced(x)=w2000:i16)  [unwired: 1 out]
                n943 = Insert Into Array "Inverse Diffusion Constant"(array=w2053, new element=w2037) -> (w2052:u32[])  [unwired: 1 in]
                n944 = Multiply(x=w2000, y=w1990) -> (x*y=w2023:dbl)
                n945 = Absolute Value(x=w2000) -> (abs(x)=w1997:i16)
                n946 = Join Numbers(hi=u8 6, lo=u8 0) -> ((hi.lo)=w2035:u16)
                n947 = Multiply(x=w1994, y="New Maximum Feedback (V)") -> (x*y=w1993:dbl)
                n948 = Divide(x=w2024, y=w2023) -> (x/y=→"Current Mobility Estimate (um/s/V)":dbl)
                n949 = Join Numbers(hi=w2035, lo=w2000) -> ((hi.lo)=w2034:u32)
                n950 = To Word Integer(number=w1993) -> (16bit integer=w1992:i16)
                n951 = Insert Into Array "Inverse Mobility"(array=w2052, new element=w2034) -> (w2017:u32[])  [unwired: 1 in]
                n952 = Quotient & Remainder(x=w1992, y=w1997) -> (floor(x/y)=w2001:i16)  [unwired: 1 out]
                n953 = call "CreateScanPattern.vi"("Point Spacing"=w2030, "Number of Points"=w1996, "Pattern"=w2057) -> ("Radius"=→"Current Radius (um)":dbl, "Y coordinates"=w2055:dbl[], "X coordinates"=w2054:dbl[])
                n954 = Multiply(x=w2001, y=w1997) -> (x*y=w1999:i16)
                n955 = Join Numbers(hi=u8 7, lo=u8 0) -> ((hi.lo)=w2019:u16)
                n956 = Join Numbers(hi=w2019, lo=w2001) -> ((hi.lo)=w2020:u32)
                n957 = Insert Into Array "Saturated Position Step"(array=w2017, new element=w2020) -> (w2007:u32[])  [unwired: 1 in]
                n958 = Bundle("X coordinates"=w2054, "Y coordinates"=w2055) -> (w1958:T33)  [unwired: 1 in]
                n959 = Build Array(w2054, w2055) -> (w2029:dbl[][])
                n960 = Divide(x=w2029, y=w1947) -> (x/y=w2028:dbl[][])
                n961 = Divide(x=w1999, y=w1994) -> (x/y=→"Current Maximum Feedback (V)":dbl)
                n962 = Multiply(x=w2028, y=w2059) -> (x*y=w2060:dbl[][])
                n963 = Join Numbers(hi=u8 4, lo=u8 0) -> ((hi.lo)=w2008:u16)
                n964 = Boolean To (0,1)(Boolean="Include Mobility Update") -> (0, 1=w2011:i16)
                n965 = To Word Integer(number=w2060) -> (16bit integer=w2027:i16[][])
                n966 = Join Numbers(hi=w2008, lo=w2011) -> ((hi.lo)=w2006:u32)
                n967 = Divide(x=w2027, y=w2059) -> (x/y=w2058:dbl[][])
                n968 = local write "Current Voltages"(w2058) -> ()
                n969 = Insert Into Array "Include Mobility Update"(array=w2007, new element=w2006) -> (w1983:u32[])  [unwired: 1 in]
                n970 = call "InterpolateCircle.vi"("Radius"=w1951, "Start Angle (degrees)"="New Modulation Angle (degrees)", "Number of Points"="New Number of Modulation Points") -> ("Y coordinates"=w1960:dbl[], "X coordinates"=w1961:dbl[])
                n971 = Join Numbers(hi=u8 12, lo=w1955) -> ((hi.lo)=w1980:u16)
                n972 = Join Numbers(hi=w1980, lo=w1954) -> ((hi.lo)=w1979:u32)
                n973 = Bundle("X coordinates"=w1961, "Y coordinates"=w1960) -> (w1959:T33)  [unwired: 1 in]
                n974 = Build Array(w1961, w1960) -> (w1950:dbl[][])
                n975 = Insert Into Array "Cycles per Modulation Point"(array=w1983, new element=w1979) -> (w1973:u32[])  [unwired: 1 in]
                n976 = Divide(x=w1950, y=w1947) -> (x/y=w1949:dbl[][])
                n977 = Build Array(w1958, w1959) -> (w1957:T10)
                n978 = case shown="False" w2026 {
                  tunnel: w1957 -> [w2087 _]
                  frame False {
                    n979 = local write "Position Plot"(w2087) -> ()
                  }
                  frame True {
                  }
                }
                n980 = Multiply(x=w1949, y=w1966) -> (x*y=w1968:dbl[][])
                n981 = Join Numbers(hi=u8 13, lo=u8 0) -> ((hi.lo)=w1976:u16)
                n982 = Join Numbers(hi=w1976, lo="New Number of Modulation Points") -> ((hi.lo)=w1975:u32)
                n983 = To Word Integer(number=w1968) -> (16bit integer=w1967:i16[][])
                n984 = Insert Into Array "Number of Modulation Points"(array=w1973, new element=w1975) -> (w1971:u32[])  [unwired: 1 in]
                n985 = Divide(x=w1967, y=w1966) -> (x/y=w1945:dbl[][])
                "Current Modulation Voltages" <- w1945
                n986 = for {
                  N: w1996 -> [_]
                  shift-right: [w2092] -> w1970
                  shift-left: w1971 -> [w2093]
                  tunnel: w2027 -> [w2091]
                  i -> [w2089]
                  n987 = Index Array(array=w2091, index (col)=w2089) -> (element=w2090:i16[])  [unwired: 1 in]
                  n988 = for {
                    N: 2 -> [_]
                    tunnel: w2090 -> [w2094] mode=indexing
                    tunnel: w2089 -> [w2103]
                    shift-right: [w2097] -> w2092
                    shift-left: w2093 -> [w2098]
                    i -> [w2105]
                    n989 = To Unsigned Byte Integer(number=w2103) -> (unsigned 8bit integer=w2102:u8)
                    n990 = To Unsigned Byte Integer(number=w2105) -> (unsigned 8bit integer=w2095:u8)
                    n991 = Add(x=w2095, y=u8 16 ("x")) -> (x+y=w2104:u8)
                    n992 = Join Numbers(hi=w2104, lo=w2102) -> ((hi.lo)=w2101:u16)
                    n993 = To Unsigned Word Integer(number=w2094) -> (unsigned 16bit integer=w2100:u16)
                    n994 = Join Numbers(hi=w2101, lo=w2100) -> ((hi.lo)=w2099:u32)
                    n995 = Insert Into Array(array=w2098, new element=w2099) -> (w2097:u32[])  [unwired: 1 in]
                  }
                }
                n996 = Square(x=w1945) -> (x^2=w1965:dbl[][])
                n997 = Add Array Elements(numeric array=w1965) -> (sum=w1964:dbl)
                n998 = Divide(x=w1964, y="New Number of Modulation Points") -> (x/y=w1962:dbl)
                n999 = Send Notification(notification=w1957, notifier=w2021) -> ()  [unwired: 1 in, 2 out]
                n1000 = Square Root(x=w1962) -> (sqrt(x)=w1948:dbl)
                n1001 = Multiply(x=w1948, y=w1947) -> (x*y=→"Current Modulation Radius (um)":dbl)
                n1002 = for {
                  N: "New Number of Modulation Points" -> [_]
                  shift-right: [w2073] -> w1969
                  shift-left: w1970 -> [w2074]
                  tunnel: w1967 -> [w2072]
                  i -> [w2070]
                  n1003 = Index Array(array=w2072, index (col)=w2070) -> (element=w2071:i16[])  [unwired: 1 in]
                  n1004 = for {
                    N: 2 -> [_]
                    tunnel: w2071 -> [w2075] mode=indexing
                    tunnel: w2070 -> [w2084]
                    shift-right: [w2078] -> w2073
                    shift-left: w2074 -> [w2079]
                    i -> [w2086]
                    n1005 = To Unsigned Byte Integer(number=w2084) -> (unsigned 8bit integer=w2083:u8)
                    n1006 = To Unsigned Byte Integer(number=w2086) -> (unsigned 8bit integer=w2076:u8)
                    n1007 = Add(x=w2076, y=u8 20 ("x")) -> (x+y=w2085:u8)
                    n1008 = Join Numbers(hi=w2085, lo=w2083) -> ((hi.lo)=w2082:u16)
                    n1009 = To Unsigned Word Integer(number=w2075) -> (unsigned 16bit integer=w2081:u16)
                    n1010 = Join Numbers(hi=w2082, lo=w2081) -> ((hi.lo)=w2080:u32)
                    n1011 = Insert Into Array(array=w2079, new element=w2080) -> (w2078:u32[])  [unwired: 1 in]
                  }
                }
                "Current Scan Form" <- w2057
                "Current Spacing (um)" <- w2030
                "Current EOD Deflection Scale (um/V)" <- w1947
                "Current Sub-Bin Delay" <- "New Sub-Bin Delay"
                "Current Number of Points per Scan" <- w1996
                "Current Number of Modulation Points" <- "New Number of Modulation Points"
                "Current Modulation Angle (degrees)" <- "New Modulation Angle (degrees)"
              }
              frame #2 {
                n1012 = case shown="True" w2106 {
                  tunnel: w2108 -> [w2112 w2115]
                  tunnel: [w2112 w2114] -> w2107
                  frame False {
                  }
                  frame True {
                    # "Restart things (if going)"
                    n1013 = Join Numbers(hi=u8 1, lo=u8 0) -> ((hi.lo)=w2117:u16)
                    n1014 = Join Numbers(hi=w2117, lo=u16 1) -> ((hi.lo)=w2113:u32)
                    n1015 = Insert Into Array(array=w2115, new element=w2113) -> (w2114:u32[])  [unwired: 1 in]
                  }
                }
                n1016 = xnode "Invoke Method"("FPGA VI Reference In"=w2109, "Data"=w2107, "Timeout (ms)"=-1) -> ()  [unwired: 1 in, 3 out]
                n1017 = local write "Ready"(TRUE ("Ready")) -> ()
              }
            }
          }
          event "Record": Value Change {
            n1018 = event-data() -> ("NewVal"=w2130:bool)  [unwired: 1 in]
            n1019 = case shown="False" w2130 {
              tunnel: w2129 -> [_ w2145]
              tunnel: w2128 -> [_ w2144]
              tunnel: w2127 -> [w2134 w2146]
              tunnel: w2124 -> [_ w2142]
              tunnel: w2123 -> [_ w2141]
              tunnel: w2122 -> [_ w2140]
              tunnel: w2121 -> [_ w2139]
              tunnel: w2120 -> [_ w2138]
              frame False {
                # "Close any file created previously if it hasn't been used"
                n1020 = Wait on Notification(notifier=w2134, timeout in ms (-1)=0) -> (notification=w2131:T30, timed out?=w2132:bool)  [unwired: 2 in, 2 out]
                n1021 = case shown="False" w2132 {
                  tunnel: w2131 -> [w2137 _]
                  frame False {
                    n1022 = Unbundle(w2137) -> ("Photon File"=w2136:refnum<file>, "Feedback File"=w2135:refnum<file>)
                    n1023 = Close File(refnum=w2135) -> ()  [unwired: 1 in, 2 out]
                    n1024 = Close File(refnum=w2136) -> ()  [unwired: 1 in, 2 out]
                  }
                  frame True {
                  }
                }
              }
              frame True {
                n1025 = local read "Trap"() -> (w2143:bool)
                n1026 = case shown="True" w2143 {
                  tunnel: w2146 -> [_ w2159]
                  tunnel: w2145 -> [_ w2158]
                  tunnel: w2144 -> [_ w2157]
                  tunnel: w2142 -> [w2147 _]
                  tunnel: w2141 -> [_ w2154]
                  tunnel: w2140 -> [_ w2153]
                  tunnel: w2139 -> [_ w2152]
                  tunnel: w2138 -> [_ w2149]
                  frame False {
                    # "Not in any data-acquisition mode - cannot record"
                    n1027 = local write "Record"(FALSE ("Record")) -> ()
                    n1028 = One Button Dialog(message=w2147) -> ()  [unwired: 1 in, 1 out]
                  }
                  frame True {
                    n1029 = local read "Workspace"() -> (w2151:path)
                    n1030 = Strip Path(path=w2151) -> (stripped path=w2150:path)  [unwired: 1 out]
                    n1031 = Build Path(base path=w2150, name or relative path=w2149) -> (appended path=w2155:path)
                    n1032 = call <vilib>:"Check if File or Folder Exists.vi"("path"=w2155) -> ("file or folder exists?"=w2156:bool)  [unwired: 8 in, 2 out]
                    n1033 = case shown="False" w2156 {
                      tunnel: w2159 -> [w2215 _]
                      tunnel: w2158 -> [w2204 _]
                      tunnel: w2157 -> [w2202 _]
                      tunnel: w2149 -> [w2167 _]
                      tunnel: w2155 -> [w2160 _]
                      tunnel: w2154 -> [_ w2239]
                      tunnel: w2153 -> [w2186 _]
                      tunnel: w2152 -> [w2166 _]
                      frame False {
                        # "Modulation Text Header File"
                        # "Modulation Binary Header File (Voltages lookup tables)"
                        # "Binary Header File (Voltages lookup tables)"
                        # "Binary Data Files"
                        # "Text Header File"
                        # "Open files and output header information"
                        n1034 = local read "Current Sub-Bin Delay"() -> (w2198:u16)
                        n1035 = local read "Current Diffusion Constant Estimate (um^2/s)"() -> (w2201:dbl)
                        n1036 = Multiply(x=w2204, y=w2202) -> (x*y=w2228:dbl)
                        n1037 = local read "Current Number of Modulation Points"() -> (w2164:u8)
                        n1038 = local read "Current EOD Deflection Scale (um/V)"() -> (w2205:dbl)
                        n1039 = local read "Current Modulation Frequency (Hz)"() -> (w2165:dbl)
                        n1040 = Divide(x=1000000000.0, y=w2228) -> (x/y=w2209:dbl)
                        n1041 = local read "Current Mobility Estimate (um/s/V)"() -> (w2200:dbl)
                        n1042 = local read "Current Beam Waist Estimate (um)"() -> (w2206:dbl)
                        n1043 = local read "Current Modulation Radius (um)"() -> (w2162:dbl)
                        n1044 = local read "Current Maximum Feedback (V)"() -> (w2187:dbl)
                        n1045 = local read "Current Modulation Angle (degrees)"() -> (w2163:dbl)
                        n1046 = Divide(x=w2198, y=0.08 ("x")) -> (x/y=w2207:dbl)
                        n1047 = local read "Include Mobility Update"() -> (w2188:bool)
                        n1048 = local read "Current Spacing (um)"() -> (w2208:dbl)
                        n1049 = local read "Current Scan Form"() -> (w2197:enum8{"Circular", "Square", "Hexagonal"})
                        n1050 = Get Date/Time In Seconds() -> (seconds since 1Jan1904=w2230:timestamp)
                        n1051 = Format Date/Time String(time format string (%c)="%Y-%m-%d\n%H:%M:%S\n", seconds (now)=w2230) -> (date/time string=w2210:string)  [unwired: 1 in]
                        n1052 = Format Into String(format string=w2186, initial string=w2210, w2204, w2209, w2197, w2202, w2208, w2207, w2206, w2205, w2201, w2200, w2187, w2188) -> (resulting string=w2199:string)  [unwired: 1 in, 1 out]
                        n1053 = Format Into String(format string=w2166, w2165, w2164, w2162, w2163) -> (resulting string=w2161:string)  [unwired: 2 in, 1 out]
                        n1054 = local read "Current Modulation Voltages"() -> (w2176:dbl[][])
                        n1055 = local read "Current Voltages"() -> (w2211:dbl[][])
                        n1056 = Create Folder(path (use dialog)=w2160) -> (created path=w2168:path)  [unwired: 2 in, 2 out]
                        n1057 = Concatenate Strings(w2167, "_modheader.txt" ("string")) -> (w2170:string)
                        n1058 = Concatenate Strings(w2167, "_header.dat" ("string")) -> (w2236:string)
                        n1059 = Concatenate Strings(w2167, "_header.txt" ("string")) -> (w2224:string)
                        n1060 = Concatenate Strings(w2167, "_modheader.dat" ("string")) -> (w2177:string)
                        n1061 = Concatenate Strings(w2167, "_photons.dat" ("string")) -> (w2231:string)
                        n1062 = Concatenate Strings(w2167, "_feedbacks.dat" ("string")) -> (w2193:string)
                        n1063 = Build Path(base path=w2168, name or relative path=w2177) -> (appended path=w2184:path)
                        n1064 = Build Path(base path=w2168, name or relative path=w2170) -> (appended path=w2173:path)
                        n1065 = Build Path(base path=w2168, name or relative path=w2236) -> (appended path=w2235:path)
                        n1066 = Build Path(base path=w2168, name or relative path=w2224) -> (appended path=w2221:path)
                        n1067 = Build Path(base path=w2168, name or relative path=w2231) -> (appended path=w2216:path)
                        n1068 = Build Path(base path=w2168, name or relative path=w2193) -> (appended path=w2196:path)
                        n1069 = Open/Create/Replace File(file path (use dialog)=w2184, operation (0:open)=T32."create", access (0:read/write)=enum16{"read/write", "read-only", "write-only"}."write-only") -> (refnum out=w2181:refnum<file>)  [unwired: 3 in, 2 out]
                        n1070 = Open/Create/Replace File(file path (use dialog)=w2173, operation (0:open)=T32."create", access (0:read/write)=enum16{"read/write", "read-only", "write-only"}."write-only") -> (refnum out=w2175:refnum<file>)  [unwired: 3 in, 2 out]
                        n1071 = Open/Create/Replace File(file path (use dialog)=w2221, operation (0:open)=T32."create", access (0:read/write)=enum16{"read/write", "read-only", "write-only"}."write-only") -> (refnum out=w2219:refnum<file>)  [unwired: 3 in, 2 out]
                        n1072 = Open/Create/Replace File(file path (use dialog)=w2216, operation (0:open)=T32."create", access (0:read/write)=enum16{"read/write", "read-only", "write-only"}."write-only") -> (refnum out=w2191:refnum<file>)  [unwired: 3 in, 2 out]
                        n1073 = Open/Create/Replace File(file path (use dialog)=w2196, operation (0:open)=T32."create", access (0:read/write)=enum16{"read/write", "read-only", "write-only"}."write-only") -> (refnum out=w2190:refnum<file>)  [unwired: 3 in, 2 out]
                        n1074 = Open/Create/Replace File(file path (use dialog)=w2235, operation (0:open)=T32."create", access (0:read/write)=enum16{"read/write", "read-only", "write-only"}."write-only") -> (refnum out=w2213:refnum<file>)  [unwired: 3 in, 2 out]
                        n1075 = Bundle("refnum out"=w2191, "refnum out"=w2190) -> (w2189:T34)  [unwired: 1 in]
                        n1076 = Send Notification(notification=w2189, notifier=w2215) -> ()  [unwired: 1 in, 2 out]
                        n1077 = Write to Text File(file (use dialog)=w2175, text=w2161) -> (refnum out=w2174:refnum<file>)  [unwired: 2 in, 2 out]
                        n1078 = Write to Text File(file (use dialog)=w2219, text=w2199) -> (refnum out=w2220:refnum<file>)  [unwired: 2 in, 2 out]
                        n1079 = Write to Binary File(file (use dialog)=w2181, data=w2176, 5:FALSE ("prepend array or string size? (T)"), 9:T31."native, host order" ("byte order (0:big-endian, network order)")) -> (refnum out=w2179:refnum<file>)  [unwired: 2 in, 2 out]
                        n1080 = Write to Binary File(file (use dialog)=w2213, data=w2211, 5:FALSE ("prepend array or string size? (T)"), 9:T31."native, host order" ("byte order (0:big-endian, network order)")) -> (refnum out=w2203:refnum<file>)  [unwired: 2 in, 2 out]
                        n1081 = Close File(refnum=w2174) -> ()  [unwired: 1 in, 2 out]
                        n1082 = Close File(refnum=w2220) -> ()  [unwired: 1 in, 2 out]
                        n1083 = Close File(refnum=w2179) -> ()  [unwired: 1 in, 2 out]
                        n1084 = Close File(refnum=w2203) -> ()  [unwired: 1 in, 2 out]
                      }
                      frame True {
                        n1085 = local write "Record"(FALSE ("Record")) -> ()
                        n1086 = One Button Dialog(message=w2239) -> ()  [unwired: 1 in, 1 out]
                      }
                    }
                  }
                }
              }
            }
          }
          event "Stop Program": Value Change {
            # "Stop trapping"
            n1087 = event-data() -> ("NewVal"=w2250:bool)  [unwired: 1 in]
            n1088 = Join Numbers(hi=u8 1, lo=u8 0) -> ((hi.lo)=w2245:u16)
            n1089 = Join Numbers(hi=w2245, lo=u16 0) -> ((hi.lo)=w2248:u32)
            n1090 = Build Array(w2248) -> (w2249:u32[])
            n1091 = xnode "Invoke Method"("FPGA VI Reference In"=w2243, "Data"=w2249, "Timeout (ms)"=-1) -> ()  [unwired: 1 in, 3 out]
          }
        }
        n1092 = feedback-in #14(w1333) -> ()
        n1093 = feedback-in #15(w1331) -> ()
      }
    }
    frame #2 {
      # "Stop resources shared between the loops"
      n1094 = xnode "Invoke Method"("FPGA VI Reference In"=w2284) -> ("FPGA VI Reference Out"=w2283:refnum<k20>)  [unwired: 1 in, 1 out]
      n1095 = Release Notifier(notifier=w2281) -> ()  [unwired: 2 in, 3 out]
      n1096 = Release Notifier(notifier=w2280) -> ()  [unwired: 2 in, 3 out]
      n1097 = local write "Trap"(FALSE ("Trap")) -> ()
      n1098 = xnode "Close FPGA VI Reference"("FPGA VI Reference In"=w2283) -> ()  [unwired: 1 in, 1 out]
    }
  }
  n1099 = while {
    tunnel: [w2301] -> w7
    tunnel: w2 -> [w2300]
    stop <- w2304 stop-if-true
    n1100 = local read "Global Stop"() -> (w2302:bool)
    n1101 = call "Vision Acquisition"("Auto Exposure::Mode"="Auto Exposure::Mode", "Auto Exposure::Value"="Auto Exposure::Value", "Brightness::Mode"="Brightness::Mode", "Brightness::Value"="Brightness::Value", "Gain::Mode"="Gain::Mode", "Stop (F)"=w2302, "Gain::Value"="Gain::Value", "error in"=w2300, "Gamma::Mode"="Gamma::Mode", "Shutter::Mode"="Shutter::Mode", "Shutter::Value"="Shutter::Value", "Trigger::Trigger Activation"="Trigger::Trigger Activation", "Trigger::Trigger Mode"="Trigger::Trigger Mode", "Trigger::Trigger Parameter"="Trigger::Trigger Parameter", "Trigger Delay::Mode"="Trigger Delay::Mode") -> ("Image Out"=→"Image Out":T9, "Image Number"=→"Image Number":u32, "Frame Rate"=→"acquired FPS":dbl, "Stopped"=w2304:bool, "error out"=w2301:errorcluster)  [unwired: 8 in]
  }
  n1102 = while {
    tunnel: w38 -> [w2308]
    shift-right: [w2307] -> w36
    shift-left: w2 -> [w2309]
    stop <- w2306 stop-if-true
    n1103 = Wait (ms)(milliseconds to wait=u32 50) -> ()  [unwired: 1 out]
    n1104 = case shown="False" "SCANNER EMERGENCY" {
      tunnel: w2308 -> [_ w2315]
      tunnel: w2309 -> [w2312 w2316]
      tunnel: [w2312 w2317] -> w2307
      frame False {
        n1105 = Wait Until Next ms Multiple(millisecond multiple=u32 100) -> ()  [unwired: 1 out]
      }
      frame True {
        n1106 = call "PI Write GPIB.vi"("System no."=w2315, "String to send"="0RT", "error in"=w2316) -> ("error out"=w2314:errorcluster)  [unwired: 16 in]
        n1107 = flat-sequence {
          tunnel: [w2318] -> w2317
          tunnel: w2314 -> [w2318]
          frame #0 {
            n1108 = One Button Dialog(message="Emergency scanner stop appeared!!!\nCheck scanner settings before continue!!!") -> ()  [unwired: 2 out]
          }
        }
      }
    }
    n1109 = local read "Global Stop"() -> (w2306:bool)
  }
  n1110 = Merge Errors(w7, w36) -> (w29:errorcluster)
  n1111 = while {
    shift-right: [w2327] -> w44
    shift-left: w2 -> [w2324]
    tunnel: w37 -> [w2335]
    tunnel: [w2334] -> w47
    shift-right: [w2329] -> w31
    shift-left: w2 -> [w2336]
    tunnel: w45 -> [w2328]
    tunnel: "Image Measurent Parameters" -> [w2322]
    tunnel: [w2321] -> w41
    tunnel: "Sample description" -> [w2320]
    stop <- w2332 stop-if-true
    n1112 = case shown="No Error" w2324 {
      selector: w2324 -> [w2351 w2911]
      tunnel: w2336 -> [w2363 w2914]
      tunnel: w2335 -> [w2362 w2915]
      tunnel: [w2361 w2915] -> w2334
      tunnel: [w2360 TRUE ("Global Stop")] -> w2331
      tunnel: [w2356 w2914] -> w2330
      tunnel: w2328 -> [w2355 _]
      tunnel: [w2354 w2911] -> w2327
      tunnel: [w2352 T14."No Measurement" ("Do Measurement")] -> w2325
      tunnel: [w2349 FALSE] -> w2323
      tunnel: w2322 -> [w2348 _]
      tunnel: [w2339 w2911] -> w2321
      tunnel: w2320 -> [w2337 _]
      frame No Error {
        n1113 = while {
          shift-right: [w2909] -> w2357
          shift-left: w2363 -> [w2909]
          tunnel: [w2904] -> w2359
          tunnel: [w2906] -> w2358
          tunnel: [w2905] -> w2353
          stop <- w2910 stop-if-true
          w2905 = FALSE ("FiFo Overrun")
          # "Wait for Start"
          n1114 = local read "Global Stop"() -> (w2906:bool)
          n1115 = Wait (ms)(milliseconds to wait=u32 100) -> ()  [unwired: 1 out]
          n1116 = local write "Stop Measurement"(w2905) -> ()
          n1117 = local read "Task"() -> (w2904:T1)
          n1118 = Greater Than 0?(x=w2904) -> (x > 0?=w2908:bool)
          n1119 = Or(x=w2908, y=w2906) -> (x .or. y?=w2910:bool)
        }
        n1120 = Build Array("X-Axis Offset", "Y-Axis Offset", "Z-Axis Offset") -> (w2340:dbl[])
        n1121 = control-ref of="WS File Tree"() -> (w2350:refnum<vi>)
        n1122 = local write "Buffer Overrun"(w2353) -> ()
        n1123 = Build Array("X-Axis Points", "Y-Axis Points", "Z-Axis Points") -> (w2344:u16[])
        n1124 = case shown="\"Aquire Image\"" w2359 {
          selector: w2359 -> [_ _ w2697 _]
          tunnel: w2351 -> [w2364 w2404 w2667 w2854]
          tunnel: w2362 -> [w2369 w2401 w2630 w2851]
          tunnel: [w2369 w2373 w2630 w2851] -> w2361
          tunnel: [w2364 w2374 w2634 w2841] -> w2354
          tunnel: [w2365 FALSE ("Global Stop") FALSE ("Global Stop") FALSE ("Global Stop")] -> w2360
          tunnel: w2358 -> [w2365 _ _ _]
          tunnel: w2357 -> [w2368 w2387 w2716 w2853]
          tunnel: [w2368 w2387 w2722 w2853] -> w2356
          tunnel: w2355 -> [_ w2459 w2638 _]
          tunnel: [T14."No Measurement" ("Do Measurement") T14."No Measurement" ("Do Measurement") w2696 T14."No Measurement" ("Do Measurement")] -> w2352
          tunnel: w2350 -> [_ _ w2684 _]
          tunnel: [FALSE FALSE w2673 FALSE] -> w2349
          tunnel: w2348 -> [_ w2436 _ _]
          tunnel: w2344 -> [_ _ _ _]
          tunnel: w2340 -> [_ _ _ _]
          tunnel: [w2364 w2407 w2668 w2841] -> w2339
          tunnel: "Laser pulse duration" -> [_ _ w2646 _]
          tunnel: w2337 -> [_ _ w2629 _]
          frame "No Measurement", Default {
          }
          frame "Aquire Image" {
            w2397 = T39."Image File" ("Measurement Type")
            w2440 = 32768 ("dimension size")
            # "TODO:\n- FIFO Read Flag Buffer Half Full?\n- auto square pixels"
            # "Image Intensity Array"
            n1125 = Index Array(array=w2459) -> (element=w2458:T40)  [unwired: 1 in]
            n1126 = Unbundle By Name(w2458) -> ("Dev"=w2427:i32)
            n1127 = Index Array(array=string[] ["yx", "yz", "xy", "xz", "zy", "zx"] ("Array"), index="Axis") -> (element=w2379:string)
            n1128 = stacked-sequence {
              seq-local: [w2471 _] -> [_ w2498]
              seq-local: [w2470 _] -> [_ w2499]
              seq-local: [w2469 _] -> [_ w2494]
              seq-local: [w2465 _] -> [_ w2492]
              seq-local: [w2466 _] -> [_ w2491]
              seq-local: [w2467 _] -> [_ w2490]
              seq-local: [w2463 _] -> [_ w2486]
              tunnel: "Picture size" -> [w2484 _]
              tunnel: "Picture size 2" -> [w2483 _]
              tunnel: w2436 -> [w2482 _]
              tunnel: "X-Position" -> [w2481 _]
              tunnel: "Y-Position" -> [w2480 _]
              tunnel: "Z-Position" -> [w2479 _]
              tunnel: "Axis" -> [w2473 _]
              tunnel: "Resolution" -> [w2469 _]
              tunnel: [w2472 _] -> w2386
              tunnel: [_ w2500] -> w2405
              tunnel: w2404 -> [w2464 _]
              tunnel: w2379 -> [_ w2497]
              tunnel: "Laser  Profile" -> [_ w2496]
              tunnel: "Pixel time" -> [w2468 w2495]
              tunnel: w2401 -> [_ w2493]
              tunnel: [_ w2485] -> w2400
              tunnel: [_ w2489] -> w2399
              tunnel: [_ w2488] -> w2398
              tunnel: [_ w2487] -> w2390
              frame #0 {
                n1129 = call "PI_CheckScan.vi"("Picture size"=w2484, "Picture size 2"=w2483, "Axis"=w2473, "x-Position"=w2481, "y-Position"=w2480, "z-Position"=w2479, "error in (no error)"=w2464) -> ("error out"=w2463:errorcluster, "Picture size out"=w2470:dbl, "Picture size out 2"=w2471:dbl, "a0"=w2465:dbl, "b0"=w2466:dbl, "c0"=w2467:dbl)  [unwired: 7 in]
                n1130 = Bundle("a0"=w2465, "b0"=w2466, "c0"=w2467) -> (w2478:cluster{"a0":dbl, "b0":dbl, "c0":dbl})  [unwired: 1 in]
                n1131 = Divide(x=w2470, y=w2469) -> (x/y=w2476:dbl)
                n1132 = Divide(x=w2471, y=w2469) -> (x/y=w2477:dbl)
                n1133 = local write "Picture size"(w2470) -> ()
                n1134 = local write "Picture size 2"(w2471) -> ()
                n1135 = Round Toward +Infinity(x=w2476) -> (ceil(x): smallest int >= x=w2475:dbl)
                n1136 = Round Toward +Infinity(x=w2477) -> (ceil(x): smallest int >= x=w2474:dbl)
                n1137 = Bundle By Name(cluster=w2482, "Position"=w2478, "Axis 1 Pixels"=w2475, "Axis 2 Pixels"=w2474, "Axis"=w2473, "Resolution"=w2469, "PixelTime"=w2468) -> (w2472:T4)
              }
              frame #1 {
                n1138 = call "PI_AreaScan_Prepare_1.vi"("System"=w2493, "Laser"=w2496, "Axis"=w2497, "da"=w2499, "db"=w2498, "error in (no error)"=w2486, "a0"=w2492, "b0"=w2491, "Resolution"=w2494, "c0"=w2490, "Pixel time"=w2495) -> ("Tacq"=w2485:dbl, "lp"=w2488:i32, "ap"=w2489:i32, "Trigger"=w2487:dbl[], "error out"=w2500:errorcluster)  [unwired: 4 in]
                "Measure. time" <- w2485
              }
            }
            n1139 = control-ref of="WS File Tree"() -> (w2443:refnum<vi>)
            n1140 = local read "Workspace"() -> (w2448:path)
            n1141 = call "AOTF-Trigger_1.vi"("Channel"="Laser  Profile", "error in (no error)"=w2405, "Triggered"=TRUE, "lp"=w2398, "ap"=w2399) -> ("error out"=w2407:errorcluster)  [unwired: 2 in]
            n1142 = call "HH_Set.vi"("Device List"=w2459, "CFD Settings"="CFD Settings", "error in (no error)"=w2405, "SyncDiv"=8) -> ("ht3 header out"=w2419:T41, "Sync Rate"=w2417:i32, "error out"=w2389:errorcluster)  [unwired: 7 in, 2 out]
            n1143 = call "MTS_PreapareImage.vi"("WS File Tree"=w2443, "Workspace"=w2448, "Measurement Type"=w2397, "Image Measurent Parameters"=w2386, "error in"=w2389, "Trigger"=w2390) -> ("File Name (dup)"=w2432:path, "File No"=→"Last Image File No":i32, "Image Header"=w2434:T27, "Comment"=w2435:string, "error out"=w2388:errorcluster)  [unwired: 5 in]
            n1144 = local write "Active pt3"(w2432) -> ()
            n1145 = control-ref of="Image"() -> (w2421:refnum<vi>)
            n1146 = String To Byte Array(string="Laser  Profile") -> (unsigned byte array=w2381:u8[])
            n1147 = Unbundle By Name(w2386) -> ("Axis 1 Pixels"=w2414:dbl, "Axis 2 Pixels"=w2415:dbl, "Resolution"=w2412:dbl, "PixelTime"=w2394:dbl)  [unwired: 2 out]
            n1148 = Divide(x=1024, y=w2417) -> (x/y=w2396:dbl)
            n1149 = call "Scan_SetGraphScales.vi"("error in (no error)"=w2388, "Image Measurent Parameters"=w2386, "Image"=w2421) -> ("error out"=w2420:errorcluster)  [unwired: 8 in]
            n1150 = Initialize Array(0, 5, 2) -> (w2378:i32[][])
            n1151 = Subtract(x=w2381, y=48) -> (x-y=w2380:i32[])
            n1152 = Multiply(x=w2400, y=1000) -> (x*y=w2411:dbl)
            n1153 = Round Toward +Infinity(x=w2411) -> (ceil(x): smallest int >= x=w2409:dbl)
            n1154 = Divide(x=w2414, y=w2412) -> (x/y=w2423:dbl)
            n1155 = Divide(x=w2394, y=1000) -> (x/y=w2392:dbl)
            n1156 = Replace Array Subset(array=w2378, new element=w2380, index (col)=0) -> (w2376:i32[][])  [unwired: 1 in]
            n1157 = call "HT3_Create.vi"("Laser"=w2376, "Image Header in"=w2434, "Save pt3"="Save Files", "Measurement Type"=w2397, "error in"=w2420, "Comment"=w2435, "ht3 Header in"=w2419, "File Path"=w2432) -> ("error out"=w2449:errorcluster, "FileHeaderPos"=w2439:T42, "refnum out"=w2447:refnum<file>)  [unwired: 1 in]
            n1158 = Divide(x=w2415, y=w2412) -> (x/y=w2425:dbl)
            n1159 = Round Toward +Infinity(x=w2423) -> (ceil(x): smallest int >= x=w2422:dbl)
            n1160 = Round Toward +Infinity(x=w2425) -> (ceil(x): smallest int >= x=w2424:dbl)
            n1161 = call "HH_Start.vi"("Device Index"=w2427, "Acq. Time"=w2409, "error in (no error)"=w2449) -> ("error out"=w2456:errorcluster)  [unwired: 11 in, 1 out]
            n1162 = Initialize Array(0 ("element"), w2422, w2424) -> (w2393:i32[][])
            n1163 = Initialize Array(u32 0, w2440) -> (w2452:u32[])
            n1164 = Unbundle By Name(w2456) -> ("status"=w2457:bool)
            n1165 = Not(x=w2457) -> (.not. x?=w2455:bool)
            n1166 = case shown="True" w2455 {
              tunnel: [w2548 w2579] -> w2454
              tunnel: w2401 -> [_ w2574]
              tunnel: w2456 -> [w2549 w2575]
              tunnel: w2427 -> [w2547 w2566]
              tunnel: w2393 -> [_ w2551]
              tunnel: w2452 -> [_ w2573]
              tunnel: w2440 -> [_ w2572]
              tunnel: [w2546 w2571] -> w2451
              tunnel: [w2546 w2570] -> w2450
              tunnel: w2447 -> [w2545 w2569]
              tunnel: [w2545 w2568] -> w2446
              tunnel: [0 ("Num Records Total") w2567] -> w2445
              tunnel: [0.0 w2560] -> w2444
              tunnel: w2379 -> [_ w2563]
              tunnel: [dbl[] [] w2557] -> w2395
              tunnel: w2392 -> [_ w2553]
              tunnel: w2390 -> [_ w2552]
              frame False {
                (unwired) u64[] [] ("Histograms")
                w2546 = FALSE ("Stop Measurement")
                n1167 = call "HH_Stop.vi"("Device Index"=w2547, "error in (no error)"=w2549) -> ("error out"=w2548:errorcluster)  [unwired: 12 in, 1 out]
              }
              frame True {
                # "Overflow Interv. Time (s)"
                # "No Error"
                n1168 = call "PI Start WG.vi"("System no."=w2574, "axis"=w2563, "Generator"=T35."both axis", "Init DDL"=T36."none", "increment"=T36."slow axis", "error in"=w2575, "saved data"=T37."actual position") -> ("error out"=w2576:errorcluster)  [unwired: 12 in]
                n1169 = Initialize Array(0, 5) -> (w2554:i32[])
                n1170 = while {
                  tunnel: w2566 -> [w2599]
                  tunnel: w2573 -> [w2615]
                  tunnel: w2572 -> [w2614]
                  shift-right: [w2600] -> w2578
                  shift-left: w2576 -> [w2616]
                  shift-right: [FALSE ("Reset")] -> _
                  shift-left: TRUE ("Reset") -> [w2587]
                  tunnel: [w2608] -> w2571
                  tunnel: [w2604] -> w2570
                  tunnel: w2569 -> [w2606]
                  tunnel: [w2605] -> w2568
                  tunnel: [w2583] -> w2567
                  tunnel: [w2582] -> w2560
                  shift-right: [w2596] -> w2559
                  shift-left: w2554 -> [w2594]
                  tunnel: [w2593] -> w2558
                  tunnel: w2553 -> [w2590]
                  tunnel: w2552 -> [_]
                  shift-right: [w2581] -> w2550
                  shift-left: w2551 -> [w2589]
                  i -> [w2592]
                  stop <- w2613 stop-if-true
                  n1171 = call "HH_FIFORead.vi"("Device Index"=w2599, "Buffer In"=w2615, "Count"=w2614, "error in (no error)"=w2616) -> ("OK"=w2609:bool, "Buffer Out"=w2586:u32[], "Data Count"=w2585:i32, "FiFo Overrun"=w2608:bool, "error out"=w2607:errorcluster)  [unwired: 7 in]
                  n1172 = Wait (ms)(milliseconds to wait=u32 2) -> ()  [unwired: 1 out]
                  n1173 = local read "Global Stop"() -> (w2602:bool)
                  n1174 = local write "Buffer Overrun"(w2608) -> ()
                  n1175 = Unbundle(w2607) -> ("status"=w2612:bool)  [unwired: 2 out]
                  n1176 = call "HT3_Write.vi"("error in"=w2607, "Data Count"=w2585, "Data in"=w2586, "refnum in"=w2606) -> ("error out"=w2601:errorcluster, "refnum out"=w2605:refnum<file>)  [unwired: 6 in]
                  n1177 = local read "Stop Measurement"() -> (w2603:bool)
                  n1178 = call "GetCountRates.vi"("error in (no error)"=w2601, "DeviceIndex"=w2599) -> ("error out"=w2600:errorcluster, "CntRates"=w2598:dbl[], "SyncRate"=w2591:i32)  [unwired: 1 in]
                  n1179 = Multiply(x=w2590, y=w2591) -> (x*y=w2580:dbl)
                  n1180 = call "HH_ToImage.vi"("Data In"=w2586, "Reset"=w2587, "Image Array In"=w2589, "Data Count"=w2585, "Pixel Time (Laser Pulses)"=w2580) -> ("Image Array Out"=w2581:i32[][], "Histograms"=→"Histogram":i32[][], "Total Oveflow Count"=w2582:u64, "Num Records Total"=w2583:i64, "Traces"=→"Trace":i32[][])  [unwired: 4 in, 2 out]
                  n1181 = Insert Into Array(array=w2598, index=0, new element=w2591) -> (w2595:dbl[])
                  n1182 = Increment(x=w2592) -> (x+1=w2593:i32)
                  n1183 = Compound Arithmetic op=OR(invert w2609, w2612, w2602, w2603) -> (w2613:bool)
                  n1184 = Add(x=w2594, y=w2595) -> (x+y=w2596:dbl[])
                  n1185 = Or(x=w2603, y=w2602) -> (x .or. y?=w2604:bool)
                }
                "Image" <- w2550
                n1186 = Divide(x=w2559, y=w2558) -> (x/y=w2557:dbl[])
                n1187 = call "HH_Stop.vi"("Device Index"=w2566, "error in (no error)"=w2578) -> ("error out"=w2579:errorcluster)  [unwired: 12 in, 1 out]
              }
            }
            n1188 = flat-sequence {
              tunnel: w2454 -> [w2519]
              tunnel: [w2508] -> w2406
              tunnel: w2451 -> [w2521]
              tunnel: w2450 -> [w2510]
              tunnel: w2401 -> [w2518]
              tunnel: [w2517] -> w2373
              tunnel: w2446 -> [w2515]
              tunnel: w2445 -> [w2514]
              tunnel: w2444 -> [w2504]
              tunnel: w2439 -> [w2509]
              tunnel: w2396 -> [w2505]
              tunnel: w2395 -> [w2501]
              frame #0 {
                # "Count Rate (per s)"
                # "Finish after Aquire Image"
                n1189 = Or(x=w2510, y=w2521) -> (x .or. y?=w2520:bool)
                n1190 = Multiply(x=w2505, y=w2504) -> (x*y=w2503:dbl)
                n1191 = case shown="False" w2520 {
                  tunnel: w2519 -> [w2526 w2536]
                  tunnel: w2518 -> [w2524 w2537]
                  tunnel: [w2523 w2537] -> w2517
                  tunnel: [w2525 w2535] -> w2516
                  tunnel: [enum16{"timeover", "manual", "overflow"}."timeover" ("Stop Reason") w2540] -> w2511
                  tunnel: w2510 -> [w2522 w2538]
                  frame False {
                    # "Stop WaveGen\nif Aborted"
                    n1192 = case shown="True" w2522 {
                      tunnel: w2526 -> [w2528 w2533]
                      tunnel: [w2528 w2532] -> w2525
                      tunnel: w2524 -> [w2529 w2531]
                      tunnel: [w2529 w2531] -> w2523
                      frame False {
                      }
                      frame True {
                        n1193 = call "PI Write GPIB.vi"("System no."=w2531, "String to send"="0RT", "error in"=w2533) -> ("error out"=w2532:errorcluster)  [unwired: 16 in]
                      }
                    }
                  }
                  frame True {
                    n1194 = call "PI Write GPIB.vi"("System no."=w2537, "String to send"="0RT", "error in"=w2536) -> ("error out"=w2535:errorcluster)  [unwired: 16 in]
                    n1195 = Select(t=enum16{"timeover", "manual", "overflow"}."manual" ("Stop Reason"), s=w2538, f=enum16{"timeover", "manual", "overflow"}."overflow" ("Stop Reason")) -> (s? t:f=w2540:enum16{"timeover", "manual", "overflow"})
                  }
                }
                n1196 = Multiply(x=w2503, y=1000.0) -> (x*y=w2513:dbl)
                n1197 = To Long Integer(number=w2513) -> (32bit integer=w2512:i32)
                n1198 = property on="Aquire Image" class="Bool"("BoolText.Text"="Aquire Image" ("Caption.Text"), "BoolText.TextColor"=u32 0 ("Boolean Text.Colors:FG Color")) -> ()  [unwired: 2 in, 2 out]
                n1199 = call "HT3_Finish.vi"("FileHeaderPos"=w2509, "Rates"=w2501, "Stop Reason"=w2511, "error in"=w2516, "Num Records"=w2514, "Stop After (ms)"=w2512, "refnum in"=w2515) -> ("error out"=w2508:errorcluster)  [unwired: 4 in]
              }
            }
            n1200 = local read "X-Position"() -> (w2370:dbl)
            n1201 = local read "Y-Position"() -> (w2371:dbl)
            n1202 = local read "Z-Position"() -> (w2372:dbl)
            n1203 = call "PI Goto GPIB.vi"("System no."=w2373, "x-position"=w2370, "y-position"=w2371, "z-position"=w2372, "error in"=w2406) -> ("error out"=w2374:errorcluster)  [unwired: 14 in]
          }
          frame "Point Measurement" {
            w2641 = 0
            w2681 = 32768 ("dimension size")
            n1204 = local read "Workspace"() -> (w2714:path)
            n1205 = local read "X-Position"() -> (w2704:dbl)
            n1206 = local read "Y-Position"() -> (w2703:dbl)
            n1207 = local read "Z-Position"() -> (w2637:dbl)
            n1208 = local read "Laser  Profile"() -> (w2655:string)
            n1209 = Index Array(array=w2638) -> (element=w2727:T40)  [unwired: 1 in]
            n1210 = case shown="False" "Move into solution" {
              tunnel: [0.0 40.0] -> w2639
              frame False {
              }
              frame True {
              }
            }
            n1211 = Add(x=w2637, y=w2639) -> (x+y=w2636:dbl)
            n1212 = Equal?(x=w2697, y=T1."Auto Point" ("Task")) -> (x = y?=w2675:bool)
            n1213 = local read "Last Image File No"() -> (w2688:i32)
            n1214 = Bundle("X-Position"=w2704, "Y-Position"=w2703, w2636) -> (w2685:cluster{"X-Position":dbl, "Y-Position":dbl, dbl})  [unwired: 1 in]
            n1215 = Unbundle By Name(w2727) -> ("Dev"=w2698:i32)
            n1216 = Initialize Array(0, 5, 2) -> (w2649:i32[][])
            n1217 = call "AOTF-Trigger_1.vi"("Channel"=w2655, "Pulse length"=w2646, "Sync trigger ratio"=5, "error in (no error)"=w2667, "Triggered"=FALSE) -> ("error out"=w2668:errorcluster)  [unwired: 2 in]
            n1218 = call "MTS_AutoPointCords.vi"("Is Auto Point"=w2675, "Cords In"=w2685) -> ("Cords"=w2662:T43)  [unwired: 9 in]
            n1219 = Unbundle By Name(w2662) -> ("X-Position"=w2661:dbl, "Y-Position"=w2659:dbl, "Z-Position"=w2660:dbl)
            n1220 = call "PI Goto GPIB.vi"("System no."=w2630, "x-position"=w2661, "y-position"=w2659, "z-position"=w2660, "error in"=w2667) -> ("error out"=w2618:errorcluster)  [unwired: 14 in]
            n1221 = local read "CFD Settings"() -> (w2672:T3)
            n1222 = Select(t="Auto Measurement Time (ms)", s=w2675, f="Measurement Time") -> (s? t:f=w2679:i32)
            n1223 = Multiply(x=w2679, y=1000) -> (x*y=w2678:i32)
            n1224 = String To Byte Array(string=w2655) -> (unsigned byte array=w2653:u8[])
            n1225 = String Length(string=w2655) -> (length=w2645:i32)
            n1226 = And(x=w2675, y="Autopoint-Auto Z") -> (x .and. y?=w2682:bool)
            n1227 = Select(t=w2688, s=w2675, f=-1) -> (s? t:f=w2686:i32)
            n1228 = Select(t=T38."Auto Point" ("Measurement Type"), s=w2675, f=T38."Point Measurement" ("Measurement Type")) -> (s? t:f=w2691:T38)
            n1229 = Select(t="AutoPoint" ("Measurement Type"), s=w2675, f="Point" ("Measurement Type")) -> (s? t:f=w2624:string)
            n1230 = call "MTS_GenFileComment.vi"("Measurement Type"=w2691, "Parent File No"=w2686, "Info"=w2629, "Upper Left"=w2662, "error in"=w2716) -> ("Comment"=w2715:string, "error out"=w2713:errorcluster)  [unwired: 7 in, 2 out]
            n1231 = Subtract(x=w2653, y=48) -> (x-y=w2648:i32[])
            n1232 = local read "concatenated string"() -> (w2625:string)
            n1233 = Concatenate Strings(w2625, w2624) -> (w2623:string)
            n1234 = call "MTS_GetNextFileName.vi"("error in (no error)"=w2713, "File Type"="ht3", "Measurement Type"=w2623, "Workspace"=w2714) -> ("error out"=w2708:errorcluster, "Next File Name"=w2707:path)  [unwired: 6 in]
            n1235 = Replace Array Subset(array=w2649, new element=w2648, index (col)=w2641) -> (w2647:i32[][])  [unwired: 1 in]
            n1236 = Array Subset(array=w2646, index=w2641, length=w2645) -> (w2644:i32[])
            n1237 = Replace Array Subset(array=w2647, new element=w2644, index (col)=1) -> (w2643:i32[][])  [unwired: 1 in]
            n1238 = local read "PI SystemNumber"() -> (w2622:i32)
            n1239 = Not(x="Adjustment") -> (.not. x?=w2627:bool)
            n1240 = case shown="True" w2627 {
              tunnel: w2708 -> [w2730 w2738]
              tunnel: w2707 -> [_ w2737]
              tunnel: [w2730 w2736] -> w2706
              tunnel: [path "D:/tmp.ht3" w2731] -> w2705
              tunnel: w2691 -> [_ w2733]
              tunnel: w2686 -> [_ w2735]
              tunnel: w2684 -> [_ w2732]
              frame False {
              }
              frame True {
                n1241 = call "MTS_AddFileToWorkspace.vi"("File Name"=w2737, "File Type"=T18."pt3 File", "Measurement Type"=w2733, "error in (no error)"=w2738, "Parent"=w2735, "Tree Refnum"=w2732) -> ("File Name (dup)"=w2731:path, "error out"=w2736:errorcluster)  [unwired: 7 in, 1 out]
              }
            }
            n1242 = And(x="Auto Shutter Control", y=w2675) -> ()  [unwired: 1 out]
            n1243 = Initialize Array(u32 0, w2681) -> (w2720:u32[])
            n1244 = call "PI Pos GPIB.vi"("System no."=w2622, "error in"=w2618) -> ("x-position"=w2621:dbl, "y-position"=w2620:dbl, "z-position"=w2619:dbl, "error out"=w2617:errorcluster)  [unwired: 14 in]
            n1245 = call "HH_Set.vi"("Device List"=w2638, "CFD Settings"=w2672, "error in (no error)"=w2617) -> ("ht3 header out"=w2702:T41, "Sync Rate"=w2656:i32, "error out"=w2700:errorcluster)  [unwired: 8 in, 2 out]
            n1246 = Bundle By Name(cluster=w2702, "AcquisitionTime (ms)"=w2678) -> (w2701:T41)
            n1247 = Divide(x=65536 ("n"), y=w2656) -> (x/y=w2657:dbl)
            n1248 = case shown="False" w2682 {
              tunnel: w2700 -> [w2741 w2748]
              tunnel: [w2741 w2747] -> w2699
              tunnel: w2698 -> [_ w2746]
              tunnel: w2657 -> [_ w2745]
              tunnel: w2662 -> [_ w2744]
              frame False {
              }
              frame True {
                # "Auto Z"
                n1249 = call "MTS_AutoZPos.vi"("PH Dev"=w2746, "OFlow Interv [s]"=w2745, "error in"=w2748, "Start Point"=w2744) -> ("New Z"=w2743:dbl, "Counts"=→"Counts":u32[], "error out"=w2747:errorcluster)  [unwired: 9 in]
                n1250 = local write "Z-Position"(w2743) -> ()
              }
            }
            n1251 = call "HT3_Create.vi"("Laser"=w2643, "Save pt3"=w2627, "error in"=w2699, "Comment"=w2715, "ht3 Header in"=w2701, "File Path"=w2705) -> ("error out"=w2717:errorcluster, "FileHeaderPos"=w2680:T42, "refnum out"=w2711:refnum<file>)  [unwired: 3 in]
            n1252 = call "HH_Start.vi"("Device Index"=w2698, "Acq. Time"=w2678, "error in (no error)"=w2717) -> ("error out"=w2669:errorcluster)  [unwired: 11 in, 1 out]
            n1253 = Unbundle By Name(w2669) -> ("status"=w2726:bool)
            n1254 = Not(x=w2726) -> (.not. x?=w2725:bool)
            n1255 = case shown="True" w2725 {
              tunnel: [w2783 w2806] -> w2723
              tunnel: w2669 -> [w2784 w2794]
              tunnel: w2706 -> [w2785 w2805]
              tunnel: [w2785 w2804] -> w2724
              tunnel: w2698 -> [w2778 w2793]
              tunnel: w2720 -> [_ w2801]
              tunnel: w2681 -> [_ w2800]
              tunnel: [w2782 w2799] -> w2719
              tunnel: [w2782 w2798] -> w2718
              tunnel: w2711 -> [w2781 w2797]
              tunnel: [w2781 w2796] -> w2710
              tunnel: [i64 0 ("Num Records Total") w2795] -> w2709
              tunnel: [dbl[] [] w2790] -> w2664
              tunnel: [0 w2789] -> w2663
              frame False {
                (unwired) 0.0
                w2782 = FALSE ("Stop Measurement")
                n1256 = call "HH_Stop.vi"("Device Index"=w2778, "error in (no error)"=w2784) -> ("error out"=w2783:errorcluster)  [unwired: 12 in, 1 out]
              }
              frame True {
                # "Overflow Interv. Time (s)"
                # "No Error"
                n1257 = Initialize Array(0, 5) -> (w2788:i32[])
                n1258 = while {
                  tunnel: w2793 -> [w2815]
                  tunnel: w2801 -> [w2839]
                  tunnel: w2800 -> [w2838]
                  shift-right: [w2816] -> w2803
                  shift-left: w2794 -> [w2840]
                  shift-right: [w2837] -> w2804
                  shift-left: w2805 -> [w2837]
                  shift-right: [FALSE ("Reset")] -> _
                  shift-left: TRUE ("Reset") -> [w2833]
                  tunnel: [w2830] -> w2799
                  tunnel: [w2822] -> w2798
                  tunnel: w2797 -> [w2826]
                  tunnel: [w2825] -> w2796
                  tunnel: [w2824] -> w2795
                  tunnel: [w2823] -> w2789
                  shift-right: [w2810] -> w2791
                  shift-left: w2788 -> [w2809]
                  tunnel: [w2807] -> w2792
                  i -> [w2808]
                  stop <- w2836 stop-if-true
                  n1259 = call "HH_FIFORead.vi"("Device Index"=w2815, "Buffer In"=w2839, "Count"=w2838, "error in (no error)"=w2840) -> ("OK"=w2831:bool, "Buffer Out"=w2827:u32[], "Data Count"=w2828:i32, "FiFo Overrun"=w2830:bool, "error out"=w2829:errorcluster)  [unwired: 7 in]
                  n1260 = Wait (ms)(milliseconds to wait=u32 10) -> ()  [unwired: 1 out]
                  n1261 = local write "Buffer Overrun"(w2830) -> ()
                  n1262 = local read "Global Stop"() -> (w2820:bool)
                  n1263 = Unbundle(w2829) -> ("status"=w2835:bool)  [unwired: 2 out]
                  n1264 = call "HH_TraceAndHisto.vi"("Data In"=w2827, "Reset"=w2833, "Data Count"=w2828) -> ("Histograms"=w2819:i32[][], "Total Oveflow Count"=w2823:u64, "Num Records Total"=w2824:i64, "Traces"=w2818:i32[][])  [unwired: 8 in, 1 out]
                  n1265 = call "HT3_Write.vi"("error in"=w2829, "Data Count"=w2828, "Data in"=w2827, "refnum in"=w2826) -> ("error out"=w2817:errorcluster, "refnum out"=w2825:refnum<file>)  [unwired: 6 in]
                  n1266 = local read "Stop Measurement"() -> (w2821:bool)
                  n1267 = local write "Histogram"(w2819) -> ()
                  n1268 = local write "Trace"(w2818) -> ()
                  n1269 = call "GetCountRates.vi"("error in (no error)"=w2817, "DeviceIndex"=w2815) -> ("error out"=w2816:errorcluster, "CntRates"=w2811:dbl[], "SyncRate"=w2812:i32)  [unwired: 1 in]
                  n1270 = Insert Into Array(array=w2811, index=0, new element=w2812) -> (w2813:dbl[])
                  n1271 = Compound Arithmetic op=OR(invert w2831, w2835, w2820, w2821) -> (w2836:bool)
                  n1272 = Or(x=w2821, y=w2820) -> (x .or. y?=w2822:bool)
                  n1273 = Increment(x=w2808) -> (x+1=w2807:i32)
                  n1274 = Add(x=w2809, y=w2813) -> (x+y=w2810:dbl[])
                }
                n1275 = Divide(x=w2791, y=w2792) -> (x/y=w2790:dbl[])
                n1276 = call "HH_Stop.vi"("Device Index"=w2793, "error in (no error)"=w2803) -> ("error out"=w2806:errorcluster)  [unwired: 12 in, 1 out]
              }
            }
            n1277 = property on="Z out" class="DigNum (strict)"("Value"=w2619) -> ()  [unwired: 2 in, 2 out]
            n1278 = property on="X out" class="DigNum (strict)"("Value"=w2621) -> ()  [unwired: 2 in, 2 out]
            n1279 = property on="Y out" class="DigNum (strict)"("Value"=w2620) -> ()  [unwired: 2 in, 2 out]
            n1280 = flat-sequence {
              tunnel: w2724 -> [w2769]
              tunnel: w2723 -> [w2765]
              tunnel: [w2769] -> w2722
              tunnel: [w2762] -> w2635
              tunnel: w2719 -> [w2767]
              tunnel: w2718 -> [w2758]
              tunnel: w2710 -> [w2761]
              tunnel: w2709 -> [w2760]
              tunnel: w2680 -> [w2757]
              tunnel: w2664 -> [w2754]
              tunnel: w2663 -> [w2753]
              frame #0 {
                # "Finish after Measurement"
                n1281 = Index Array(array=w2754, index=0) -> (element=w2755:dbl)
                n1282 = Or(x=w2758, y=w2767) -> (x .or. y?=w2766:bool)
                n1283 = Divide(x=w2753, y=w2755) -> (x/y=w2752:dbl)
                n1284 = case shown="False" w2766 {
                  tunnel: w2765 -> [w2771 w2772]
                  tunnel: [w2771 w2772] -> w2763
                  tunnel: [enum16{"timeover", "manual", "overflow"}."timeover" ("Stop Reason") w2775] -> w2759
                  tunnel: w2758 -> [_ w2773]
                  frame False {
                  }
                  frame True {
                    n1285 = Select(t=enum16{"timeover", "manual", "overflow"}."manual" ("Stop Reason"), s=w2773, f=enum16{"timeover", "manual", "overflow"}."overflow" ("Stop Reason")) -> (s? t:f=w2775:enum16{"timeover", "manual", "overflow"})
                  }
                }
                n1286 = Multiply(x=1024000, y=w2752) -> (x*y=w2750:dbl)
                n1287 = To Long Integer(number=w2750) -> (32bit integer=w2749:i32)
                n1288 = property on="Point Measurement" class="Bool"("BoolText.Text"="Point Measurement" ("Caption.Text"), "BoolText.TextColor"=u32 0 ("Boolean Text.Colors:FG Color")) -> ()  [unwired: 2 in, 2 out]
                n1289 = call "HT3_Finish.vi"("FileHeaderPos"=w2757, "Rates"=w2754, "Stop Reason"=w2759, "error in"=w2763, "Num Records"=w2760, "Stop After (ms)"=w2749, "refnum in"=w2761) -> ("error out"=w2762:errorcluster)  [unwired: 4 in]
              }
            }
            n1290 = local read "Auto Shutter Control"() -> (w2674:bool)
            n1291 = And(x=w2675, y=w2674) -> (x .and. y?=w2673:bool)
            n1292 = Select(t=T14."Auto Measurement Control" ("Do Measurement"), s=w2675, f=T14."No Measurement" ("Do Measurement")) -> (s? t:f=w2696:T14)
            n1293 = local read "X-Position"() -> (w2633:dbl)
            n1294 = local read "Y-Position"() -> (w2631:dbl)
            n1295 = local read "Z-Position"() -> (w2632:dbl)
            n1296 = call "PI Goto GPIB.vi"("System no."=w2630, "x-position"=w2633, "y-position"=w2631, "z-position"=w2632, "error in"=w2635) -> ("error out"=w2634:errorcluster)  [unwired: 14 in]
          }
          frame "Save Color Image" {
            n1297 = local read "Active pt3"() -> (w2849:path)
            n1298 = call "MTS_GetFileFromWS.vi"(".pt3 File Name"=w2849) -> ("File Header"=w2848:T24)  [unwired: 9 in, 1 out]
            n1299 = Unbundle By Name(w2848) -> ("Measurement Type"=w2847:T25, "Pixels"=w2844:i32[])
            n1300 = Equal?(x=T38."Image File" ("Measurement Type"), y=w2847) -> (x = y?=w2845:bool)
            n1301 = control-ref of="WS File Tree"() -> (w2850:refnum<vi>)
            n1302 = case shown="True" w2845 {
              tunnel: w2854 -> [w2855 w2878]
              tunnel: w2849 -> [_ w2877]
              tunnel: w2849 -> [_ _]
              tunnel: [w2855 w2857] -> w2841
              tunnel: w2850 -> [_ _]
              tunnel: w2844 -> [_ w2862]
              frame False {
              }
              frame True {
                # "Image Intensity Array"
                # "Image Intensity Array"
                n1303 = call "HT3_Open.vi"("error in"=w2878, "File Path"=w2877) -> ("error out"=w2870:errorcluster, "Header"=w2874:T26, "refnum out"=w2876:refnum<file>)  [unwired: 3 in, 4 out]
                n1304 = Index Array(array=w2862, index #2=1 ("index")) -> (element #1=w2859:i32, element #2=w2860:i32)  [unwired: 1 in]
                n1305 = Unbundle By Name(w2874) -> ()  [unwired: 15 out]
                n1306 = Initialize Array(0 ("element"), w2859, w2860) -> (w2872:i32[][])
                n1307 = while {
                  tunnel: w2876 -> [w2903]
                  shift-right: [FALSE ("Start From Top")] -> _
                  shift-left: TRUE ("Start From Top") -> [w2897]
                  shift-right: [w2896] -> w2869
                  shift-left: w2870 -> [w2894]
                  tunnel: [w2895] -> w2868
                  tunnel: w2872 -> [w2893]
                  tunnel: [w2892] -> w2871
                  tunnel: [w2893] -> _
                  stop <- w2900 stop-if-true
                  n1308 = call "HT3_Read.vi"("Start From Top"=w2897, "error in"=w2894, "Data count"=10000, "refnum in"=w2903) -> ("error out"=w2896:errorcluster, "Data out"=w2899:u32[], "refnum out"=w2895:refnum<file>, "EOF?"=w2900:bool)  [unwired: 4 in]
                  n1309 = Array Size(array=w2899) -> (size(s)=w2898:i32)
                  n1310 = call "HH_FileToImage_1.vi"("Data In"=w2899, "Reset"=w2897, "Data Count"=w2898) -> ("Histograms"=w2892:i32[][])  [unwired: 7 in, 5 out]
                }
                n1311 = call "MTS_SelectTCSPCBinning.vi"("Histograms in"=w2871) -> ("TCSPC Binning"=w2864:i32[][])  [unwired: 1 in, 9 out]
                n1312 = Initialize Array(0 ("element"), 4 ("dimension size"), w2859, w2860) -> (w2865:i32[][][])
                n1313 = while {
                  tunnel: w2868 -> [w2891]
                  shift-right: [FALSE ("Start From Top")] -> _
                  shift-left: TRUE ("Start From Top") -> [w2885]
                  shift-right: [w2884] -> w2856
                  shift-left: w2869 -> [w2880]
                  tunnel: [w2883] -> w2858
                  tunnel: w2865 -> [w2882]
                  tunnel: [w2881] -> _
                  tunnel: w2864 -> [w2879]
                  stop <- w2888 stop-if-true
                  n1314 = call "HT3_Read.vi"("Start From Top"=w2885, "error in"=w2880, "Data count"=10000, "refnum in"=w2891) -> ("error out"=w2884:errorcluster, "Data out"=w2887:u32[], "refnum out"=w2883:refnum<file>, "EOF?"=w2888:bool)  [unwired: 4 out]
                  n1315 = Array Size(array=w2887) -> (size(s)=w2886:i32)
                  n1316 = call "HH_ToColorImage.vi"("Data In"=w2887, "Reset"=w2885, "Image Array In"=w2882, "Data Count"=w2886, "TCSPC Binning"=w2879) -> ("Image Array Out"=w2881:i32[][][])  [unwired: 2 in, 8 out]
                }
                n1317 = Close File(refnum=w2858, error in=w2856) -> (error out=w2857:errorcluster)  [unwired: 1 out]
              }
            }
          }
        }
      }
      frame Error {
      }
    }
    n1318 = flat-sequence {
      tunnel: w2330 -> [w2922]
      tunnel: [w2922] -> w2329
      tunnel: w2325 -> [w2918]
      tunnel: w2323 -> [_]
      frame #0 {
        n1319 = control-ref of="ShowTab"() -> (w2921:refnum<vi>)
        n1320 = Equal?(x=w2918, y=T14."No Measurement" ("Do Measurement")) -> (x = y?=w2919:bool)
        n1321 = Not(x=w2919) -> (.not. x?=w2920:bool)
        n1322 = case shown="True" w2919 {
          tunnel: w2921 -> [_ w2923]
          frame False {
          }
          frame True {
            n1323 = call "MTS_ShowHideTabs.vi"("Action"=enum16{"Show All", "Hide Tab", "Show Tab"}."Show All", "ShowTab"=w2923) -> ()  [unwired: 8 in, 2 out]
          }
        }
        n1324 = local write "Running"(w2920) -> ()
        n1325 = local write "Task"(w2918) -> ()
      }
    }
    n1326 = Unbundle(w2327) -> ("status"=w2326:bool)  [unwired: 2 out]
    n1327 = local read "Global Stop"() -> (w2333:bool)
    n1328 = Compound Arithmetic op=OR(w2326, w2331, w2333) -> (w2332:bool)
  }
  n1329 = Divide(x=w20, y=w18) -> (x/y=w19:dbl)
  n1330 = Divide(x=32767.0 ("Maximum Voltage"), y=3276.8) -> (x/y=w15:dbl)
  n1331 = flat-sequence {
    tunnel: w44 -> [w2925]
    tunnel: [w2925] -> w43
    frame #0 {
      n1332 = local write "Global Stop"(TRUE ("Global Stop")) -> ()
    }
  }
  n1333 = call <userlib>:"Close connection if open.vi"("System no."=w47, "error in"=w43) -> ("error out"=w30:errorcluster)  [unwired: 16 in, 1 out]
  n1334 = Merge Errors(w33, w32, w30, w31, w41, w29) -> (w46:errorcluster)
  n1335 = call <vilib>:"Simple Error Handler.vi"("error in (no error)"=w46) -> ("error out"=→"error out":errorcluster)  [unwired: 4 in, 4 out]
